vi "MC_8_10_12a_PD.vi"() -> ()   [LabVIEW 2011]
uses:
  <vilib>/Utility/file.llb/Read From Spreadsheet File (string).vi
  <vilib>/Utility/inputDevices.llb/keyboardAcquire.vi
  <vilib>/Utility/file.llb/Write To Spreadsheet File (DBL).vi
  <vilib>/Utility/file.llb/Write To Spreadsheet File (string).vi
  <vilib>/regexp/Match Regular Expression.xnode
panel:
  out "Opj X Axis":string
  in  "Room Temp":dbl=294.0
  out "No Image 2":path=path "\\\\acad1\\physics/Jurchescu-group/JW-PD/Image Not Found.png"
  out "Save1 Array":string[][](array[string])
  out "Lin Vd":dbl
  out "Lin-Vg Array-Used":dbl[](array[numeric])
  out "Lin Id-Used":dbl[](array[numeric])
  out "Comments":string
  out "Folder Index":dbl caption="Length"
  out "Current \nRecord":string[](array[string])
  out "Transformer \nHeaders":string[](array[string])
  out "Current Device ID":string
  out "Column":string
  out "Row":string
  out "Rec: Concentration":dbl
  out "Rec: Solvent":string
  out "Rec: Method":string
  in  "?":T1(tab)
  in  "Transport File":path
  out "Transport Folder":path
  out "Rec: Material":string
  in  "Treatment Concentration (mM):":dbl=nan
  in  "Surface Treatment:":string="NaN"
  in  "# Drops*:":dbl=inf
  in  "Solution Temp (C):":dbl=nan
  in  "Relative Humidity (%):":dbl=nan
  in  "Room Temp (F):":dbl=nan
  in  "Time (s):":dbl=nan
  out "Accel (RPM/s):":dbl
  in  "RPM:":dbl=nan
  in  "Wait Time (s):":dbl=nan
  in  "Sample #:":dbl=1.0
  in  "Fabricator:":string="NaN"
  in  "Transfer File":path
  out "Transfer Folder":path
  in  "Image Folder":path
  out "Image File":path=path "D:/UserData/Desktop/Jeremy/WFU/Research/Programs/VI mods/Image Not Found.png"
  in  "Ramp (s):":dbl=3.0
  out "Calc: On/Off":dbl caption="On/Off-Sat" format="%#.2e"
  out "Calc: Off I-Sat":dbl caption="Off I-Sat" format="%#.2e"
  in  "Manuel-Dielectric":bool
  in  "Manuel-Length":bool
  out "Calc: VT-Lin":dbl
  out "New: VT-Lin":dbl
  out "Rec: VT-Lin":dbl caption="VT-Lin" format="%#_3g"
  out "Calc: Trap Density-STS":dbl format="%#.2e"
  out "New: Trap Density-STS":dbl format="%#.2e"
  out "Rec: Trap Density-STS":dbl caption="N-Sat (STS)" format="%#.2e"
  out "Calc: Trap Density-VT":dbl format="%#.2e"
  out "New: Trap Density-VT":dbl format="%#.2e"
  out "Rec: Trap Density-VT":dbl caption="N-Sat (VT)" format="%#.2e"
  out "Calc: Mobility-Lin":dbl format="%#.2e"
  out "New: Mobility-Lin":dbl format="%#_4e"
  out "Rec: Mobility-Lin":dbl caption="Mobility-Lin" format="%#_3e"
  out "Calc: Mobility-Sat":dbl format="%#.2e"
  out "Rec: Length":dbl caption="Length" format="%#_3g"
  out "Rec: Width":dbl caption="Width" format="%#_4g"
  out "Rec: Dielectric (d)":dbl caption="Dielectric (d)" format="%#_3g"
  in  "Cancel Button":bool
  in  "Up Button":bool
  in  "Down Button":bool
  out "Data Name:":string
  in  "Save Changes?":bool
  in  "New: Dielectric":dbl
  in  "New: Length":dbl
  in  "New: Width":dbl
  out "New: Mobility-Sat":dbl format="%#.2e"
  in  "Blank Button":bool
  in  "Zoom":i16(slide)=-3 scale=-5.0..5.0
  out "Image Out 2":T2(plugin-control)
  out "Image Out":T2(plugin-control)
  in  "Magnification":u16(ring) items=["5x", "10x", "20x", "50x", "80x"]
  out "Total Width":dbl
  out "Distances":dbl[](array[numeric])
  in  "Undo Button":bool
  in  "Remove Button":bool
  out "Rec: Mobility-Sat":dbl caption="Mobility-Sat" format="%#.2e"
  out "Index":string
  out "Image Name":string
  in  "Export":bool
  out "Calc: VT-Sat":dbl format="%#.2g"
  out "New: VT-Sat":dbl format="%#.2g"
  in  "Manual-Width":bool caption="Manual"
  out "Calc: STS":dbl format="%#.2g"
  out "New: STS":dbl format="%#.2g"
  out "Rec: VT-Sat":dbl caption="VT-Sat" format="%#.2g"
  out "Rec: STS":dbl caption="STS-Sat" format="%#.2g"
  out "Rec: On/Off":dbl caption="On/Off-Sat" format="%#.2e"
  in  "Save Changes? 2":bool
  in  "Save Changes? 3":bool
  out "Date Recorded":string="Date Recorded" caption="Measured"
  out "Date Created":string caption="Fabricated"
  out "Rec: Temp":dbl caption="Sample Temp" format="%.1f"
  in  "New: Temp":dbl format="%.1f"
  out "Rec: Off I-Sat":dbl caption="Off I-Sat" format="%#.2e"
  in  "Independant Variable":string(combo)="Length (um):"
  in  "Transfer Plots":enum32{"Linear", "Saturation"}(tab)=enum."Saturation"
  out "XY Graph-Lin":cluster{dbl[], dbl[]}[](graph)
  in  "Slide":dbl(slide) step=1.0 scale=-22.0..89.0 scale format="%#_1p"
  out "XY Graph":cluster{dbl[], dbl[]}[](graph)
  in  "Previous Button":bool
  in  "Next Button":bool
  in  "NumPts":dbl=5.0
  in  "Log Plots":enum32{"Linear", "Saturation"}(tab)=enum."Saturation"
  in  "Slide 2":dbl(slide) step=1.0 scale=-1.0..82.0 scale format="%#_1p"
  out "XY Graph 2":cluster{dbl[], dbl[]}[](graph)
  in  "Previous Button 2":bool
  in  "Next Button 2":bool
  in  "NumPts 2":dbl=5.0 caption="NumPts"
  in  "Manual-Temp":bool caption="Manual"
  in  "Origin Project File":path=path "\\\\acad1\\physics/Jurchescu-group/JW-PD/Group Library/Origin Project Files/DeviceData_8_10_12a_JW.opj"
  in  "No Image File":path=path "\\\\acad1\\physics/Jurchescu-group/JW-PD/Mega Awesome/Image Not Found.png"
  out "String":string
  out "Index 2":dbl
  out "Sat Id-Log-Used":dbl[](array[numeric])
  out "Vg Array-Log-Used":dbl[](array[numeric])
  out "ROI Descriptor out":T3 {"Contours"."Type" items=["No Selection", "Point", "Line", "Rectangle", "Oval", "Polygon", "Freehand Region", "Annulus", "Unused2", "Unused3", "Broken Line", "Freehand Line", "Rotated Rectangle"]}
  out "ROI Descriptor":T3 {"Contours"."Type" items=["No Selection", "Point", "Line", "Rectangle", "Oval", "Polygon", "Freehand Region", "Annulus", "Unused2", "Unused3", "Broken Line", "Freehand Line", "Rotated Rectangle"]}
  out "Numeric 3":dbl
  out "Array 6":dbl[][](array[numeric])
  out "Cluster":T4
  out "Array 5":dbl[](array[numeric])
  out "Array 4":dbl[](array[numeric])
  out "Array 3":dbl[](array[numeric])
  out "Numeric 2":dbl
  out "Numeric":dbl
  out "Sat Id-Used":dbl[](array[numeric])
  out "Sat Vg Array-Used":dbl[](array[numeric])
  out "MobVi Index":dbl
  in  "Row Start":dbl=20.0
  # "Data Locations"
  # "Transport Location"
  # "Transfer Location"
  # "Image Location"
  # "Sample Properties"
  # "*     Inf = Full coverage\n   NaN = Unknown or Not Applicable"
  # "Recorded"
  # "Calculated"
  # "Re-Calculated"
  # "Manual"
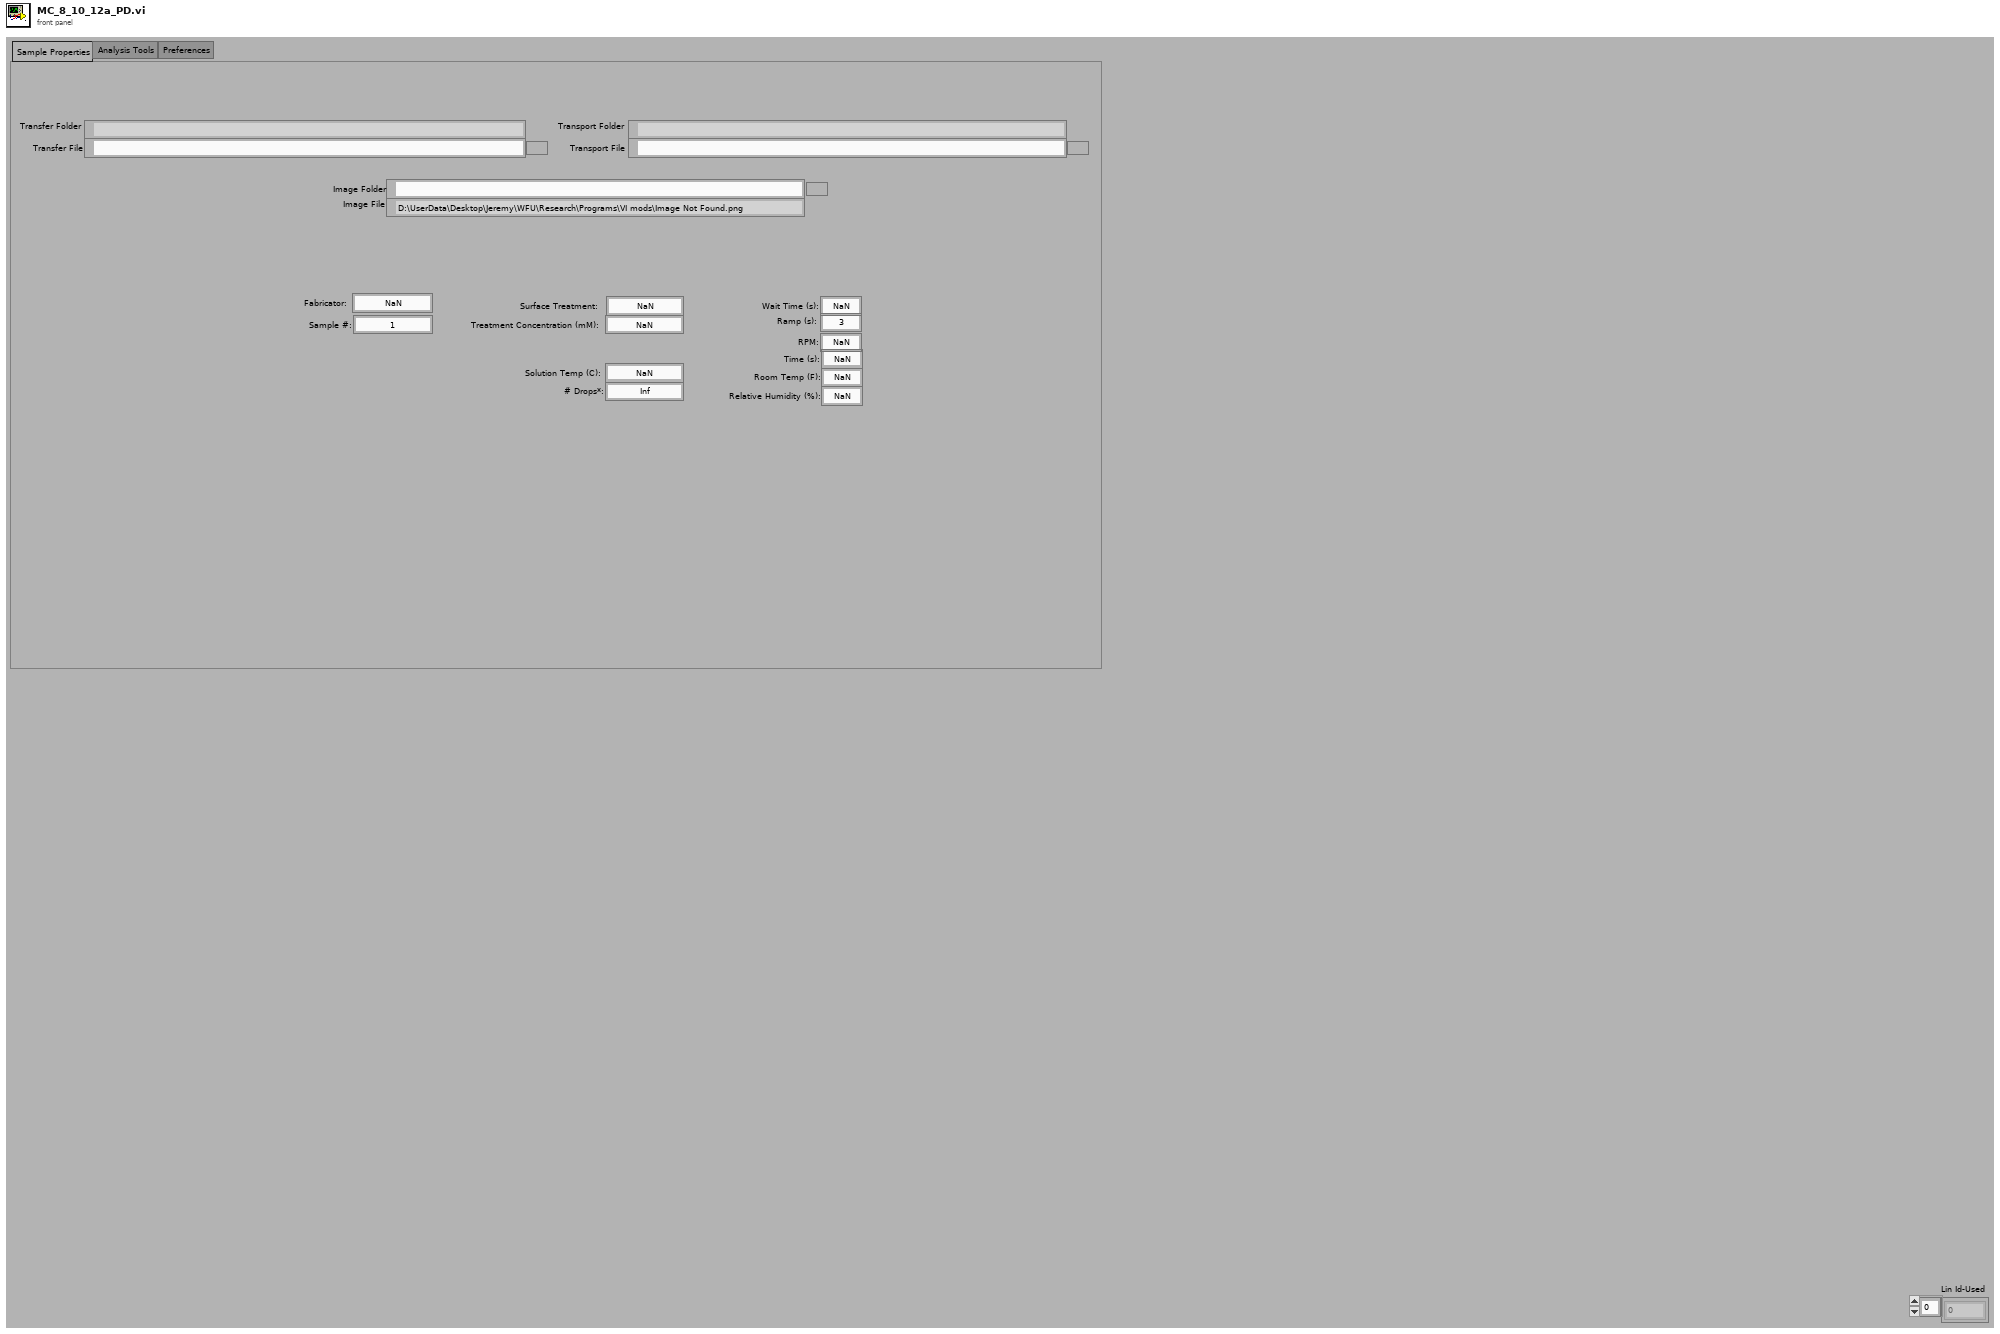
[diagram p1: front panel]
types:
  T1 = enum32{"Sample Properties", "Analysis Tools", "Preferences", "Current Database"}
  T2 = typedef "IMAQ Image.ctl" = refnum<image>
  T3 = typedef "ROI Descriptor" = cluster{"Global Rectangle":i32[], "Contours":cluster{"ID":enum32{"External", "Internal"}, "Type":u32, "Coordinates":i32[]}[]}
  T4 = cluster{"Numeric":dbl, "Numeric 2":dbl, "Numeric 3":dbl, "Numeric 4":dbl}
  T5 = cluster{"Mobility-Sat":dbl, "Moblitity-Lin":dbl, "On/Off":dbl, "Off Current":dbl, "Vt-Sat":dbl, "STS":dbl, "Trap Density-VT":dbl, "Trap Density-STS":dbl}
  T6 = cluster{"Date Recorded":string, "Index":string, "Length":dbl, "Width":dbl, "Sample Temp":dbl}
  T7 = cluster{"Date Created":string, "Material":string, "Solvent":string, "Concentration":dbl, "Method":string, "Dielectric (nm)":dbl, "Treatment":string, "Comments":string}
  T8 = cluster{"Mobility-Sat":dbl, "Vt-Sat":dbl, "Mobility-Lin":dbl, "Vt-Lin":dbl, "Off I-Sat":dbl, "On/Off I-Sat":dbl}
  T9 = cluster{"[0]":cluster{dbl[], dbl[]}, "[1]":cluster{dbl[], dbl[]}, "[2]":cluster{dbl[], dbl[]}, "[3]":cluster{dbl[], dbl[]}, "[4]":cluster{dbl[], dbl[]}, "[5]":cluster{dbl[], dbl[]}, "[6]":cluster{dbl[], dbl[]}, "[7]":cluster{dbl[], dbl[]}, "[8]":cluster{dbl[], dbl[]}}
  T10 = cluster{"Global Rectangle":i32[], "Contours":cluster{"Contour Type":u32, "ROI Type":u32, "Points":i32[]}[]}
  T11 = typedef "LVBoundsTypeDef.ctl" = cluster{"Width":u32, "Height":u32}
  T12 = enum16{"0", "1", "2", "3", "4", "5", "6", "7", "8", "9", "A", "B", "C", "D", "E", "F", "G", "H", "I", "J", "K", "L", "M", "N", "O", "P", "Q", "R", "S", "T", "U", "V", "W", "X", "Y", "Z", "F1", "F2", "F3", "F4", "F5", "F6", "F7", "F8", "F9", "F10", "F11", "F12", "F13", "F14", "F15", "ADD", "BACK", "BACKSLASH", "CAPITAL", "COMMA", "DECIMAL", "DELETE", "DIVIDE", "DOWN", "END", "EQUALS", "ESCAPE", "GRAVE (`)", "HOME", "INSERT", "LBRACKET", "LCONTROL", "LEFT", "L ALT", "LSHIFT", "LWIN", "MINUS", "MULTIPLY", "NEXT", "NUMLOCK", "NUMPAD_0", "NUMPAD_1", "NUMPAD_2", "NUMPAD_3", "NUMPAD_4", "NUMPAD_5", "NUMPAD_6", "NUMPAD_7", "NUMPAD_8", "NUMPAD_9", "PAUSE", "PERIOD", "PRIOR (PG UP)", "RBRACKET", "RCONTROL", "RETURN", "RIGHT", "R ALT", "RSHIFT", "RWIN", "SCROLL", "SEMICOLON", "SLASH", "SPACE", "SUBTRACT", "TAB", "UP", "ENTER (num pad)", "' (quote)"}[]
  T13 = enum16{"0", "1", "2", "3", "4", "5", "6", "7", "8", "9", "A", "B", "C", "D", "E", "F", "G", "H", "I", "J", "K", "L", "M", "N", "O", "P", "Q", "R", "S", "T", "U", "V", "W", "X", "Y", "Z", "F1", "F2", "F3", "F4", "F5", "F6", "F7", "F8", "F9", "F10", "F11", "F12", "F13", "F14", "F15", "ADD", "BACK", "BACKSLASH", "CAPITAL", "COMMA", "DECIMAL", "DELETE", "DIVIDE", "DOWN", "END", "EQUALS", "ESCAPE", "GRAVE (`)", "HOME", "INSERT", "LBRACKET", "LCONTROL", "LEFT", "L ALT", "LSHIFT", "LWIN", "MINUS", "MULTIPLY", "NEXT", "NUMLOCK", "NUMPAD_0", "NUMPAD_1", "NUMPAD_2", "NUMPAD_3", "NUMPAD_4", "NUMPAD_5", "NUMPAD_6", "NUMPAD_7", "NUMPAD_8", "NUMPAD_9", "PAUSE", "PERIOD", "PRIOR (PG UP)", "RBRACKET", "RCONTROL", "RETURN", "RIGHT", "R ALT", "RSHIFT", "RWIN", "SCROLL", "SEMICOLON", "SLASH", "SPACE", "SUBTRACT", "TAB", "UP", "ENTER (num pad)", "' (quote)"}
  T14 = cluster{"Contour Type":u32, "ROI Type":u32, "Points":i32[]}[]
  T15 = cluster{i32[], cluster{"Contour Type":u32, "ROI Type":u32, "Points":i32[]}[]}
  T16 = cluster{"Independant  Variable Indicator":string, "Parameter String Indicator":string}
  T17 = cluster{string, sgl, bool, bool, bool, bool, bool, bool, i32}
  T18 = cluster{i32, cluster{string, sgl, bool, bool, bool, bool, bool, bool, i32}, i32, i32}
  T19 = cluster{"Contour Type":u32, "ROI Type":u32, "Points":i32[]}
  T20 = cluster{"Points[0]":i32, "Points[1]":i32, "Points[2]":i32, "Points[3]":i32, "Points[4]":i32, "Points[5]":i32, "Points[6]":i32, "Points[7]":i32, "Points[8]":i32}
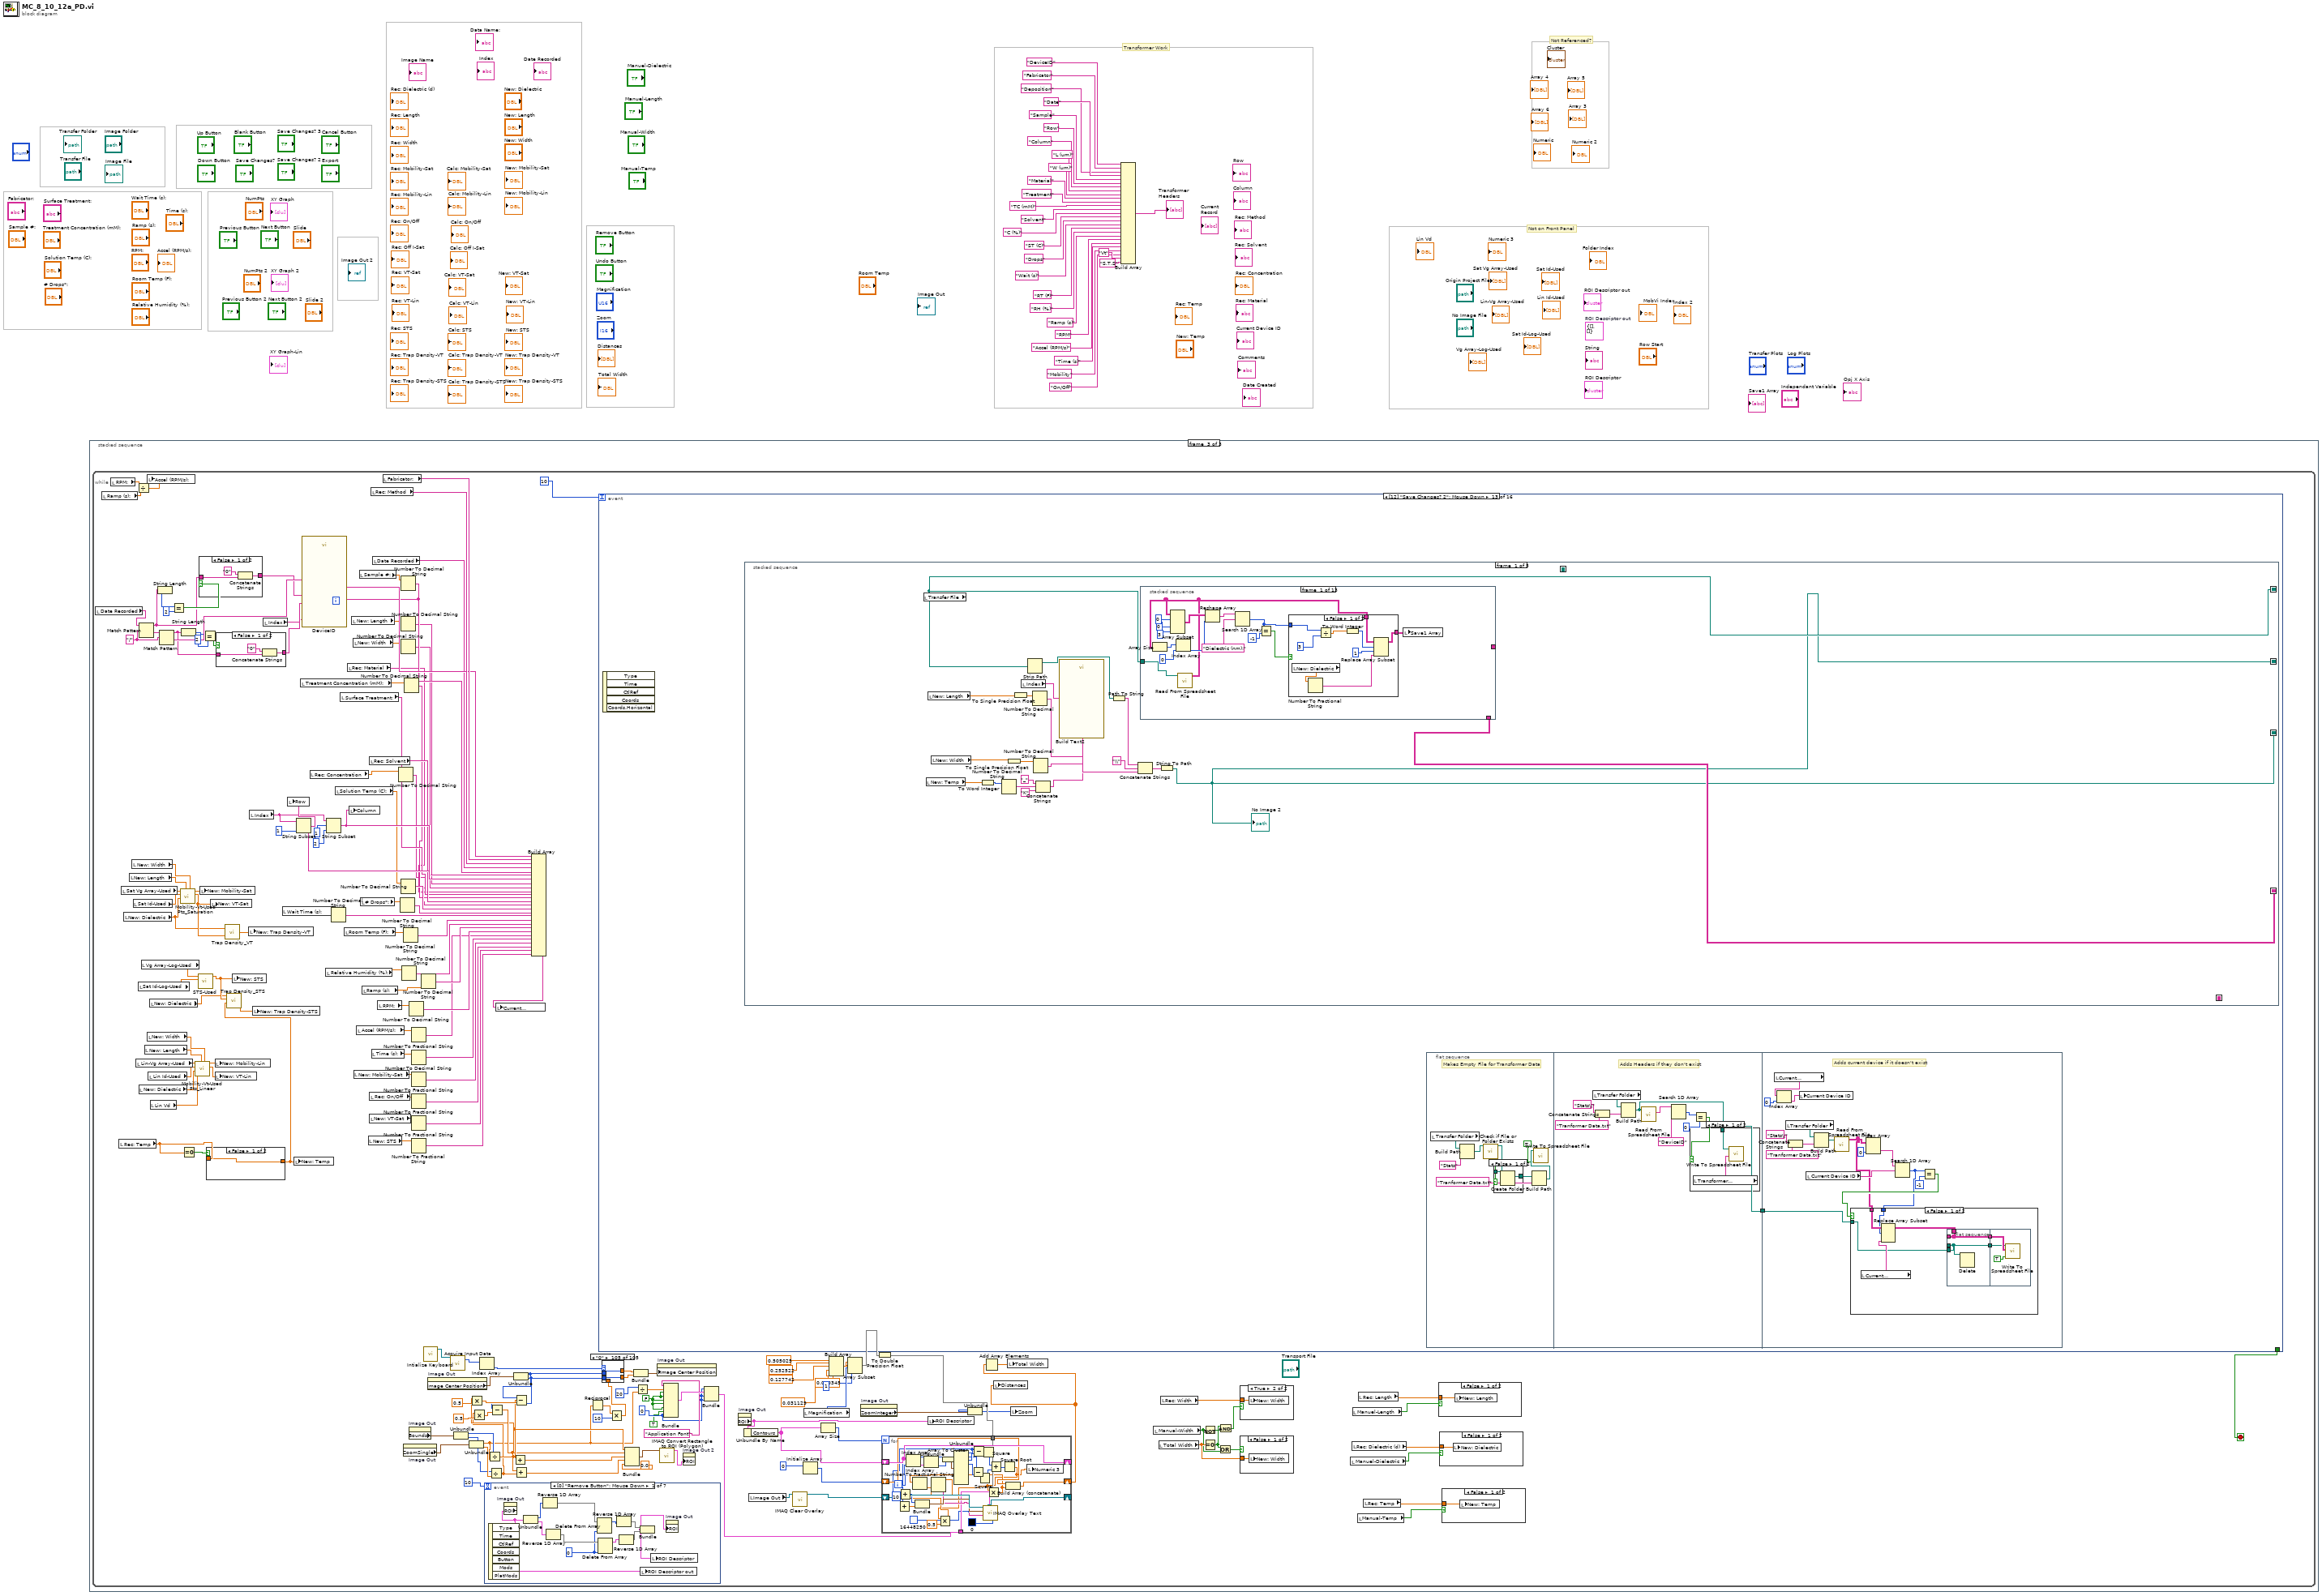
[diagram p0: block diagram]
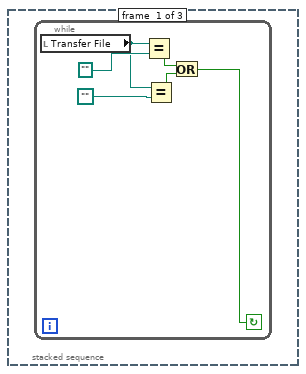
[diagram p2: hidden frame]
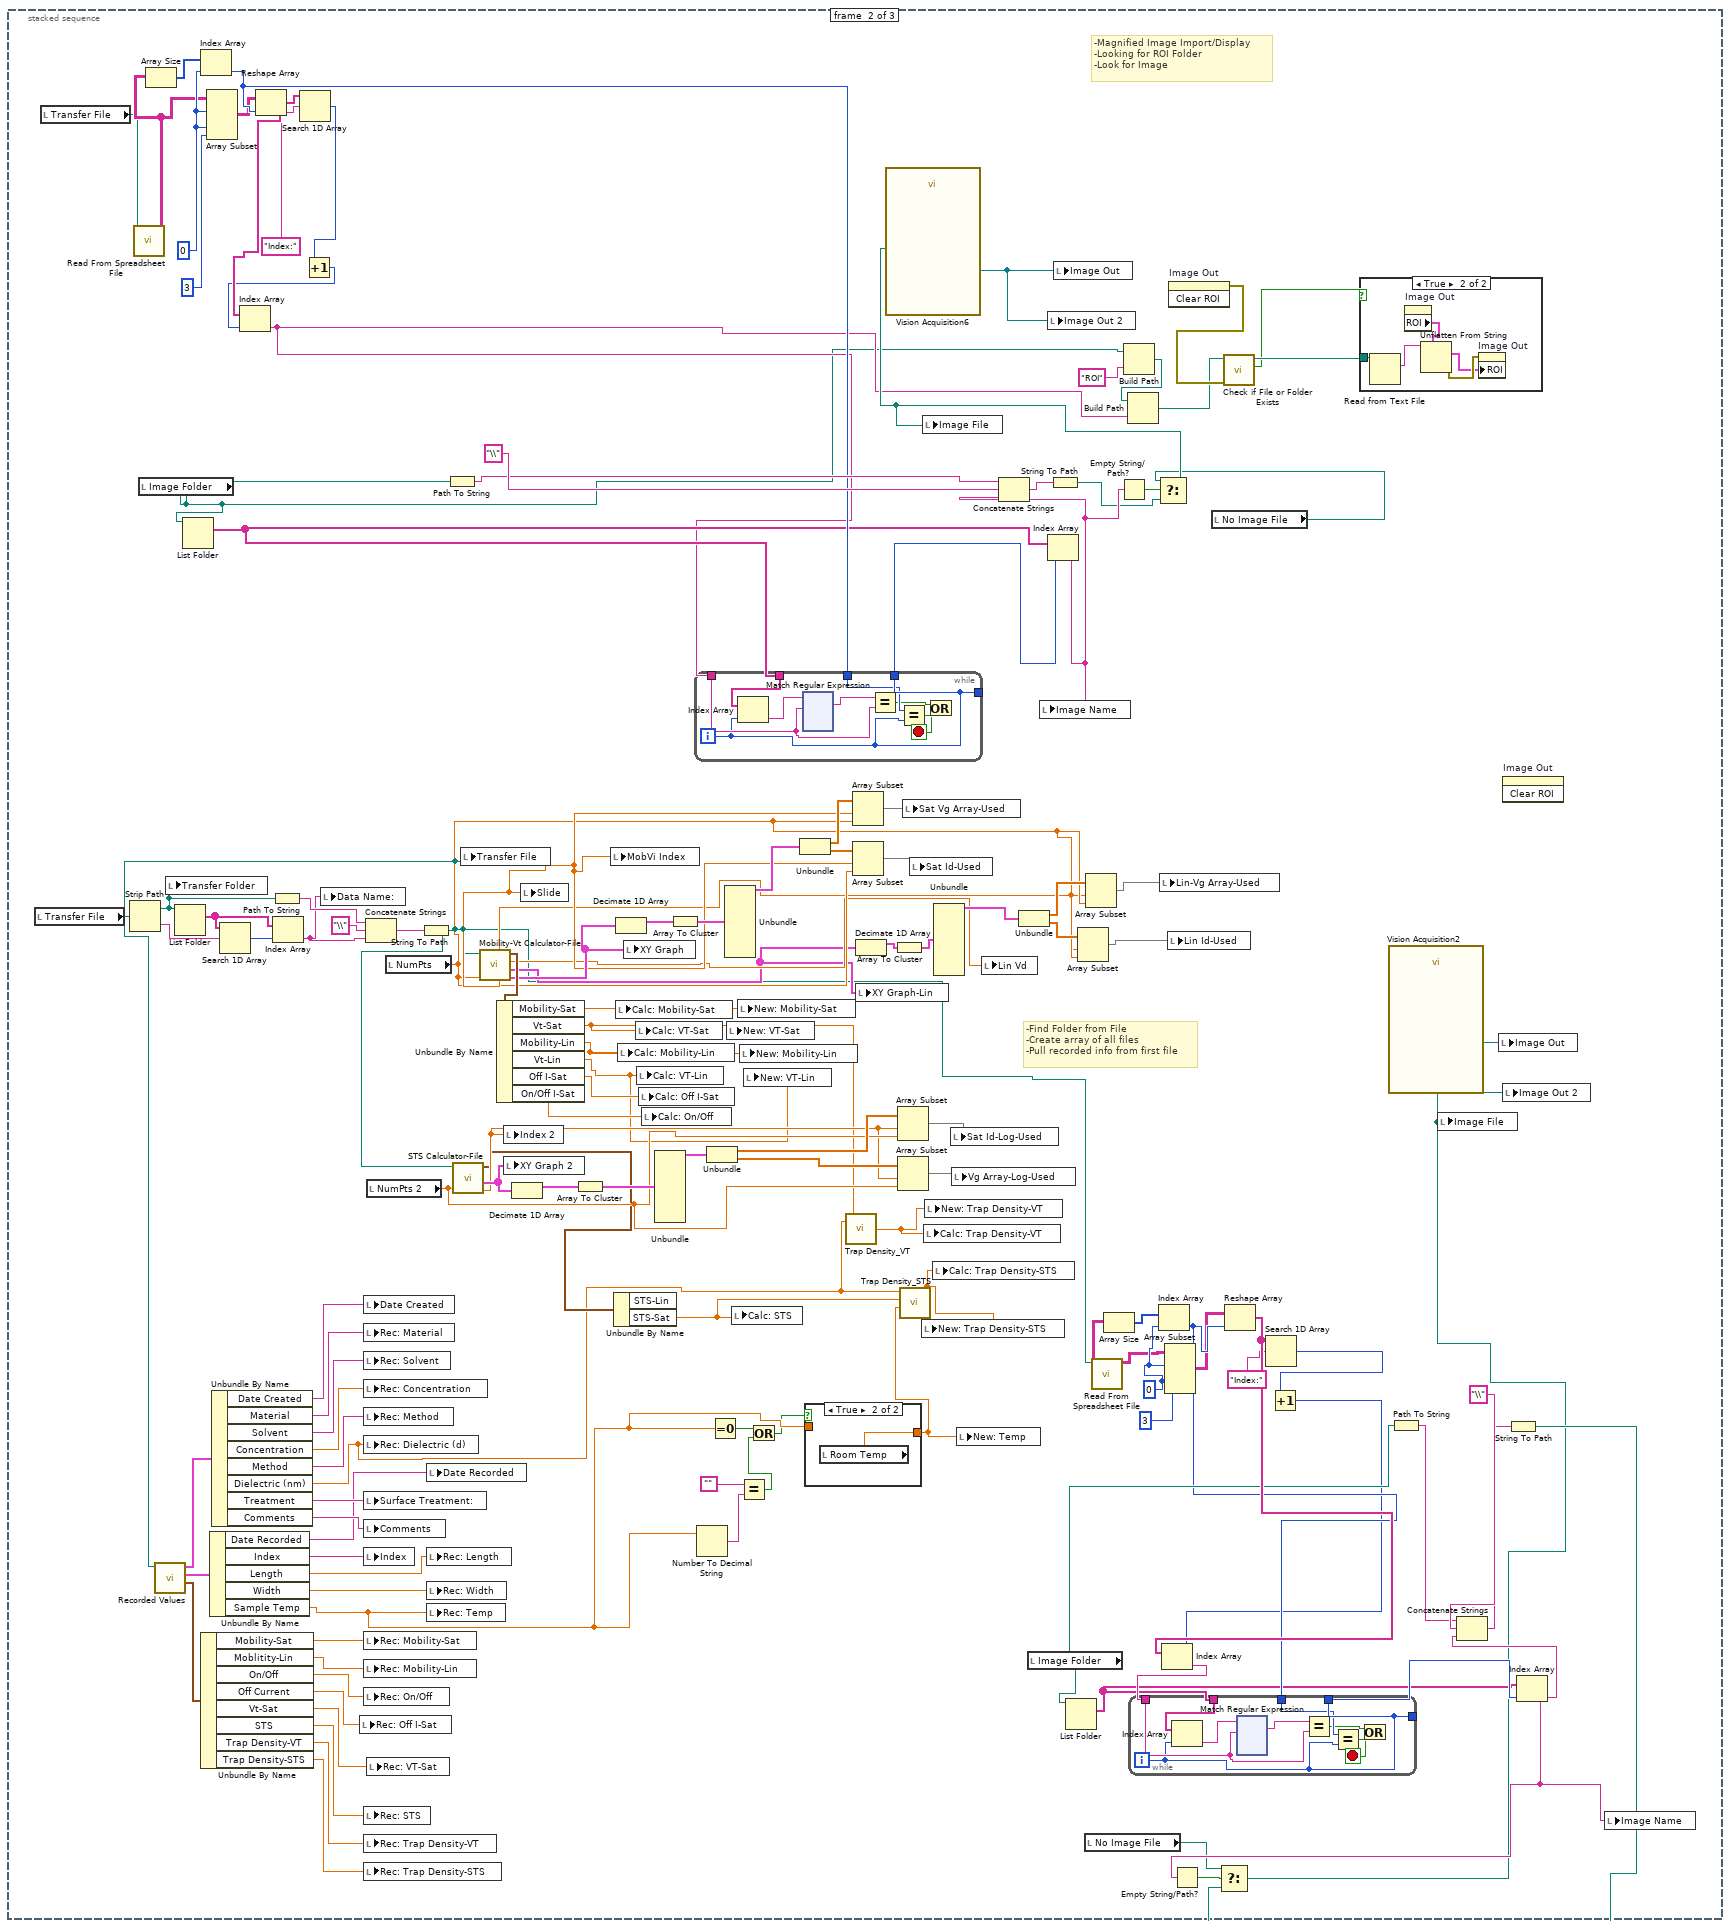
[diagram p3: hidden frame]
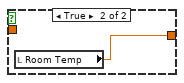
[diagram p7: hidden frame]
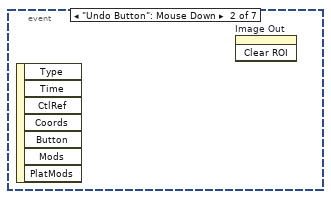
[diagram p14: hidden frame]
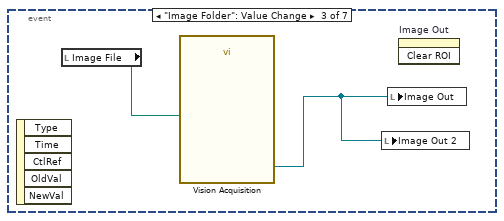
[diagram p15: hidden frame]
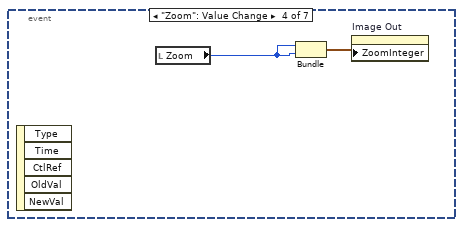
[diagram p16: hidden frame]
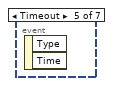
[diagram p17: hidden frame]
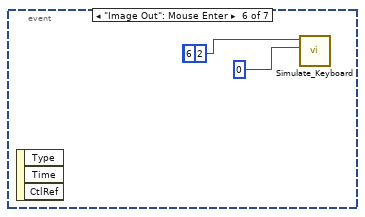
[diagram p18: hidden frame]
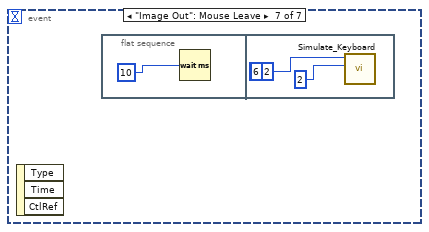
[diagram p19: hidden frame]
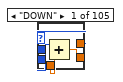
[diagram p20: hidden frame]
diagram:
  (unwired) T3 {"Global Rectangle"=[], "Contours"=[]}  # ROI Descriptor out
  # "Not Referenced?"
  # "Transformer Work"
  # "Not on Front Panel"
  n1 = stacked-sequence {
    frame #0 {
      n2 = while {
        stop <- w29 continue-if-true
        n3 = local read "Transfer File"() -> (w31:path)
        n4 = Equal?(x=w31, y=path "") -> (x = y?=w33:bool)
        n5 = Equal?(x=w31, y=path "") -> (x = y?=w32:bool)
        n6 = Or(x=w33, y=w32) -> (x .or. y?=w29:bool)
      }
    }
    frame #1 {
      w133 = 0
      w157 = 0
      # "-Find Folder from File\n-Create array of all files\n-Pull recorded info from first file"
      # "-Magnified Image Import/Display\n-Looking for ROI Folder\n-Look for Image"
      n7 = local read "Transfer File"() -> (w137:path)
      n8 = local read "Transfer File"() -> (w152:path)
      n9 = Strip Path(path=w137) -> (stripped path=w138:path, name=w124:string)
      n10 = call-poly <vilib>:"Read From Spreadsheet File.vi"("file path (dialog if empty)"=w152) -> ("all rows"=w155:string[][])  [unwired: 6 in, 4 out]
      n11 = local read "Image Folder"() -> (w94:path)
      n12 = Array Size(array=w155) -> (size(s)=w156:i32[])
      n13 = local write "Transfer Folder"(w138) -> ()
      n14 = List Folder(path=w138) -> (filenames=w128:string[])  [unwired: 3 in, 3 out]
      n15 = List Folder(path=w94) -> (filenames=w161:string[])  [unwired: 3 in, 3 out]
      n16 = Index Array(array=w156, index=w157) -> (element=w163:i32)
      n17 = Array Subset(array=w155, index (row)=w157, index (col)=w157, length (col)=3) -> (w154:string[][])  [unwired: 1 in]
      n18 = Search 1D Array(1D array=w128, element=w124) -> (index of element=w127:i32)  [unwired: 1 in]
      n19 = Reshape Array(w154, w163) -> (w168:string[])
      n20 = Path To String(path=w138) -> (string=w123:string)
      n21 = Index Array(array=w128, index=w127) -> (element=w93:string)
      n22 = Search 1D Array(1D array=w168, element="Index:") -> (index of element=w160:i32)  [unwired: 1 in]
      n23 = Increment(x=w160) -> (x+1=w159:i32)
      n24 = Index Array(array=w168, index=w159) -> (element=w95:string)
      n25 = local write "Data Name:"(w93) -> ()
      n26 = Concatenate Strings(w123, "\\", w93) -> (w125:string)
      n27 = local read "NumPts 2"() -> (w68:dbl)
      n28 = local read "NumPts"() -> (w59:dbl)
      n29 = String To Path(string=w125) -> (path=w52:path)
      n30 = call "Recorded Values.vi"("Path"=w52) -> ("Recorded Char"=w91:T5, "Recorded Prop"=w90:T6, "Fabrication Prop"=w92:T7)  [unwired: 8 in]
      n31 = Unbundle By Name(w91) -> ("Mobility-Sat"=w79:dbl, "Moblitity-Lin"=w78:dbl, "On/Off"=w77:dbl, "Off Current"=w76:dbl, "Vt-Sat"=w38:dbl, "STS"=w75:dbl, "Trap Density-VT"=w74:dbl, "Trap Density-STS"=w73:dbl)
      n32 = Unbundle By Name(w90) -> ("Date Recorded"=w83:string, "Index"=w82:string, "Length"=w81:dbl, "Width"=w80:dbl, "Sample Temp"=w44:dbl)
      n33 = Unbundle By Name(w92) -> ("Date Created"=w72:string, "Material"=w89:string, "Solvent"=w88:string, "Concentration"=w87:dbl, "Method"=w86:string, "Dielectric (nm)"=w48:dbl, "Treatment"=w85:string, "Comments"=w84:string)
      n34 = local write "Rec: Off I-Sat"(w76) -> ()
      n35 = local write "Date Created"(w72) -> ()
      n36 = local write "Rec: Material"(w89) -> ()
      n37 = local write "Rec: Solvent"(w88) -> ()
      n38 = local write "Rec: Concentration"(w87) -> ()
      n39 = local write "Rec: Method"(w86) -> ()
      n40 = local write "Rec: Dielectric (d)"(w48) -> ()
      n41 = local write "Surface Treatment:"(w85) -> ()
      n42 = local write "Comments"(w84) -> ()
      n43 = local write "Index"(w82) -> ()
      n44 = local write "Rec: Mobility-Sat"(w79) -> ()
      n45 = local write "Rec: Mobility-Lin"(w78) -> ()
      n46 = local write "Rec: On/Off"(w77) -> ()
      n47 = local write "Rec: STS"(w75) -> ()
      n48 = local write "Rec: Trap Density-VT"(w74) -> ()
      n49 = local write "Rec: Trap Density-STS"(w73) -> ()
      n50 = local write "Rec: VT-Sat"(w38) -> ()
      n51 = local write "Date Recorded"(w83) -> ()
      n52 = local write "Rec: Length"(w81) -> ()
      n53 = local write "Rec: Width"(w80) -> ()
      n54 = local write "Rec: Temp"(w44) -> ()
      n55 = Path To String(path=w94) -> (string=w165:string)
      n56 = call "STS Calculator-File.vi"("NumPts"=w68, "Path"=w52) -> ("STS Index-Sat"=w66:dbl, "XY Graph-Sat"=w67:cluster{dbl[], dbl[]}[], "Ouput"=w65:cluster{"STS-Sat":dbl, "STS-Lin":dbl})  [unwired: 5 in, 2 out]
      n57 = local write "Transfer File"(w52) -> ()
      n58 = call "Mobility-Vt Calculator-File.vi"("NumPts"=w59, "Path"=w52) -> ("XY Graph-Sat"=w70:cluster{dbl[], dbl[]}[], "XY Graph-Lin"=w54:cluster{dbl[], dbl[]}[], "Lin Vd"=w55:dbl, "Output"=w71:T8, "Index-Sat"=w69:dbl, "Index-Lin"=w58:dbl)  [unwired: 4 in]
      n59 = Unbundle By Name(w71) -> ("Mobility-Sat"=w47:dbl, "Vt-Sat"=w46:dbl, "Mobility-Lin"=w37:dbl, "Vt-Lin"=w35:dbl, "Off I-Sat"=w53:dbl, "On/Off I-Sat"=w36:dbl)
      n60 = local write "Index 2"(w66) -> ()
      n61 = local write "XY Graph 2"(w67) -> ()
      n62 = Decimate 1D Array(w67) -> (w115:cluster{dbl[], dbl[]}[])  [unwired: 1 out]
      n63 = local write "Slide"(w69) -> ()
      n64 = Array To Cluster(array=w115) -> (cluster=w117:T9)
      n65 = local write "MobVi Index"(w69) -> ()
      n66 = Unbundle By Name(w65) -> ("STS-Sat"=w51:dbl)  [unwired: 1 out]
      n67 = Decimate 1D Array(w70) -> (w151:cluster{dbl[], dbl[]}[])  [unwired: 1 out]
      n68 = local write "Calc: Mobility-Sat"(w47) -> ()
      n69 = local write "Calc: Mobility-Lin"(w37) -> ()
      n70 = local write "XY Graph"(w70) -> ()
      n71 = local write "Calc: VT-Sat"(w46) -> ()
      n72 = local write "Calc: VT-Lin"(w35) -> ()
      n73 = local write "Calc: Off I-Sat"(w53) -> ()
      n74 = local write "Calc: On/Off"(w36) -> ()
      n75 = Unbundle(w117) -> ("[0]"=w116:cluster{dbl[], dbl[]})  [unwired: 8 out]
      n76 = Array To Cluster(array=w151) -> (cluster=w149:T9)
      n77 = while {
        tunnel: w161 -> [w303]
        tunnel: w95 -> [w301]
        tunnel: [w300] -> _
        tunnel: [w300] -> w162
        tunnel: w163 -> [w299]
        i -> [w300]
        stop <- w296 stop-if-true
        n78 = Index Array(array=w303, index=w300) -> (element=w304:string)
        n79 = xnode "Match Regular Expression"("input string"=w304, "regular expression"=w301) -> ("whole match"=w302:string)  [unwired: 4 in, 4 out]
        n80 = Equal?(x=w302, y=w301) -> (x = y?=w298:bool)
        n81 = Equal?(x=w299, y=w300) -> (x = y?=w297:bool)
        n82 = Or(x=w298, y=w297) -> (x .or. y?=w296:bool)
      }
      n83 = Number To Decimal String(number=w44) -> (decimal integer string=w42:string)  [unwired: 1 in]
      n84 = Unbundle(w116) -> (w113:dbl[], w112:dbl[])
      n85 = Equal To 0?(x=w44) -> (x = 0?=w43:bool)
      n86 = Unbundle(w149) -> ("[0]"=w150:cluster{dbl[], dbl[]})  [unwired: 8 out]
      n87 = local write "New: VT-Sat"(w46) -> ()
      n88 = local write "Calc: STS"(w51) -> ()
      n89 = local write "New: Mobility-Sat"(w47) -> ()
      n90 = Equal?(x="", y=w42) -> (x = y?=w40:bool)
      n91 = local write "New: Mobility-Lin"(w37) -> ()
      n92 = local write "New: VT-Lin"(w35) -> ()
      n93 = Or(x=w43, y=w40) -> (x .or. y?=w39:bool)
      n94 = Unbundle(w150) -> (w114:dbl[], w118:dbl[])
      n95 = case shown="True" w39 {
        tunnel: [w169 w170] -> w50
        tunnel: w44 -> [w169 _]
        frame False {
        }
        frame True {
          n96 = local read "Room Temp"() -> (w170:dbl)
        }
      }
      n97 = call "Trap Density_VT.vi"("VT"=w46, "Dielectric"=w48) -> ("Trap Density-VT"=w45:dbl)
      n98 = Array Subset(array=w114, index=w69, length=w59) -> (w121:dbl[])
      n99 = Array Subset(array=w118, index=w69, length=w59) -> (w122:dbl[])
      n100 = Decimate 1D Array(w54) -> (w64:cluster{dbl[], dbl[]}[])  [unwired: 1 out]
      n101 = local write "XY Graph-Lin"(w54) -> ()
      n102 = Array To Cluster(array=w64) -> (cluster=w63:T9)
      n103 = Array Subset(array=w113, index=w66, length=w68) -> (w120:dbl[])
      n104 = Array Subset(array=w112, index=w66, length=w68) -> (w119:dbl[])
      n105 = call "Trap Density_STS.vi"("Temp (T) [K]"=w50, "S.T.S. (S)"=w51, "Dielectric"=w48) -> ("Trap Density (N)"=w49:dbl)  [unwired: 8 in]
      n106 = local write "Sat Vg Array-Used"(w121) -> ()
      n107 = local write "Sat Id-Used"(w122) -> ()
      n108 = local write "New: Trap Density-STS"(w49) -> ()
      n109 = local write "Calc: Trap Density-VT"(w45) -> ()
      n110 = local write "New: Trap Density-VT"(w45) -> ()
      n111 = local write "Calc: Trap Density-STS"(w49) -> ()
      n112 = Unbundle(w63) -> ("[0]"=w62:cluster{dbl[], dbl[]})  [unwired: 8 out]
      n113 = local write "Sat Id-Log-Used"(w120) -> ()
      n114 = local write "Vg Array-Log-Used"(w119) -> ()
      n115 = local write "New: Temp"(w50) -> ()
      n116 = local write "Lin Vd"(w55) -> ()
      n117 = Unbundle(w62) -> (w61:dbl[], w60:dbl[])
      n118 = local read "Image Folder"() -> (w144:path)
      n119 = Index Array(array=w161, index=w162) -> (element=w111:string)
      n120 = Concatenate Strings(w165, "\\", w111) -> (w166:string)
      n121 = local write "Image Name"(w111) -> ()
      n122 = String To Path(string=w166) -> (path=w109:path)
      n123 = List Folder(path=w144) -> (filenames=w140:string[])  [unwired: 3 in, 3 out]
      n124 = Array Subset(array=w60, index=w58, length=w59) -> (w56:dbl[])
      n125 = local read "No Image File"() -> (w103:path)
      n126 = Array Subset(array=w61, index=w58, length=w59) -> (w57:dbl[])
      n127 = call-poly <vilib>:"Read From Spreadsheet File.vi"("file path (dialog if empty)"=w52) -> ("all rows"=w131:string[][])  [unwired: 6 in, 4 out]
      n128 = Array Size(array=w131) -> (size(s)=w132:i32[])
      n129 = Empty String/Path?(string/path=w111) -> (empty?=w110:bool)
      n130 = Build Path(base path=w94, name or relative path="ROI") -> (appended path=w97:path)
      n131 = Build Path(base path=w97, name or relative path=w95) -> (appended path=w96:path)
      n132 = Index Array(array=w132, index=w133) -> (element=w143:i32)
      n133 = local write "Lin-Vg Array-Used"(w57) -> ()
      n134 = Array Subset(array=w131, index (row)=w133, index (col)=w133, length (col)=3) -> (w130:string[][])  [unwired: 1 in]
      n135 = local write "Lin Id-Used"(w56) -> ()
      n136 = invoke on="Image Out" class="ImageControl" method="Clear ROI"() -> (error out=w101:errorcluster)  [unwired: 3 in, 2 out]
      n137 = local read "No Image File"() -> (w102:path)
      n138 = Select(t=w102, s=w110, f=w109) -> (s? t:f=w108:path)
      n139 = call "Vision Acquisition6"("Image Path"=w108) -> ("Image Out"=w164:T2)  [unwired: 25 in, 1 out]
      n140 = local write "Image File"(w108) -> ()
      n141 = local write "Image Out 2"(w164) -> ()
      n142 = local write "Image Out"(w164) -> ()
      n143 = call <vilib>:"Check if File or Folder Exists.vi"("error in (no error)"=w101, "path"=w96) -> ("file or folder exists?"=w99:bool, "dup path"=w100:path)  [unwired: 7 in, 1 out]
      n144 = Reshape Array(w130, w143) -> (w148:string[])
      n145 = Search 1D Array(1D array=w148, element="Index:") -> (index of element=w136:i32)  [unwired: 1 in]
      n146 = Increment(x=w136) -> (x+1=w135:i32)
      n147 = Index Array(array=w148, index=w135) -> (element=w141:string)
      n148 = while {
        tunnel: w140 -> [w183]
        tunnel: w141 -> [w181]
        tunnel: [w180] -> _
        tunnel: [w180] -> w142
        tunnel: w143 -> [w179]
        i -> [w180]
        stop <- w176 stop-if-true
        n149 = Index Array(array=w183, index=w180) -> (element=w184:string)
        n150 = xnode "Match Regular Expression"("input string"=w184, "regular expression"=w181) -> ("whole match"=w182:string)  [unwired: 4 in, 4 out]
        n151 = Equal?(x=w182, y=w181) -> (x = y?=w178:bool)
        n152 = Equal?(x=w179, y=w180) -> (x = y?=w177:bool)
        n153 = Or(x=w178, y=w177) -> (x .or. y?=w176:bool)
      }
      n154 = case shown="True" w99 {
        tunnel: w100 -> [_ w171]
        frame False {
        }
        frame True {
          n155 = Read from Text File(file (use dialog)=w171) -> (text=w175:string)  [unwired: 3 in, 3 out]
          n156 = property on="Image Out" class="ImageControl"() -> ("ROI"=w172:T10)  [unwired: 2 in, 2 out]
          n157 = Unflatten From String(type=w172, binary string=w175) -> (value=w173:T10, error out=w174:errorcluster)  [unwired: 3 in, 1 out]
          n158 = property on="Image Out" class="ImageControl"(error in=w174, "ROI"=w173) -> ()  [unwired: 1 in, 2 out]
        }
      }
      n159 = Path To String(path=w144) -> (string=w145:string)
      n160 = invoke on="Image Out" class="ImageControl" method="Clear ROI"() -> ()  [unwired: 3 in, 3 out]
      n161 = Index Array(array=w140, index=w142) -> (element=w106:string)
      n162 = Empty String/Path?(string/path=w106) -> (empty?=w107:bool)
      n163 = Concatenate Strings(w145, "\\", w106) -> (w146:string)
      n164 = String To Path(string=w146) -> (path=w105:path)
      n165 = Select(t=w103, s=w107, f=w105) -> (s? t:f=w104:path)
      n166 = call "Vision Acquisition2"("Image Path"=w104) -> ("Image Out"=w139:T2)  [unwired: 25 in, 1 out]
      n167 = local write "Image File"(w104) -> ()
      n168 = local write "Image Out"(w139) -> ()
      n169 = local write "Image Out 2"(w139) -> ()
      n170 = local write "Image Name"(w106) -> ()
    }
    frame #2 {
      n171 = while {
        stop <- w583 stop-if-true
        w479 = "/"
        w533 = FALSE
        w531 = 0
        n172 = local read "Date Recorded"() -> (w482:string)
        n173 = local read "Ramp (s):"() -> (w449:dbl)
        n174 = local read "RPM:"() -> (w450:dbl)
        n175 = local read "Rec: Temp"() -> (w421:dbl)
        n176 = local read "Sat Vg Array-Used"() -> (w438:dbl[])
        n177 = local read "New: Dielectric"() -> (w423:dbl)
        n178 = local read "New: Length"() -> (w439:dbl)
        n179 = local read "New: Width"() -> (w441:dbl)
        n180 = local read "Sat Id-Used"() -> (w437:dbl[])
        n181 = local read "Lin-Vg Array-Used"() -> (w432:dbl[])
        n182 = Divide(x=w450, y=w449) -> (x/y=w448:dbl)
        n183 = local read "Sat Id-Log-Used"() -> (w436:dbl[])
        n184 = local read "New: Dielectric"() -> (w429:dbl)
        n185 = Match Pattern(string=w482, regular expression=w479) -> (before substring=w473:string, after substring=w480:string)  [unwired: 1 in, 2 out]
        n186 = local read "Vg Array-Log-Used"() -> (w435:dbl[])
        n187 = local read "New: Length"() -> (w431:dbl)
        n188 = local write "Accel (RPM/s):"(w448) -> ()
        n189 = local read "New: Width"() -> (w428:dbl)
        n190 = local read "Lin Id-Used"() -> (w433:dbl[])
        n191 = local read "New: Dielectric"() -> (w425:dbl)
        n192 = local read "Lin Vd"() -> (w427:dbl)
        n193 = String Length(string=w473) -> (length=w476:i32)
        n194 = Match Pattern(string=w480, regular expression=w479) -> (before substring=w467:string, after substring=w478:string)  [unwired: 1 in, 2 out]
        n195 = Equal?(x=w476, y=2) -> (x = y?=w474:bool)
        n196 = call "Mobility-Vt-Used Pts_Saturation.vi"("Width"=w441, "Length"=w439, "Dielectric (d)"=w423, "Sat Id Used"=w437, "Vg Used"=w438) -> ("Vt"=w424:dbl, "Mobility"=w440:dbl)  [unwired: 4 in, 1 out]
        n197 = String Length(string=w467) -> (length=w469:i32)
        n198 = Equal To 0?(x=w421) -> (x = 0?=w420:bool)
        n199 = call "Mobility-Vt-Used Pts_Linear.vi"("Width"=w428, "Length"=w431, "Vd"=w427, "Dielectric (d)"=w429, "Sat Id Used"=w433, "Vg Used"=w432) -> ("Vt"=w434:dbl, "Mobility"=w430:dbl)  [unwired: 3 in, 1 out]
        n200 = call "STS-Used.vi"("Id Used"=w436, "Vg-Used"=w435) -> ("STS"=w426:dbl)  [unwired: 9 in]
        n201 = case shown="False" w474 {
          tunnel: w473 -> [w594 w596]
          tunnel: [w593 w596] -> w472
          frame False {
            n202 = Concatenate Strings("0", w594) -> (w593:string)
          }
          frame True {
          }
        }
        n203 = local write "New: Mobility-Sat"(w440) -> ()
        n204 = Equal?(x=w469, y=2) -> (x = y?=w471:bool)
        n205 = case shown="False" w420 {
          tunnel: [w585 w586] -> w418
          tunnel: w421 -> [w585 _]
          frame False {
          }
          frame True {
            n206 = local read "Room Temp"() -> (w586:dbl)
          }
        }
        n207 = local write "New: VT-Sat"(w424) -> ()
        n208 = local write "New: Mobility-Lin"(w430) -> ()
        n209 = local write "New: VT-Lin"(w434) -> ()
        n210 = case shown="False" w471 {
          tunnel: w467 -> [w590 w592]
          tunnel: [w589 w592] -> w468
          frame False {
            n211 = Concatenate Strings("0", w590) -> (w589:string)
          }
          frame True {
          }
        }
        n212 = call "Trap Density_VT.vi"("VT"=w424, "Dielectric"=w423) -> ("Trap Density-VT"=w422:dbl)
        n213 = call "Trap Density_STS.vi"("Temp (T) [K]"=w418, "S.T.S. (S)"=w426, "Dielectric"=w425) -> ("Trap Density (N)"=w419:dbl)  [unwired: 8 in]
        n214 = local write "New: STS"(w426) -> ()
        n215 = local write "New: Trap Density-VT"(w422) -> ()
        n216 = local read "Index"() -> (w452:string)
        n217 = local write "New: Trap Density-STS"(w419) -> ()
        n218 = local read "Index"() -> (w466:string)
        n219 = local read "Wait Time (s):"() -> (w512:dbl)
        n220 = local write "New: Temp"(w418) -> ()
        n221 = String Subset(string=w452, length (rest)=1) -> (substring=w507:string)  [unwired: 1 in]
        n222 = local write "Row"(w507) -> ()
        n223 = local read "Treatment Concentration (mM):"() -> (w460:dbl)
        n224 = local read "Rec: Concentration"() -> (w447:dbl)
        n225 = local read "Relative Humidity (%):"() -> (w457:dbl)
        n226 = String Subset(string=w452, offset (0)=1, length (rest)=2) -> (substring=w508:string)
        n227 = Number To Decimal String(number=w512) -> (decimal integer string=w513:string)  [unwired: 1 in]
        n228 = local read "Solution Temp (C):"() -> (w501:dbl)
        n229 = local read "Surface Treatment:"() -> (w459:string)
        n230 = local read "Room Temp (F):"() -> (w505:dbl)
        n231 = local read "Rec: Material"() -> (w455:string)
        n232 = local write "Column"(w508) -> ()
        n233 = local read "New: Length"() -> (w465:dbl)
        n234 = local read "New: Width"() -> (w464:dbl)
        n235 = local read "New: Mobility-Sat"() -> (w494:dbl)
        n236 = local read "Accel (RPM/s):"() -> (w492:dbl)
        n237 = local read "Sample #:"() -> (w484:dbl)
        n238 = local read "# Drops*:"() -> (w502:dbl)
        n239 = local read "Ramp (s):"() -> (w510:dbl)
        n240 = local read "New: STS"() -> (w486:dbl)
        n241 = local read "Rec: Solvent"() -> (w461:string)
        n242 = local read "New: VT-Sat"() -> (w488:dbl)
        n243 = local read "Rec: On/Off"() -> (w490:dbl)
        n244 = local read "Rec: Method"() -> (w485:string)
        n245 = local read "Time (s):"() -> (w497:dbl)
        n246 = local read "Date Recorded"() -> (w481:string)
        n247 = local read "RPM:"() -> (w498:dbl)
        n248 = local read "Fabricator:"() -> (w506:string)
        n249 = Number To Decimal String(number=w447) -> (decimal integer string=w446:string)  [unwired: 1 in]
        n250 = Number To Decimal String(number=w502) -> (decimal integer string=w503:string)  [unwired: 1 in]
        n251 = Number To Decimal String(number=w484) -> (decimal integer string=w477:string)  [unwired: 1 in]
        n252 = call "DeviceID"("Sample"=w477, "Year"=w478, "Month"=w472, "Day"=w468, "Index"=w466) -> ("Result"=w483:string)  [unwired: 9 in, 1 out]
        n253 = Number To Decimal String(number=w465) -> (decimal integer string=w463:string)  [unwired: 1 in]
        n254 = Number To Decimal String(number=w464) -> (decimal integer string=w462:string)  [unwired: 1 in]
        n255 = Number To Decimal String(number=w501) -> (decimal integer string=w500:string)  [unwired: 1 in]
        n256 = Number To Decimal String(number=w457) -> (decimal integer string=w456:string)  [unwired: 1 in]
        n257 = Number To Decimal String(number=w505) -> (decimal integer string=w504:string)  [unwired: 1 in]
        n258 = property on="Image Out" class="ImageControl"() -> ("ZoomSingle"=w551:cluster{"X":sgl, "Y":sgl})  [unwired: 2 in, 2 out]
        n259 = Number To Decimal String(number=w460) -> (decimal integer string=w458:string)  [unwired: 1 in]
        n260 = property on="Image Out" class="ImageControl"() -> ("Bounds"=w552:T11)  [unwired: 2 in, 2 out]
        n261 = Number To Decimal String(number=w498) -> (decimal integer string=w499:string)  [unwired: 1 in]
        n262 = Number To Fractional String(number=w492) -> (F-format string=w493:string)  [unwired: 3 in]
        n263 = Number To Decimal String(number=w497) -> (decimal integer string=w496:string)  [unwired: 1 in]
        n264 = Number To Fractional String(number=w494) -> (F-format string=w495:string)  [unwired: 3 in]
        n265 = Number To Fractional String(number=w490) -> (F-format string=w491:string)  [unwired: 3 in]
        n266 = Number To Fractional String(number=w488) -> (F-format string=w489:string)  [unwired: 3 in]
        n267 = Number To Fractional String(number=w486) -> (F-format string=w487:string)  [unwired: 3 in]
        n268 = Number To Decimal String(number=w510) -> (decimal integer string=w511:string)  [unwired: 1 in]
        n269 = call <vilib>:"Intialize Keyboard.vi"() -> ("device ID"=w563:refnum<k1>)  [unwired: 10 in, 1 out]
        n270 = property on="Image Out" class="ImageControl"() -> ("Image Center Position"=w558:cluster{"X":u32, "Y":u32})  [unwired: 2 in, 2 out]
        n271 = call-poly <vilib>:"Acquire Input Data.vi"("device ID"=w563) -> ("keys pressed"=w562:T12)  [unwired: 16 in, 2 out]
        n272 = Unbundle(w552) -> ("Width"=w549:u32, "Height"=w548:u32)
        n273 = Unbundle(w551) -> ("X"=w526:sgl, "Y"=w550:sgl)
        n274 = Index Array(array=w562) -> (element=w566:T13)  [unwired: 1 in]
        n275 = event shown="[0] \"Remove Button\": Mouse Down" {
          selector: _ -> [_ _ _ _ _ _ _]
          dyn-events: _ -> [_ _ _ _ _ _ _]
          timeout: 10 -> [_ _ _ _ _ _ _]
          event "Remove Button": Mouse Down {
            w601 = 0
            n276 = event-data() -> ()  [unwired: 1 in, 7 out]
            n277 = property on="Image Out" class="ImageControl"() -> ("ROI"=w599:T10)  [unwired: 2 in, 2 out]
            n278 = Unbundle(w599) -> ("Global Rectangle"=w602:i32[], "Contours"=w604:T14)
            n279 = Reverse 1D Array(array=w602) -> (reversed array=w603:i32[])
            n280 = Reverse 1D Array(array=w604) -> (reversed array=w605:T14)
            n281 = Delete From Array(array=w603, index=w601) -> (array with subset deleted=w606:i32[])  [unwired: 1 in, 1 out]
            n282 = Delete From Array(array=w605, index=w601) -> (array with subset deleted=w607:T14)  [unwired: 1 in, 1 out]
            n283 = Reverse 1D Array(array=w606) -> (reversed array=w608:i32[])
            n284 = Reverse 1D Array(array=w607) -> (reversed array=w609:T14)
            n285 = Bundle(w608, w609) -> (w600:T15)  [unwired: 1 in]
            n286 = local write "ROI Descriptor out"(w599) -> ()
            n287 = local write "ROI Descriptor"(w600) -> ()
            n288 = property on="Image Out" class="ImageControl"("ROI"=w600) -> ()  [unwired: 2 in, 2 out]
          }
          event "Undo Button": Mouse Down {
            n289 = event-data() -> ()  [unwired: 1 in, 7 out]
            n290 = invoke on="Image Out" class="ImageControl" method="Clear ROI"() -> ()  [unwired: 3 in, 3 out]
          }
          event "Image Folder": Value Change {
            n291 = event-data() -> ()  [unwired: 1 in, 5 out]
            n292 = local read "Image File"() -> (w611:path)
            n293 = call "Vision Acquisition"("Image Path"=w611) -> ("Image Out"=w610:T2)  [unwired: 25 in, 1 out]
            n294 = local write "Image Out 2"(w610) -> ()
            n295 = local write "Image Out"(w610) -> ()
            n296 = invoke on="Image Out" class="ImageControl" method="Clear ROI"() -> ()  [unwired: 3 in, 3 out]
          }
          event "Zoom": Value Change {
            n297 = event-data() -> ()  [unwired: 1 in, 5 out]
            n298 = local read "Zoom"() -> (w612:i16)
            n299 = Bundle("Zoom"=w612, "Zoom"=w612) -> (w613:cluster{"Zoom":i16, "Zoom":i16})  [unwired: 1 in]
            n300 = property on="Image Out" class="ImageControl"("ZoomInteger"=w613) -> ()  [unwired: 2 in, 2 out]
          }
          event Timeout {
            n301 = event-data() -> ()  [unwired: 1 in, 2 out]
          }
          event "Image Out": Mouse Enter {
            (unwired) 6
            n302 = event-data() -> ()  [unwired: 1 in, 3 out]
            n303 = call "Simulate_Keyboard.vi"("Action"=0, "Virtual Key"=162) -> ()  [unwired: 7 in, 1 out]
          }
          event "Image Out": Mouse Leave {
            n304 = event-data() -> ()  [unwired: 1 in, 3 out]
            n305 = flat-sequence {
              frame #0 {
                n306 = Wait (ms)(milliseconds to wait=10) -> ()  [unwired: 1 out]
              }
              frame #1 {
                (unwired) 6
                n307 = call "Simulate_Keyboard.vi"("Action"=2, "Virtual Key"=162) -> ()  [unwired: 7 in, 1 out]
              }
            }
          }
        }
        n308 = Divide(x=w549, y=w526) -> (x/y=w539:sgl)
        n309 = Multiply(x=w539, y=0.5) -> (x*y=w545:dbl)
        n310 = Divide(x=w548, y=w550) -> (x/y=w538:sgl)
        n311 = Multiply(x=w538, y=0.5) -> (x*y=w544:dbl)
        n312 = Unbundle(w558) -> ("X"=w540:u32, "Y"=w541:u32)
        n313 = Subtract(x=w541, y=w544) -> (x-y=w542:dbl)
        n314 = Subtract(x=w540, y=w545) -> (x-y=w543:dbl)
        n315 = Add(x=w543, y=w539) -> (x+y=w557:dbl)
        n316 = Add(x=w542, y=w538) -> (x+y=w556:dbl)
        n317 = Build Array(w483, w506, w485, w481, w477, w507, w508, w463, w462, w455, w459, w458, w461, w446, w500, w503, w513, w504, w456, w511, w499, w493, w496, w495, w491, w489, w487) -> (w509:string[])
        n318 = local write "Current \nRecord"(w509) -> ()
        n319 = Reciprocal(x=w526) -> (1/x=w525:sgl)
        n320 = event shown="[12] \"Save Changes? 2\": Mouse Down" {
          selector: _ -> [_ _ _ _ _ _ _ _ _ _ _ _ _ _ _ _]
          dyn-events: _ -> [_ _ _ _ _ _ _ _ _ _ _ _ _ _ _ _]
          timeout: 10 -> [_ _ _ _ _ _ _ _ _ _ _ _ _ _ _ _]
          tunnel: [_ _ _ _ _ _ _ _ _ _ _ _ _ TRUE _ TRUE] -> w583
          event Timeout {
            n321 = event-data() -> ()  [unwired: 1 in, 2 out]
          }
          event "Down Button": Mouse Down {
            w953 = 0
            n322 = event-data() -> ()  [unwired: 1 in, 7 out]
            n323 = local read "Transfer File"() -> (w958:path)
            n324 = Strip Path(path=w958) -> (stripped path=w949:path, name=w967:string)
            n325 = local write "Transfer Folder"(w949) -> ()
            n326 = List Folder(path=w949) -> (filenames=w963:string[], error out=w903:errorcluster)  [unwired: 3 in, 2 out]
            n327 = local read "Folder Index"() -> (w905:dbl)
            n328 = Array Size(array=w963) -> (size(s)=w959:i32)
            n329 = Search 1D Array(1D array=w963, element=w967) -> (index of element=w960:i32)  [unwired: 1 in]
            n330 = property on="Image Out" class="ImageControl"() -> (error out=w906:errorcluster, "Image Center Position"=w910:cluster{"X":u32, "Y":u32})  [unwired: 2 in, 1 out]
            n331 = Decrement(x=w959) -> (x-1=w961:i32)
            n332 = Equal?(x=w960, y=w961) -> (x = y?=w962:bool)
            n333 = invoke on="Image Out" class="ImageControl" method="Clear ROI"() -> ()  [unwired: 3 in, 3 out]
            n334 = case shown="False" w962 {
              tunnel: w905 -> [w1120 _]
              tunnel: [w1119 0] -> w904
              tunnel: w903 -> [w1118 w1121]
              tunnel: [w1118 w1121] -> w902
              frame False {
                n335 = Increment(x=w1120) -> (x+1=w1119:dbl)
              }
              frame True {
              }
            }
            n336 = Unbundle(w910) -> ("X"=w908:u32)  [unwired: 1 out]
            n337 = local write "Folder Index"(w904) -> ()
            n338 = Bundle("X"=w908, 0) -> (w909:cluster{"X":u32, i32})  [unwired: 1 in]
            n339 = property on="Image Out" class="ImageControl"(error in=w906, "Image Center Position"=w909) -> ()  [unwired: 1 in, 2 out]
            n340 = Path To String(path=w949) -> (string=w968:string)
            n341 = Index Array(array=w963, index=w904) -> (element=w964:string)
            n342 = local write "Data Name:"(w964) -> ()
            n343 = Concatenate Strings(w968, "\\", w964) -> (w966:string)
            n344 = String To Path(string=w966) -> (path=w876:path)
            n345 = call "Recorded Values.vi"("Path"=w876) -> ("Recorded Char"=w970:T5, "Recorded Prop"=w971:T6, "Fabrication Prop"=w969:T7)  [unwired: 8 in]
            n346 = Unbundle By Name(w970) -> ("Mobility-Sat"=w983:dbl, "Moblitity-Lin"=w984:dbl, "On/Off"=w985:dbl, "Off Current"=w986:dbl, "Vt-Sat"=w871:dbl, "STS"=w987:dbl, "Trap Density-VT"=w988:dbl, "Trap Density-STS"=w989:dbl)
            n347 = Unbundle By Name(w969) -> ("Date Created"=w990:string, "Material"=w972:string, "Solvent"=w973:string, "Concentration"=w974:dbl, "Method"=w975:string, "Dielectric (nm)"=w976:dbl, "Treatment"=w977:string, "Comments"=w978:string)
            n348 = Unbundle By Name(w971) -> ("Date Recorded"=w979:string, "Index"=w980:string, "Length"=w981:dbl, "Width"=w982:dbl, "Sample Temp"=w873:dbl)
            n349 = local write "Date Created"(w990) -> ()
            n350 = local write "Rec: Off I-Sat"(w986) -> ()
            n351 = local write "Rec: Material"(w972) -> ()
            n352 = local write "Rec: VT-Sat"(w871) -> ()
            n353 = local write "Rec: Concentration"(w974) -> ()
            n354 = local write "Rec: Method"(w975) -> ()
            n355 = local write "Rec: Dielectric (d)"(w976) -> ()
            n356 = local write "Surface Treatment:"(w977) -> ()
            n357 = local write "Comments"(w978) -> ()
            n358 = local write "Index"(w980) -> ()
            n359 = local write "Rec: Mobility-Sat"(w983) -> ()
            n360 = local write "Rec: Mobility-Lin"(w984) -> ()
            n361 = local write "Rec: On/Off"(w985) -> ()
            n362 = local write "Rec: STS"(w987) -> ()
            n363 = local write "Rec: Trap Density-VT"(w988) -> ()
            n364 = local write "Rec: Trap Density-STS"(w989) -> ()
            n365 = local write "Rec: Solvent"(w973) -> ()
            n366 = local write "Date Recorded"(w979) -> ()
            n367 = local write "Rec: Length"(w981) -> ()
            n368 = local write "Rec: Width"(w982) -> ()
            n369 = local write "Rec: Temp"(w873) -> ()
            n370 = Equal To 0?(x=w873) -> (x = 0?=w874:bool)
            n371 = case shown="True" w874 {
              tunnel: [w991 w992] -> w872
              tunnel: w873 -> [w991 _]
              frame False {
              }
              frame True {
                n372 = local read "Room Temp"() -> (w992:dbl)
              }
            }
            n373 = local read "NumPts 2"() -> (w897:dbl)
            n374 = local write "Transfer File"(w876) -> ()
            n375 = local read "NumPts"() -> (w901:dbl)
            n376 = call-poly <vilib>:"Read From Spreadsheet File.vi"("file path (dialog if empty)"=w876) -> ("all rows"=w955:string[][])  [unwired: 6 in, 4 out]
            n377 = call "Mobility-Vt Calculator-File.vi"("NumPts"=w901, "Path"=w876) -> ("XY Graph-Sat"=w899:cluster{dbl[], dbl[]}[], "XY Graph-Lin"=w870:cluster{dbl[], dbl[]}[], "Output"=w900:T8, "Index-Sat"=w898:dbl, "Index-Lin"=w884:dbl)  [unwired: 4 in, 1 out]
            n378 = local read "New: Dielectric"() -> (w881:dbl)
            n379 = call "STS Calculator-File.vi"("NumPts"=w897, "Path"=w876) -> ("STS Index-Sat"=w896:dbl, "XY Graph-Sat"=w895:cluster{dbl[], dbl[]}[], "Ouput"=w894:cluster{"STS-Sat":dbl, "STS-Lin":dbl})  [unwired: 5 in, 2 out]
            n380 = Unbundle By Name(w900) -> ("Mobility-Sat"=w893:dbl, "Vt-Sat"=w880:dbl, "Mobility-Lin"=w892:dbl, "Vt-Lin"=w891:dbl, "Off I-Sat"=w877:dbl, "On/Off I-Sat"=w869:dbl)
            n381 = Unbundle By Name(w894) -> ("STS-Sat"=w875:dbl)  [unwired: 1 out]
            n382 = local write "Index 2"(w896) -> ()
            n383 = local write "XY Graph 2"(w895) -> ()
            n384 = local write "MobVi Index"(w898) -> ()
            n385 = local write "Slide"(w898) -> ()
            n386 = local write "XY Graph"(w899) -> ()
            n387 = Array Size(array=w955) -> (size(s)=w954:i32[])
            n388 = call "Trap Density_VT.vi"("VT"=w880, "Dielectric"=w881) -> ("Trap Density-VT"=w879:dbl)
            n389 = call "Trap Density_STS.vi"("Temp (T) [K]"=w872, "S.T.S. (S)"=w875, "Dielectric"=w881) -> ("Trap Density (N)"=w878:dbl)  [unwired: 8 in]
            n390 = local write "New: STS"(w875) -> ()
            n391 = local write "Calc: STS"(w875) -> ()
            n392 = local write "Calc: Mobility-Sat"(w893) -> ()
            n393 = local write "Calc: Off I-Sat"(w891) -> ()
            n394 = local write "Calc: Mobility-Lin"(w892) -> ()
            n395 = Index Array(array=w954, index=w953) -> (element=w935:i32)
            n396 = Decimate 1D Array(w895) -> (w929:cluster{dbl[], dbl[]}[])  [unwired: 1 out]
            n397 = Decimate 1D Array(w899) -> (w939:cluster{dbl[], dbl[]}[])  [unwired: 1 out]
            n398 = local write "Calc: Off I-Sat"(w877) -> ()
            n399 = local write "Calc: On/Off"(w869) -> ()
            n400 = Decimate 1D Array(w870) -> (w890:cluster{dbl[], dbl[]}[])  [unwired: 1 out]
            n401 = local write "Calc: VT-Sat"(w880) -> ()
            n402 = Array Subset(array=w955, index (row)=w953, index (col)=w953, length (col)=3) -> (w956:string[][])  [unwired: 1 in]
            n403 = local write "Calc: Trap Density-VT"(w879) -> ()
            n404 = local write "Calc: Trap Density-STS"(w878) -> ()
            n405 = local write "New: Trap Density-STS"(w878) -> ()
            n406 = local write "New: Trap Density-VT"(w879) -> ()
            n407 = local write "XY Graph-Lin"(w870) -> ()
            n408 = Array To Cluster(array=w929) -> (cluster=w927:T9)
            n409 = Array To Cluster(array=w939) -> (cluster=w941:T9)
            n410 = local write "New: VT-Lin"(w891) -> ()
            n411 = local write "New: VT-Sat"(w880) -> ()
            n412 = local write "New: Mobility-Sat"(w893) -> ()
            n413 = local write "New: Mobility-Lin"(w892) -> ()
            n414 = Reshape Array(w956, w935) -> (w942:string[])
            n415 = Array To Cluster(array=w890) -> (cluster=w889:T9)
            n416 = Subtract(x=w935, y=20) -> (x-y=w934:i32)
            n417 = property on="Slide" class="Slide (strict)"("Scale.Maximum"=w934) -> ()  [unwired: 2 in, 2 out]
            n418 = Unbundle(w927) -> ("[0]"=w928:cluster{dbl[], dbl[]})  [unwired: 8 out]
            n419 = Unbundle(w941) -> ("[0]"=w940:cluster{dbl[], dbl[]})  [unwired: 8 out]
            n420 = Unbundle(w889) -> ("[0]"=w886:cluster{dbl[], dbl[]})  [unwired: 8 out]
            n421 = Search 1D Array(1D array=w942, element="Index:") -> (index of element=w950:i32)  [unwired: 1 in]
            n422 = local read "NumPts"() -> (w885:dbl)
            n423 = Unbundle(w886) -> (w888:dbl[], w887:dbl[])
            n424 = Increment(x=w950) -> (x+1=w951:i32)
            n425 = Unbundle(w928) -> (w926:dbl[], w925:dbl[])
            n426 = Unbundle(w940) -> (w931:dbl[], w930:dbl[])
            n427 = Array Subset(array=w888, index=w884, length=w885) -> (w883:dbl[])
            n428 = Array Subset(array=w887, index=w884, length=w885) -> (w882:dbl[])
            n429 = Array Subset(array=w926, index=w896, length=w897) -> (w933:dbl[])
            n430 = Array Subset(array=w925, index=w896, length=w897) -> (w932:dbl[])
            n431 = Array Subset(array=w931, index=w898, length=w901) -> (w938:dbl[])
            n432 = Array Subset(array=w930, index=w898, length=w901) -> (w937:dbl[])
            n433 = Index Array(array=w942, index=w951) -> (element=w914:string)
            n434 = local write "Lin-Vg Array-Used"(w883) -> ()
            n435 = local write "Sat Vg Array-Used"(w938) -> ()
            n436 = local write "Vg Array-Log-Used"(w932) -> ()
            n437 = local write "Lin Id-Used"(w882) -> ()
            n438 = local read "Image Folder"() -> (w912:path)
            n439 = local write "Sat Id-Used"(w937) -> ()
            n440 = local write "Sat Id-Log-Used"(w933) -> ()
            n441 = List Folder(path=w912, error in=w902) -> (filenames=w948:string[], error out=w915:errorcluster)  [unwired: 2 in, 2 out]
            n442 = while {
              tunnel: w948 -> [w1005]
              tunnel: w914 -> [w1003]
              tunnel: [w1002] -> _
              tunnel: [w1002] -> w947
              tunnel: w935 -> [w1001]
              i -> [w1002]
              stop <- w998 stop-if-true
              n443 = Index Array(array=w1005, index=w1002) -> (element=w1006:string)
              n444 = xnode "Match Regular Expression"("input string"=w1006, "regular expression"=w1003) -> ("whole match"=w1004:string)  [unwired: 4 in, 4 out]
              n445 = Equal?(x=w1004, y=w1003) -> (x = y?=w1000:bool)
              n446 = Equal?(x=w1001, y=w1002) -> (x = y?=w999:bool)
              n447 = Or(x=w1000, y=w999) -> (x .or. y?=w998:bool)
            }
            n448 = Build Path(base path=w912, name or relative path="ROI") -> (appended path=w911:path)
            n449 = Path To String(path=w912) -> (string=w945:string)
            n450 = Index Array(array=w948, index=w947) -> (element=w923:string)
            n451 = invoke on="Image Out" class="ImageControl" method="Clear ROI"(error in=w915) -> (error out=w918:errorcluster)  [unwired: 2 in, 2 out]
            n452 = local write "Image Name"(w923) -> ()
            n453 = Build Path(base path=w911, name or relative path=w914) -> (appended path=w919:path)
            n454 = call <vilib>:"Check if File or Folder Exists.vi"("error in (no error)"=w918, "path"=w919) -> ("file or folder exists?"=w916:bool, "dup path"=w917:path)  [unwired: 7 in, 1 out]
            n455 = Concatenate Strings(w945, "\\", w923) -> (w944:string)
            n456 = case shown="False" w916 {
              tunnel: w917 -> [_ w993]
              frame False {
              }
              frame True {
                n457 = Read from Text File(file (use dialog)=w993) -> (text=w997:string)  [unwired: 3 in, 3 out]
                n458 = property on="Image Out" class="ImageControl"() -> ("ROI"=w994:T10)  [unwired: 2 in, 2 out]
                n459 = Unflatten From String(type=w994, binary string=w997) -> (value=w995:T10, error out=w996:errorcluster)  [unwired: 3 in, 1 out]
                n460 = property on="Image Out" class="ImageControl"(error in=w996, "ROI"=w995) -> ()  [unwired: 1 in, 2 out]
              }
            }
            n461 = String To Path(string=w944) -> (path=w922:path)
            n462 = Empty String/Path?(string/path=w923) -> (empty?=w924:bool)
            n463 = local read "No Image File"() -> (w920:path)
            n464 = Select(t=w920, s=w924, f=w922) -> (s? t:f=w921:path)
            n465 = local write "Image File"(w921) -> ()
            n466 = call "Vision Acquisition4"("Image Path"=w921) -> ("Image Out"=w946:T2)  [unwired: 25 in, 1 out]
            n467 = local write "Image Out"(w946) -> ()
            n468 = local write "Image Out 2"(w946) -> ()
          }
          event "Transfer File": Value Change {
            w1229 = 0
            n469 = event-data() -> ()  [unwired: 1 in, 5 out]
            n470 = local read "Transfer File"() -> (w1225:path)
            n471 = Strip Path(path=w1225) -> (stripped path=w1224:path, name=w1238:string)
            n472 = local write "Transfer Folder"(w1224) -> ()
            n473 = property on="Image Out" class="ImageControl"() -> (error out=w1180:errorcluster, "Image Center Position"=w1184:cluster{"X":u32, "Y":u32})  [unwired: 2 in, 1 out]
            n474 = List Folder(path=w1224) -> (filenames=w1234:string[], error out=w1190:errorcluster)  [unwired: 3 in, 2 out]
            n475 = Search 1D Array(1D array=w1234, element=w1238) -> (index of element=w1179:i32)  [unwired: 1 in]
            n476 = local write "Folder Index"(w1179) -> ()
            n477 = Unbundle(w1184) -> ("X"=w1182:u32)  [unwired: 1 out]
            n478 = Path To String(path=w1224) -> (string=w1239:string)
            n479 = Index Array(array=w1234, index=w1179) -> (element=w1235:string)
            n480 = Bundle("X"=w1182, 0) -> (w1183:cluster{"X":u32, i32})  [unwired: 1 in]
            n481 = local write "Data Name:"(w1235) -> ()
            n482 = property on="Image Out" class="ImageControl"(error in=w1180, "Image Center Position"=w1183) -> ()  [unwired: 1 in, 2 out]
            n483 = Concatenate Strings(w1239, "\\", w1235) -> (w1237:string)
            n484 = String To Path(string=w1237) -> (path=w1130:path)
            n485 = call "Recorded Values.vi"("Path"=w1130) -> ("Recorded Char"=w1177:T5, "Recorded Prop"=w1176:T6, "Fabrication Prop"=w1178:T7)  [unwired: 8 in]
            n486 = Unbundle By Name(w1177) -> ("Mobility-Sat"=w1164:dbl, "Moblitity-Lin"=w1163:dbl, "On/Off"=w1162:dbl, "Off Current"=w1161:dbl, "Vt-Sat"=w1126:dbl, "STS"=w1160:dbl, "Trap Density-VT"=w1159:dbl, "Trap Density-STS"=w1158:dbl)
            n487 = Unbundle By Name(w1178) -> ("Date Created"=w1157:string, "Material"=w1175:string, "Solvent"=w1174:string, "Concentration"=w1173:dbl, "Method"=w1172:string, "Dielectric (nm)"=w1171:dbl, "Treatment"=w1170:string, "Comments"=w1169:string)
            n488 = Unbundle By Name(w1176) -> ("Date Recorded"=w1168:string, "Index"=w1167:string, "Length"=w1166:dbl, "Width"=w1165:dbl, "Sample Temp"=w1128:dbl)
            n489 = local write "Date Created"(w1157) -> ()
            n490 = local write "Rec: Material"(w1175) -> ()
            n491 = local write "Rec: Off I-Sat"(w1161) -> ()
            n492 = local write "Rec: VT-Sat"(w1126) -> ()
            n493 = local write "Rec: Concentration"(w1173) -> ()
            n494 = local write "Rec: Method"(w1172) -> ()
            n495 = local write "Rec: Dielectric (d)"(w1171) -> ()
            n496 = local write "Surface Treatment:"(w1170) -> ()
            n497 = local write "Comments"(w1169) -> ()
            n498 = local write "Index"(w1167) -> ()
            n499 = local write "Rec: Mobility-Sat"(w1164) -> ()
            n500 = local write "Rec: Mobility-Lin"(w1163) -> ()
            n501 = local write "Rec: On/Off"(w1162) -> ()
            n502 = local write "Rec: STS"(w1160) -> ()
            n503 = local write "Rec: Trap Density-VT"(w1159) -> ()
            n504 = local write "Rec: Trap Density-STS"(w1158) -> ()
            n505 = local write "Rec: Solvent"(w1174) -> ()
            n506 = local write "Date Recorded"(w1168) -> ()
            n507 = local write "Rec: Length"(w1166) -> ()
            n508 = local write "Rec: Width"(w1165) -> ()
            n509 = local write "Rec: Temp"(w1128) -> ()
            n510 = Equal To 0?(x=w1128) -> (x = 0?=w1129:bool)
            n511 = case shown="False" w1129 {
              tunnel: [w1240 w1241] -> w1127
              tunnel: w1128 -> [w1240 _]
              frame False {
              }
              frame True {
                n512 = local read "Room Temp"() -> (w1241:dbl)
              }
            }
            n513 = local write "Transfer File"(w1130) -> ()
            n514 = local read "NumPts 2"() -> (w1152:dbl)
            n515 = local read "NumPts"() -> (w1153:dbl)
            n516 = call-poly <vilib>:"Read From Spreadsheet File.vi"("file path (dialog if empty)"=w1130) -> ("all rows"=w1231:string[][])  [unwired: 6 in, 4 out]
            n517 = local read "New: Dielectric"() -> (w1136:dbl)
            n518 = call "STS Calculator-File.vi"("NumPts"=w1152, "Path"=w1130) -> ("STS Index-Sat"=w1150:dbl, "XY Graph-Sat"=w1151:cluster{dbl[], dbl[]}[], "Ouput"=w1149:cluster{"STS-Sat":dbl, "STS-Lin":dbl})  [unwired: 5 in, 2 out]
            n519 = call "Mobility-Vt Calculator-File.vi"("NumPts"=w1153, "Path"=w1130) -> ("XY Graph-Sat"=w1156:cluster{dbl[], dbl[]}[], "XY Graph-Lin"=w1125:cluster{dbl[], dbl[]}[], "Output"=w1154:T8, "Index-Sat"=w1155:dbl, "Index-Lin"=w1142:dbl)  [unwired: 4 in, 1 out]
            n520 = Unbundle By Name(w1154) -> ("Mobility-Sat"=w1138:dbl, "Vt-Sat"=w1132:dbl, "Mobility-Lin"=w1137:dbl, "Vt-Lin"=w1123:dbl, "Off I-Sat"=w1131:dbl, "On/Off I-Sat"=w1124:dbl)
            n521 = local write "Index 2"(w1150) -> ()
            n522 = local write "XY Graph 2"(w1151) -> ()
            n523 = Unbundle By Name(w1149) -> ("STS-Sat"=w1133:dbl)  [unwired: 1 out]
            n524 = local write "MobVi Index"(w1155) -> ()
            n525 = Array Size(array=w1231) -> (size(s)=w1230:i32[])
            n526 = call "Trap Density_VT.vi"("VT"=w1132, "Dielectric"=w1136) -> ("Trap Density-VT"=w1135:dbl)
            n527 = call "Trap Density_STS.vi"("Temp (T) [K]"=w1127, "S.T.S. (S)"=w1133, "Dielectric"=w1136) -> ("Trap Density (N)"=w1134:dbl)  [unwired: 8 in]
            n528 = local write "Slide"(w1155) -> ()
            n529 = local write "Calc: Mobility-Lin"(w1137) -> ()
            n530 = local write "Calc: Mobility-Sat"(w1138) -> ()
            n531 = local write "Calc: VT-Sat"(w1132) -> ()
            n532 = local write "Calc: Off I-Sat"(w1131) -> ()
            n533 = local write "Calc: VT-Lin"(w1123) -> ()
            n534 = local write "Calc: On/Off"(w1124) -> ()
            n535 = local write "Calc: STS"(w1133) -> ()
            n536 = Decimate 1D Array(w1125) -> (w1148:cluster{dbl[], dbl[]}[])  [unwired: 1 out]
            n537 = local write "Calc: Trap Density-VT"(w1135) -> ()
            n538 = local write "Calc: Trap Density-STS"(w1134) -> ()
            n539 = local write "New: Trap Density-STS"(w1134) -> ()
            n540 = local write "New: Trap Density-VT"(w1135) -> ()
            n541 = local write "XY Graph-Lin"(w1125) -> ()
            n542 = local write "New: VT-Sat"(w1132) -> ()
            n543 = Decimate 1D Array(w1151) -> (w1205:cluster{dbl[], dbl[]}[])  [unwired: 1 out]
            n544 = Index Array(array=w1230, index=w1229) -> (element=w1211:i32)
            n545 = Decimate 1D Array(w1156) -> (w1214:cluster{dbl[], dbl[]}[])  [unwired: 1 out]
            n546 = local write "XY Graph"(w1156) -> ()
            n547 = local write "New: Mobility-Lin"(w1137) -> ()
            n548 = Array Subset(array=w1231, index (row)=w1229, index (col)=w1229, length (col)=3) -> (w1232:string[][])  [unwired: 1 in]
            n549 = local write "New: VT-Lin"(w1123) -> ()
            n550 = Array To Cluster(array=w1148) -> (cluster=w1147:T9)
            n551 = local write "New: STS"(w1133) -> ()
            n552 = local write "New: Mobility-Sat"(w1138) -> ()
            n553 = Array To Cluster(array=w1205) -> (cluster=w1203:T9)
            n554 = Array To Cluster(array=w1214) -> (cluster=w1216:T9)
            n555 = Reshape Array(w1232, w1211) -> (w1217:string[])
            n556 = Subtract(x=w1211, y=20) -> (x-y=w1209:i32)
            n557 = Unbundle(w1147) -> ("[0]"=w1146:cluster{dbl[], dbl[]})  [unwired: 8 out]
            n558 = property on="Slide" class="Slide (strict)"("Scale.Maximum"=w1209) -> ()  [unwired: 2 in, 2 out]
            n559 = local read "NumPts"() -> (w1143:dbl)
            n560 = Unbundle(w1146) -> (w1145:dbl[], w1144:dbl[])
            n561 = Unbundle(w1203) -> ("[0]"=w1204:cluster{dbl[], dbl[]})  [unwired: 8 out]
            n562 = Unbundle(w1216) -> ("[0]"=w1215:cluster{dbl[], dbl[]})  [unwired: 8 out]
            n563 = Search 1D Array(1D array=w1217, element="Index:") -> (index of element=w1226:i32)  [unwired: 1 in]
            n564 = local read "NumPts"() -> (w1139:dbl)
            n565 = Array Subset(array=w1145, index=w1142, length=w1143) -> (w1141:dbl[])
            n566 = Array Subset(array=w1144, index=w1142, length=w1143) -> (w1140:dbl[])
            n567 = Increment(x=w1226) -> (x+1=w1227:i32)
            n568 = Unbundle(w1204) -> (w1201:dbl[], w1200:dbl[])
            n569 = Unbundle(w1215) -> (w1202:dbl[], w1206:dbl[])
            n570 = local read "Image Folder"() -> (w1186:path)
            n571 = local write "Lin-Vg Array-Used"(w1141) -> ()
            n572 = Array Subset(array=w1201, index=w1150, length=w1152) -> (w1208:dbl[])
            n573 = Array Subset(array=w1200, index=w1150, length=w1152) -> (w1207:dbl[])
            n574 = Array Subset(array=w1202, index=w1155, length=w1139) -> (w1213:dbl[])
            n575 = Array Subset(array=w1206, index=w1155, length=w1139) -> (w1212:dbl[])
            n576 = Index Array(array=w1217, index=w1227) -> (element=w1188:string)
            n577 = local write "Lin Id-Used"(w1140) -> ()
            n578 = local write "Sat Vg Array-Used"(w1213) -> ()
            n579 = local write "Vg Array-Log-Used"(w1207) -> ()
            n580 = local write "Sat Id-Log-Used"(w1208) -> ()
            n581 = local write "Sat Id-Used"(w1212) -> ()
            n582 = local write "Index"(w1188) -> ()
            n583 = List Folder(path=w1186, error in=w1190) -> (filenames=w1222:string[], error out=w1189:errorcluster)  [unwired: 2 in, 2 out]
            n584 = Build Path(base path=w1186, name or relative path="ROI") -> (appended path=w1185:path)
            n585 = invoke on="Image Out" class="ImageControl" method="Clear ROI"(error in=w1189) -> (error out=w1193:errorcluster)  [unwired: 2 in, 2 out]
            n586 = Build Path(base path=w1185, name or relative path=w1188) -> (appended path=w1194:path)
            n587 = while {
              tunnel: w1222 -> [w1254]
              tunnel: w1188 -> [w1252]
              tunnel: [w1251] -> _
              tunnel: [w1251] -> w1221
              tunnel: w1211 -> [w1250]
              i -> [w1251]
              stop <- w1247 stop-if-true
              n588 = Index Array(array=w1254, index=w1251) -> (element=w1255:string)
              n589 = xnode "Match Regular Expression"("input string"=w1255, "regular expression"=w1252) -> ("whole match"=w1253:string)  [unwired: 4 in, 4 out]
              n590 = Equal?(x=w1253, y=w1252) -> (x = y?=w1249:bool)
              n591 = Equal?(x=w1250, y=w1251) -> (x = y?=w1248:bool)
              n592 = Or(x=w1249, y=w1248) -> (x .or. y?=w1247:bool)
            }
            n593 = call <vilib>:"Check if File or Folder Exists.vi"("error in (no error)"=w1193, "path"=w1194) -> ("file or folder exists?"=w1191:bool, "dup path"=w1192:path)  [unwired: 7 in, 1 out]
            n594 = case shown="True" w1191 {
              tunnel: w1192 -> [_ w1242]
              frame False {
              }
              frame True {
                n595 = Read from Text File(file (use dialog)=w1242) -> (text=w1246:string)  [unwired: 3 in, 3 out]
                n596 = property on="Image Out" class="ImageControl"() -> ("ROI"=w1243:T10)  [unwired: 2 in, 2 out]
                n597 = Unflatten From String(type=w1243, binary string=w1246) -> (value=w1244:T10, error out=w1245:errorcluster)  [unwired: 3 in, 1 out]
                n598 = property on="Image Out" class="ImageControl"(error in=w1245, "ROI"=w1244) -> ()  [unwired: 1 in, 2 out]
              }
            }
            n599 = invoke on="Image Out" class="ImageControl" method="Clear ROI"() -> ()  [unwired: 3 in, 3 out]
            n600 = Path To String(path=w1186) -> (string=w1220:string)
            n601 = Index Array(array=w1222, index=w1221) -> (element=w1198:string)
            n602 = Concatenate Strings(w1220, "\\", w1198) -> (w1219:string)
            n603 = local write "Image Name"(w1198) -> ()
            n604 = String To Path(string=w1219) -> (path=w1197:path)
            n605 = Empty String/Path?(string/path=w1198) -> (empty?=w1199:bool)
            n606 = local read "No Image File"() -> (w1195:path)
            n607 = Select(t=w1195, s=w1199, f=w1197) -> (s? t:f=w1196:path)
            n608 = local write "Image File"(w1196) -> ()
            n609 = call "Vision Acquisition3"("Image Path"=w1196) -> ("Image Out"=w1223:T2)  [unwired: 25 in, 1 out]
            n610 = local write "Image Out"(w1223) -> ()
            n611 = local write "Image Out 2"(w1223) -> ()
          }
          event "Up Button": Mouse Down {
            w1474 = 0
            n612 = event-data() -> ()  [unwired: 1 in, 5 out]
            n613 = local read "Transfer File"() -> (w1470:path)
            n614 = Strip Path(path=w1470) -> (stripped path=w1469:path, name=w1485:string)
            n615 = local write "Transfer Folder"(w1469) -> ()
            n616 = List Folder(path=w1469) -> (filenames=w1479:string[], error out=w1436:errorcluster)  [unwired: 3 in, 2 out]
            n617 = Array Size(array=w1479) -> (size(s)=w1424:i32)
            n618 = Search 1D Array(1D array=w1479, element=w1485) -> (index of element=w1480:i32)  [unwired: 1 in]
            n619 = Equal To 0?(x=w1480) -> (x = 0?=w1481:bool)
            n620 = local read "Folder Index"() -> (w1423:dbl)
            n621 = property on="Image Out" class="ImageControl"() -> (error out=w1426:errorcluster, "Image Center Position"=w1430:cluster{"X":u32, "Y":u32})  [unwired: 2 in, 1 out]
            n622 = case shown="True" w1481 {
              tunnel: w1423 -> [w1615 _]
              tunnel: [w1614 w1616] -> w1422
              tunnel: w1424 -> [_ w1617]
              frame False {
                n623 = Decrement(x=w1615) -> (x-1=w1614:dbl)
              }
              frame True {
                n624 = Decrement(x=w1617) -> (x-1=w1616:i32)
              }
            }
            n625 = Unbundle(w1430) -> ("X"=w1428:u32)  [unwired: 1 out]
            n626 = local write "Folder Index"(w1422) -> ()
            n627 = Bundle("X"=w1428, 0) -> (w1429:cluster{"X":u32, i32})  [unwired: 1 in]
            n628 = Path To String(path=w1469) -> (string=w1486:string)
            n629 = Index Array(array=w1479, index=w1422) -> (element=w1482:string)
            n630 = local write "Data Name:"(w1482) -> ()
            n631 = property on="Image Out" class="ImageControl"(error in=w1426, "Image Center Position"=w1429) -> ()  [unwired: 1 in, 2 out]
            n632 = Concatenate Strings(w1486, "\\", w1482) -> (w1484:string)
            n633 = String To Path(string=w1484) -> (path=w1373:path)
            n634 = call "Recorded Values.vi"("Path"=w1373) -> ("Recorded Char"=w1420:T5, "Recorded Prop"=w1419:T6, "Fabrication Prop"=w1421:T7)  [unwired: 8 in]
            n635 = Unbundle By Name(w1420) -> ("Mobility-Sat"=w1407:dbl, "Moblitity-Lin"=w1406:dbl, "On/Off"=w1405:dbl, "Off Current"=w1404:dbl, "Vt-Sat"=w1369:dbl, "STS"=w1403:dbl, "Trap Density-VT"=w1402:dbl, "Trap Density-STS"=w1401:dbl)
            n636 = Unbundle By Name(w1421) -> ("Date Created"=w1400:string, "Material"=w1418:string, "Solvent"=w1417:string, "Concentration"=w1416:dbl, "Method"=w1415:string, "Dielectric (nm)"=w1414:dbl, "Treatment"=w1413:string, "Comments"=w1412:string)
            n637 = Unbundle By Name(w1419) -> ("Date Recorded"=w1411:string, "Index"=w1410:string, "Length"=w1409:dbl, "Width"=w1408:dbl, "Sample Temp"=w1370:dbl)
            n638 = local write "Date Created"(w1400) -> ()
            n639 = local write "Rec: Material"(w1418) -> ()
            n640 = local write "Rec: Off I-Sat"(w1404) -> ()
            n641 = local write "Rec: VT-Sat"(w1369) -> ()
            n642 = local write "Rec: Solvent"(w1417) -> ()
            n643 = local write "Rec: Concentration"(w1416) -> ()
            n644 = local write "Rec: Method"(w1415) -> ()
            n645 = local write "Rec: Dielectric (d)"(w1414) -> ()
            n646 = local write "Surface Treatment:"(w1413) -> ()
            n647 = local write "Comments"(w1412) -> ()
            n648 = local write "Index"(w1410) -> ()
            n649 = local write "Rec: Mobility-Sat"(w1407) -> ()
            n650 = local write "Rec: Mobility-Lin"(w1406) -> ()
            n651 = local write "Rec: On/Off"(w1405) -> ()
            n652 = local write "Rec: STS"(w1403) -> ()
            n653 = local write "Rec: Trap Density-VT"(w1402) -> ()
            n654 = local write "Rec: Trap Density-STS"(w1401) -> ()
            n655 = local write "Date Recorded"(w1411) -> ()
            n656 = local write "Rec: Length"(w1409) -> ()
            n657 = local write "Rec: Width"(w1408) -> ()
            n658 = local write "Rec: Temp"(w1370) -> ()
            n659 = Equal To 0?(x=w1370) -> (x = 0?=w1372:bool)
            n660 = case shown="False" w1372 {
              tunnel: [w1487 w1488] -> w1371
              tunnel: w1370 -> [w1487 _]
              frame False {
              }
              frame True {
                n661 = local read "Room Temp"() -> (w1488:dbl)
              }
            }
            n662 = local write "Transfer File"(w1373) -> ()
            n663 = local read "NumPts 2"() -> (w1395:dbl)
            n664 = local read "NumPts"() -> (w1399:dbl)
            n665 = local read "New: Dielectric"() -> (w1379:dbl)
            n666 = call "Mobility-Vt Calculator-File.vi"("NumPts"=w1399, "Path"=w1373) -> ("XY Graph-Sat"=w1397:cluster{dbl[], dbl[]}[], "XY Graph-Lin"=w1368:cluster{dbl[], dbl[]}[], "Output"=w1398:T8, "Index-Sat"=w1396:dbl, "Index-Lin"=w1383:dbl)  [unwired: 4 in, 1 out]
            n667 = call "STS Calculator-File.vi"("NumPts"=w1395, "Path"=w1373) -> ("STS Index-Sat"=w1394:dbl, "XY Graph-Sat"=w1393:cluster{dbl[], dbl[]}[], "Ouput"=w1392:cluster{"STS-Sat":dbl, "STS-Lin":dbl})  [unwired: 5 in, 2 out]
            n668 = call-poly <vilib>:"Read From Spreadsheet File.vi"("file path (dialog if empty)"=w1373) -> ("all rows"=w1476:string[][])  [unwired: 6 in, 4 out]
            n669 = Unbundle By Name(w1398) -> ("Mobility-Sat"=w1382:dbl, "Vt-Sat"=w1375:dbl, "Mobility-Lin"=w1381:dbl, "Vt-Lin"=w1380:dbl, "Off I-Sat"=w1374:dbl, "On/Off I-Sat"=w1367:dbl)
            n670 = Unbundle By Name(w1392) -> ("STS-Sat"=w1376:dbl)  [unwired: 1 out]
            n671 = local write "Index 2"(w1394) -> ()
            n672 = local write "XY Graph 2"(w1393) -> ()
            n673 = local write "MobVi Index"(w1396) -> ()
            n674 = local write "Slide"(w1396) -> ()
            n675 = local write "XY Graph"(w1397) -> ()
            n676 = local write "Calc: Mobility-Sat"(w1382) -> ()
            n677 = local write "Calc: VT-Sat"(w1375) -> ()
            n678 = local write "Calc: Mobility-Lin"(w1381) -> ()
            n679 = local write "Calc: Off I-Sat"(w1374) -> ()
            n680 = local write "Calc: On/Off"(w1367) -> ()
            n681 = Array Size(array=w1476) -> (size(s)=w1475:i32[])
            n682 = local write "Calc: VT-Lin"(w1380) -> ()
            n683 = call "Trap Density_VT.vi"("VT"=w1375, "Dielectric"=w1379) -> ("Trap Density-VT"=w1378:dbl)
            n684 = call "Trap Density_STS.vi"("Temp (T) [K]"=w1371, "S.T.S. (S)"=w1376, "Dielectric"=w1379) -> ("Trap Density (N)"=w1377:dbl)  [unwired: 8 in]
            n685 = local write "Calc: STS"(w1376) -> ()
            n686 = local write "New: STS"(w1376) -> ()
            n687 = Decimate 1D Array(w1368) -> (w1391:cluster{dbl[], dbl[]}[])  [unwired: 1 out]
            n688 = local write "Calc: Trap Density-VT"(w1378) -> ()
            n689 = local write "New: VT-Sat"(w1375) -> ()
            n690 = local write "Calc: Trap Density-STS"(w1377) -> ()
            n691 = local write "New: Trap Density-STS"(w1377) -> ()
            n692 = local write "New: Trap Density-VT"(w1378) -> ()
            n693 = local write "XY Graph-Lin"(w1368) -> ()
            n694 = local write "New: VT-Lin"(w1380) -> ()
            n695 = local write "New: Mobility-Sat"(w1382) -> ()
            n696 = local write "New: Mobility-Lin"(w1381) -> ()
            n697 = Decimate 1D Array(w1393) -> (w1453:cluster{dbl[], dbl[]}[])  [unwired: 1 out]
            n698 = Index Array(array=w1475, index=w1474) -> (element=w1459:i32)
            n699 = Decimate 1D Array(w1397) -> (w1463:cluster{dbl[], dbl[]}[])  [unwired: 1 out]
            n700 = Array To Cluster(array=w1391) -> (cluster=w1390:T9)
            n701 = Array Subset(array=w1476, index (row)=w1474, index (col)=w1474, length (col)=3) -> (w1477:string[][])  [unwired: 1 in]
            n702 = Array To Cluster(array=w1453) -> (cluster=w1451:T9)
            n703 = Array To Cluster(array=w1463) -> (cluster=w1465:T9)
            n704 = Reshape Array(w1477, w1459) -> (w1466:string[])
            n705 = Subtract(x=w1459, y=20) -> (x-y=w1458:i32)
            n706 = Unbundle(w1390) -> ("[0]"=w1387:cluster{dbl[], dbl[]})  [unwired: 8 out]
            n707 = property on="Slide" class="Slide (strict)"("Scale.Maximum"=w1458) -> ()  [unwired: 2 in, 2 out]
            n708 = Unbundle(w1451) -> ("[0]"=w1452:cluster{dbl[], dbl[]})  [unwired: 8 out]
            n709 = Unbundle(w1465) -> ("[0]"=w1464:cluster{dbl[], dbl[]})  [unwired: 8 out]
            n710 = local read "NumPts"() -> (w1384:dbl)
            n711 = Unbundle(w1387) -> (w1386:dbl[], w1385:dbl[])
            n712 = Search 1D Array(1D array=w1466, element="Index:") -> (index of element=w1471:i32)  [unwired: 1 in]
            n713 = Increment(x=w1471) -> (x+1=w1472:i32)
            n714 = Unbundle(w1452) -> (w1450:dbl[], w1449:dbl[])
            n715 = Unbundle(w1464) -> (w1457:dbl[], w1456:dbl[])
            n716 = Array Subset(array=w1386, index=w1383, length=w1384) -> (w1388:dbl[])
            n717 = Array Subset(array=w1385, index=w1383, length=w1384) -> (w1389:dbl[])
            n718 = local read "Image Folder"() -> (w1425:path)
            n719 = local write "Lin-Vg Array-Used"(w1388) -> ()
            n720 = Array Subset(array=w1450, index=w1394, length=w1395) -> (w1455:dbl[])
            n721 = Array Subset(array=w1449, index=w1394, length=w1395) -> (w1454:dbl[])
            n722 = Array Subset(array=w1457, index=w1396, length=w1399) -> (w1462:dbl[])
            n723 = Array Subset(array=w1456, index=w1396, length=w1399) -> (w1461:dbl[])
            n724 = local write "Lin Id-Used"(w1389) -> ()
            n725 = Index Array(array=w1466, index=w1472) -> (element=w1432:string)
            n726 = local write "Sat Vg Array-Used"(w1462) -> ()
            n727 = local write "Vg Array-Log-Used"(w1454) -> ()
            n728 = local write "Sat Id-Log-Used"(w1455) -> ()
            n729 = local write "Sat Id-Used"(w1461) -> ()
            n730 = local write "Index"(w1432) -> ()
            n731 = List Folder(path=w1425, error in=w1436) -> (filenames=w1468:string[], error out=w1435:errorcluster)  [unwired: 2 in, 2 out]
            n732 = Build Path(base path=w1425, name or relative path="ROI") -> (appended path=w1433:path)
            n733 = while {
              tunnel: w1468 -> [w1501]
              tunnel: w1432 -> [w1499]
              tunnel: [w1498] -> w1467
              tunnel: w1459 -> [w1497]
              i -> [w1498]
              stop <- w1494 stop-if-true
              n734 = Index Array(array=w1501, index=w1498) -> (element=w1502:string)
              n735 = xnode "Match Regular Expression"("input string"=w1502, "regular expression"=w1499) -> ("whole match"=w1500:string)  [unwired: 4 in, 4 out]
              n736 = Equal?(x=w1500, y=w1499) -> (x = y?=w1496:bool)
              n737 = Equal?(x=w1497, y=w1498) -> (x = y?=w1495:bool)
              n738 = Or(x=w1496, y=w1495) -> (x .or. y?=w1494:bool)
            }
            n739 = invoke on="Image Out" class="ImageControl" method="Clear ROI"(error in=w1435) -> (error out=w1439:errorcluster)  [unwired: 2 in, 2 out]
            n740 = Build Path(base path=w1433, name or relative path=w1432) -> (appended path=w1431:path)
            n741 = call <vilib>:"Check if File or Folder Exists.vi"("error in (no error)"=w1439, "path"=w1431) -> ("file or folder exists?"=w1437:bool, "dup path"=w1438:path)  [unwired: 7 in, 1 out]
            n742 = case shown="True" w1437 {
              tunnel: w1438 -> [_ w1489]
              frame False {
              }
              frame True {
                n743 = Read from Text File(file (use dialog)=w1489) -> (text=w1493:string)  [unwired: 3 in, 3 out]
                n744 = property on="Image Out" class="ImageControl"() -> ("ROI"=w1490:T10)  [unwired: 2 in, 2 out]
                n745 = Unflatten From String(type=w1490, binary string=w1493) -> (value=w1491:T10, error out=w1492:errorcluster)  [unwired: 3 in, 1 out]
                n746 = property on="Image Out" class="ImageControl"(error in=w1492, "ROI"=w1491) -> ()  [unwired: 1 in, 2 out]
              }
            }
            n747 = Index Array(array=w1468, index=w1467) -> (element=w1441:string)
            n748 = local write "Image Name"(w1441) -> ()
            n749 = Empty String/Path?(string/path=w1441) -> (empty?=w1448:bool)
            n750 = Build Path(base path=w1425, name or relative path=w1441) -> (appended path=w1440:path)
            n751 = local read "No Image File"() -> (w1447:path)
            n752 = Select(t=w1447, s=w1448, f=w1440) -> (s? t:f=w1442:path)
            n753 = call <vilib>:"Get File Extension.vi"("file"=w1442) -> ("lowercase file extension"=w1444:string)  [unwired: 7 in, 3 out]
            n754 = local write "Image File"(w1442) -> ()
            n755 = local write "String"(w1444) -> ()
            n756 = Search 1D Array(1D array=string[] ["bmp", "jpeg", "png", "jpg", "gif"], element=w1444) -> (index of element=w1443:i32)  [unwired: 1 in]
            n757 = call "Vision Acquisition5"("Image Path"=w1442) -> ("Image Out"=w1446:T2)  [unwired: 25 in, 1 out]
            n758 = Less Than 0?(x=w1443) -> ()  [unwired: 1 out]
            n759 = local write "Image Out"(w1446) -> ()
            n760 = local write "Image Out 2"(w1446) -> ()
          }
          event "Save Changes? 3": Mouse Down {
            n761 = event-data() -> ()  [unwired: 1 in, 7 out]
            n762 = local read "Image Folder"() -> (w1618:path)
            n763 = Build Path(base path=w1618, name or relative path="ROI") -> (appended path=w1625:path)
            n764 = call <vilib>:"Check if File or Folder Exists.vi"("path"=w1625) -> ("file or folder exists?"=w1627:bool, "dup path"=w1624:path)  [unwired: 8 in, 1 out]
            n765 = case shown="False" w1627 {
              tunnel: w1624 -> [w1629 w1630]
              tunnel: [w1628 w1630] -> w1619
              frame False {
                n766 = Create Folder(path (use dialog)=w1629) -> (created path=w1628:path)  [unwired: 2 in, 2 out]
              }
              frame True {
              }
            }
            n767 = local read "Index"() -> (w1621:string)
            n768 = property on="Image Out" class="ImageControl"() -> ("ROI"=w1623:T10)  [unwired: 2 in, 2 out]
            n769 = Build Path(base path=w1619, name or relative path=w1621) -> (appended path=w1620:path)
            n770 = Flatten To String(anything=w1623) -> (data string=w1622:string)  [unwired: 3 in, 2 out]
            n771 = Write to Text File(file (use dialog)=w1620, text=w1622) -> ()  [unwired: 2 in, 3 out]
          }
          event "Next Button": Mouse Down {
            n772 = event-data() -> ()  [unwired: 1 in, 5 out]
            n773 = local read "XY Graph"() -> (w1643:cluster{dbl[], dbl[]}[])
            n774 = Decimate 1D Array(w1643) -> (w1639:cluster{dbl[], dbl[]}[], w1638:cluster{dbl[], dbl[]}[])
            n775 = Array To Cluster(array=w1639) -> (cluster=w1649:T9)
            n776 = local read "MobVi Index"() -> (w1645:dbl)
            n777 = Unbundle(w1649) -> ("[0]"=w1648:cluster{dbl[], dbl[]})  [unwired: 8 out]
            n778 = local read "NumPts"() -> (w1644:dbl)
            n779 = Unbundle(w1648) -> (w1647:dbl[], w1646:dbl[])
            n780 = Increment(x=w1645) -> (x+1=w1640:dbl)
            n781 = local read "New: Dielectric"() -> (w1634:dbl)
            n782 = local read "New: Length"() -> (w1633:dbl)
            n783 = local read "New: Width"() -> (w1632:dbl)
            n784 = local write "MobVi Index"(w1640) -> ()
            n785 = Array Subset(array=w1647, index=w1640, length=w1644) -> (w1636:dbl[])
            n786 = Array Subset(array=w1646, index=w1640, length=w1644) -> (w1635:dbl[])
            n787 = local write "Sat Vg Array-Used"(w1636) -> ()
            n788 = local write "Sat Id-Used"(w1635) -> ()
            n789 = call "Mobility-Vt-Used Pts_Saturation.vi"("Width"=w1632, "Length"=w1633, "Dielectric (d)"=w1634, "Sat Id Used"=w1635, "Vg Used"=w1636) -> ("Vt"=w1631:dbl, "Mobility"=w1637:dbl)  [unwired: 4 in, 1 out]
            n790 = Bundle(w1636, w1635) -> (w1642:cluster{dbl[], dbl[]})  [unwired: 1 in]
            n791 = Build Array (concatenate)(w1639, w1638, w1642) -> (w1641:cluster{dbl[], dbl[]}[])
            n792 = local write "New: Mobility-Sat"(w1637) -> ()
            n793 = local write "New: VT-Sat"(w1631) -> ()
            n794 = local write "XY Graph"(w1641) -> ()
          }
          event "Next Button 2": Mouse Down {
            n795 = event-data() -> ()  [unwired: 1 in, 7 out]
            n796 = local read "XY Graph 2"() -> (w1658:cluster{dbl[], dbl[]}[])
            n797 = Decimate 1D Array(w1658) -> (w1654:cluster{dbl[], dbl[]}[], w1653:cluster{dbl[], dbl[]}[])
            n798 = Array To Cluster(array=w1654) -> (cluster=w1664:T9)
            n799 = local read "Index 2"() -> (w1660:dbl)
            n800 = Unbundle(w1664) -> ("[0]"=w1663:cluster{dbl[], dbl[]})  [unwired: 8 out]
            n801 = local read "NumPts 2"() -> (w1659:dbl)
            n802 = Unbundle(w1663) -> (w1662:dbl[], w1661:dbl[])
            n803 = Increment(x=w1660) -> (x+1=w1655:dbl)
            n804 = local write "Index 2"(w1655) -> ()
            n805 = Array Subset(array=w1661, index=w1655, length=w1659) -> (w1650:dbl[])
            n806 = Array Subset(array=w1662, index=w1655, length=w1659) -> (w1651:dbl[])
            n807 = call "STS-Used.vi"("Id Used"=w1651, "Vg-Used"=w1650) -> ("STS"=w1652:dbl)  [unwired: 9 in]
            n808 = Bundle(w1651, w1650) -> (w1657:cluster{dbl[], dbl[]})  [unwired: 1 in]
            n809 = local write "Vg Array-Log-Used"(w1650) -> ()
            n810 = local write "Sat Id-Log-Used"(w1651) -> ()
            n811 = local write "New: STS"(w1652) -> ()
            n812 = Build Array (concatenate)(w1654, w1653, w1657) -> (w1656:cluster{dbl[], dbl[]}[])
            n813 = local write "XY Graph 2"(w1656) -> ()
          }
          event "Previous Button 2": Mouse Down {
            n814 = event-data() -> ()  [unwired: 1 in, 7 out]
            n815 = local read "XY Graph 2"() -> (w1674:cluster{dbl[], dbl[]}[])
            n816 = Decimate 1D Array(w1674) -> (w1671:cluster{dbl[], dbl[]}[], w1670:cluster{dbl[], dbl[]}[])
            n817 = Array To Cluster(array=w1671) -> (cluster=w1679:T9)
            n818 = local read "Index 2"() -> (w1667:dbl)
            n819 = Unbundle(w1679) -> ("[0]"=w1678:cluster{dbl[], dbl[]})  [unwired: 8 out]
            n820 = local read "NumPts 2"() -> (w1675:dbl)
            n821 = Unbundle(w1678) -> (w1677:dbl[], w1676:dbl[])
            n822 = Decrement(x=w1667) -> (x-1=w1668:dbl)
            n823 = local write "Index 2"(w1668) -> ()
            n824 = Array Subset(array=w1677, index=w1668, length=w1675) -> (w1665:dbl[])
            n825 = Array Subset(array=w1676, index=w1668, length=w1675) -> (w1666:dbl[])
            n826 = local write "Vg Array-Log-Used"(w1666) -> ()
            n827 = local write "Sat Id-Log-Used"(w1665) -> ()
            n828 = Bundle(w1665, w1666) -> (w1673:cluster{dbl[], dbl[]})  [unwired: 1 in]
            n829 = call "STS-Used.vi"("Id Used"=w1665, "Vg-Used"=w1666) -> ("STS"=w1669:dbl)  [unwired: 9 in]
            n830 = Build Array (concatenate)(w1671, w1670, w1673) -> (w1672:cluster{dbl[], dbl[]}[])
            n831 = local write "New: STS"(w1669) -> ()
            n832 = local write "XY Graph 2"(w1672) -> ()
          }
          event "Previous Button": Mouse Down {
            n833 = event-data() -> ()  [unwired: 1 in, 5 out]
            n834 = local read "XY Graph"() -> (w1693:cluster{dbl[], dbl[]}[])
            n835 = Decimate 1D Array(w1693) -> (w1690:cluster{dbl[], dbl[]}[], w1689:cluster{dbl[], dbl[]}[])
            n836 = Array To Cluster(array=w1690) -> (cluster=w1698:T9)
            n837 = local read "MobVi Index"() -> (w1688:dbl)
            n838 = Unbundle(w1698) -> ("[0]"=w1697:cluster{dbl[], dbl[]})  [unwired: 8 out]
            n839 = local read "NumPts"() -> (w1694:dbl)
            n840 = Unbundle(w1697) -> (w1696:dbl[], w1695:dbl[])
            n841 = Decrement(x=w1688) -> (x-1=w1687:dbl)
            n842 = local read "New: Dielectric"() -> (w1681:dbl)
            n843 = local read "New: Length"() -> (w1682:dbl)
            n844 = local read "New: Width"() -> (w1683:dbl)
            n845 = local write "MobVi Index"(w1687) -> ()
            n846 = Array Subset(array=w1696, index=w1687, length=w1694) -> (w1686:dbl[])
            n847 = Array Subset(array=w1695, index=w1687, length=w1694) -> (w1685:dbl[])
            n848 = local write "Sat Vg Array-Used"(w1686) -> ()
            n849 = local write "Sat Id-Used"(w1685) -> ()
            n850 = call "Mobility-Vt-Used Pts_Linear.vi"("Width"=w1683, "Length"=w1682, "Dielectric (d)"=w1681, "Sat Id Used"=w1685, "Vg Used"=w1686) -> ("Vt"=w1680:dbl, "Mobility"=w1684:dbl)  [unwired: 4 in, 1 out]
            n851 = Bundle(w1686, w1685) -> (w1692:cluster{dbl[], dbl[]})  [unwired: 1 in]
            n852 = local write "New: VT-Sat"(w1680) -> ()
            n853 = Build Array (concatenate)(w1690, w1689, w1692) -> (w1691:cluster{dbl[], dbl[]}[])
            n854 = local write "New: Mobility-Sat"(w1684) -> ()
            n855 = local write "XY Graph"(w1691) -> ()
          }
          event "Slide": Value Change {
            n856 = event-data() -> ()  [unwired: 1 in, 5 out]
            n857 = local read "XY Graph"() -> (w1711:cluster{dbl[], dbl[]}[])
            n858 = Decimate 1D Array(w1711) -> (w1708:cluster{dbl[], dbl[]}[], w1707:cluster{dbl[], dbl[]}[])
            n859 = Array To Cluster(array=w1708) -> (cluster=w1716:T9)
            n860 = Unbundle(w1716) -> ("[0]"=w1715:cluster{dbl[], dbl[]})  [unwired: 8 out]
            n861 = local read "NumPts"() -> (w1712:dbl)
            n862 = local read "Slide"() -> (w1700:dbl)
            n863 = Unbundle(w1715) -> (w1714:dbl[], w1713:dbl[])
            n864 = local read "New: Dielectric"() -> (w1701:dbl)
            n865 = local read "New: Length"() -> (w1702:dbl)
            n866 = local read "New: Width"() -> (w1703:dbl)
            n867 = local write "MobVi Index"(w1700) -> ()
            n868 = Array Subset(array=w1714, index=w1700, length=w1712) -> (w1706:dbl[])
            n869 = Array Subset(array=w1713, index=w1700, length=w1712) -> (w1705:dbl[])
            n870 = local write "Sat Vg Array-Used"(w1706) -> ()
            n871 = local write "Sat Id-Used"(w1705) -> ()
            n872 = call "Mobility-Vt-Used Pts_Linear.vi"("Width"=w1703, "Length"=w1702, "Dielectric (d)"=w1701, "Sat Id Used"=w1705, "Vg Used"=w1706) -> ("Vt"=w1699:dbl, "Mobility"=w1704:dbl)  [unwired: 4 in, 1 out]
            n873 = Bundle(w1706, w1705) -> (w1710:cluster{dbl[], dbl[]})  [unwired: 1 in]
            n874 = local write "New: VT-Sat"(w1699) -> ()
            n875 = Build Array (concatenate)(w1708, w1707, w1710) -> (w1709:cluster{dbl[], dbl[]}[])
            n876 = local write "New: Mobility-Sat"(w1704) -> ()
            n877 = local write "XY Graph"(w1709) -> ()
          }
          event "Slide 2": Value Change {
            n878 = event-data() -> ()  [unwired: 1 in, 5 out]
            n879 = local read "XY Graph 2"() -> (w1725:cluster{dbl[], dbl[]}[])
            n880 = Decimate 1D Array(w1725) -> (w1722:cluster{dbl[], dbl[]}[], w1721:cluster{dbl[], dbl[]}[])
            n881 = Array To Cluster(array=w1722) -> (cluster=w1730:T9)
            n882 = Unbundle(w1730) -> ("[0]"=w1729:cluster{dbl[], dbl[]})  [unwired: 8 out]
            n883 = local read "NumPts 2"() -> (w1726:dbl)
            n884 = local read "Slide 2"() -> (w1720:dbl)
            n885 = Unbundle(w1729) -> (w1728:dbl[], w1727:dbl[])
            n886 = local write "Index 2"(w1720) -> ()
            n887 = Array Subset(array=w1728, index=w1720, length=w1726) -> (w1718:dbl[])
            n888 = Array Subset(array=w1727, index=w1720, length=w1726) -> (w1717:dbl[])
            n889 = local write "Vg Array-Log-Used"(w1717) -> ()
            n890 = local write "Sat Id-Log-Used"(w1718) -> ()
            n891 = call "STS-Used.vi"("Id Used"=w1718, "Vg-Used"=w1717) -> ("STS"=w1719:dbl)  [unwired: 9 in]
            n892 = Bundle(w1718, w1717) -> (w1724:cluster{dbl[], dbl[]})  [unwired: 1 in]
            n893 = local write "New: STS"(w1719) -> ()
            n894 = Build Array (concatenate)(w1722, w1721, w1724) -> (w1723:cluster{dbl[], dbl[]}[])
            n895 = local write "XY Graph 2"(w1723) -> ()
          }
          event "Save Changes?": Mouse Down {
            n896 = event-data() -> ()  [unwired: 1 in, 5 out]
            n897 = flat-sequence {
              tunnel: [w1736] -> w1735
              tunnel: [w1744] -> w1734
              tunnel: [w1737] -> w1733
              tunnel: w1735 -> [w2253]
              tunnel: w1734 -> [w2250]
              tunnel: [w2251] -> w1732
              tunnel: w1733 -> [w2251]
              tunnel: [w2250] -> w1731
              tunnel: w1732 -> [w2258]
              tunnel: w1731 -> [w2257]
              frame #0 {
                n898 = local read "Transfer File"() -> (w1736:path)
                n899 = local read "New: Temp"() -> (w1738:dbl)
                n900 = local read "New: Length"() -> (w1742:dbl)
                n901 = local read "New: Width"() -> (w1740:dbl)
                n902 = To Single Precision Float(number=w1738) -> (single precision float=w1739:sgl)
                n903 = Number To Decimal String(number=w1739) -> (decimal integer string=w1747:string)  [unwired: 1 in]
                n904 = To Single Precision Float(number=w1740) -> (single precision float=w1741:sgl)
                n905 = To Single Precision Float(number=w1742) -> (single precision float=w1743:sgl)
                n906 = local read "Index"() -> (w1752:string)
                n907 = Strip Path(path=w1736) -> (stripped path=w1757:path)  [unwired: 1 out]
                n908 = Number To Decimal String(number=w1743) -> (decimal integer string=w1750:string)  [unwired: 1 in]
                n909 = Number To Decimal String(number=w1741) -> (decimal integer string=w1751:string)  [unwired: 1 in]
                n910 = Concatenate Strings("_", w1747, "K") -> (w1745:string)
                n911 = call "Build Text"("Temp"=w1745, "Index"=w1752, "Length"=w1750, "Width"=w1751) -> ("Result"=w1753:string)  [unwired: 10 in, 1 out]
                n912 = flat-sequence {
                  tunnel: [w2207] -> w1749
                  tunnel: w1749 -> [w2224]
                  frame #0 {
                    # "Makes Empty File for Transformer Data"
                    n913 = local read "Transfer Folder"() -> (w2196:path)
                    n914 = Build Path(base path=w2196, name or relative path="Stats") -> (appended path=w2198:path)
                    n915 = call <vilib>:"Check if File or Folder Exists.vi"("path"=w2198) -> ("file or folder exists?"=w2199:bool, "dup path"=w2200:path)  [unwired: 8 in, 1 out]
                    n916 = case shown="False" w2199 {
                      tunnel: [w2204 w2206] -> w2201
                      tunnel: w2200 -> [w2205 w2206]
                      frame False {
                        n917 = Create Folder(path (use dialog)=w2205) -> (created path=w2204:path)  [unwired: 2 in, 2 out]
                      }
                      frame True {
                      }
                    }
                    n918 = Build Path(base path=w2201, name or relative path="Tranformer Data.txt") -> (appended path=w2203:path)
                    n919 = call-poly <vilib>:"Write To Spreadsheet File.vi"("append to file? (new file:F)"=TRUE, "file path (dialog if empty)"=w2203) -> ()  [unwired: 6 in, 1 out]
                  }
                  frame #1 {
                    # "Adds Headers if they don't exist"
                    n920 = local read "Transfer Folder"() -> (w2213:path)
                    n921 = Concatenate Strings("Stats\\", "Tranformer Data.txt") -> (w2214:string)
                    n922 = Build Path(base path=w2213, name or relative path=w2214) -> (appended path=w2207:path)
                    n923 = call-poly <vilib>:"Read From Spreadsheet File.vi"("file path (dialog if empty)"=w2207) -> ("first row"=w2212:string[])  [unwired: 6 in, 4 out]
                    n924 = Search 1D Array(1D array=w2212, element="DeviceID") -> (index of element=w2210:i32)  [unwired: 1 in]
                    n925 = Equal?(x=w2210, y=0) -> (x = y?=w2208:bool)
                    n926 = case shown="False" w2208 {
                      tunnel: w2207 -> [w2218 _]
                      frame False {
                        n927 = local read "Transformer \nHeaders"() -> (w2217:string[])
                        n928 = call-poly <vilib>:"Write To Spreadsheet File.vi"("1D data"=w2217, "file path (dialog if empty)"=w2218) -> ()  [unwired: 6 in, 1 out]
                      }
                      frame True {
                      }
                    }
                  }
                  frame #2 {
                    # "Adds current device if it doesn't exist"
                    n929 = local read "Current \nRecord"() -> (w2223:string[])
                    n930 = Index Array(array=w2223, index=0) -> (element=w2222:string)
                    n931 = local read "Transfer Folder"() -> (w2226:path)
                    n932 = Concatenate Strings("Stats\\", "Tranformer Data.txt") -> (w2227:string)
                    n933 = local write "Current Device ID"(w2222) -> ()
                    n934 = local read "Current Device ID"() -> (w2232:string)
                    n935 = Build Path(base path=w2226, name or relative path=w2227) -> (appended path=w2225:path)
                    n936 = call-poly <vilib>:"Read From Spreadsheet File.vi"("file path (dialog if empty)"=w2225) -> ("all rows"=w2219:string[][])  [unwired: 6 in, 4 out]
                    n937 = Index Array(array=w2219, index (col)=0) -> (element=w2220:string[])  [unwired: 1 in]
                    n938 = Search 1D Array(1D array=w2220, element=w2232) -> (index of element=w2221:i32)  [unwired: 1 in]
                    n939 = Equal?(x=w2221, y=-1) -> (x = y?=w2234:bool)
                    n940 = case shown="False" w2234 {
                      tunnel: w2224 -> [w2237 w2248]
                      tunnel: w2221 -> [w2240 _]
                      tunnel: w2219 -> [w2241 _]
                      frame False {
                        n941 = local read "Current \nRecord"() -> (w2239:string[])
                        n942 = Replace Array Subset(array=w2241, new element=w2239, index (row)=w2240) -> (w2238:string[][])  [unwired: 1 in]
                        n943 = flat-sequence {
                          tunnel: w2237 -> [w2242]
                          tunnel: w2238 -> [w2243]
                          tunnel: [w2243] -> w2236
                          tunnel: [w2242] -> w2235
                          tunnel: w2236 -> [w2245]
                          tunnel: w2235 -> [w2244]
                          frame #0 {
                            n944 = Delete(path (use dialog)=w2242) -> ()  [unwired: 4 in, 3 out]
                          }
                          frame #1 {
                            n945 = call-poly <vilib>:"Write To Spreadsheet File.vi"("append to file? (new file:F)"=TRUE, "2D data"=w2245, "file path (dialog if empty)"=w2244) -> ()  [unwired: 5 in, 1 out]
                          }
                        }
                      }
                      frame True {
                        n946 = local read "Current \nRecord"() -> (w2247:string[])
                        n947 = call-poly <vilib>:"Write To Spreadsheet File.vi"("append to file? (new file:F)"=TRUE, "1D data"=w2247, "file path (dialog if empty)"=w2248) -> ()  [unwired: 5 in, 1 out]
                      }
                    }
                  }
                }
                n948 = Path To String(path=w1757) -> (string=w1755:string)
                n949 = stacked-sequence {
                  tunnel: [_ _ _ _ _ _ _ _ _ _ _ _ w2167] -> w1737
                  tunnel: w1736 -> [w1759 _ _ _ _ _ _ _ _ _ _ _ _]
                  frame #0 {
                    n950 = call-poly <vilib>:"Read From Spreadsheet File.vi"("file path (dialog if empty)"=w1759) -> ("all rows"=w1758:string[][])  [unwired: 6 in, 4 out]
                    n951 = Array Size(array=w1758) -> (size(s)=w1763:i32[])
                    n952 = Array Subset(array=w1758, index (row)=0, index (col)=0, length (col)=3) -> (w1767:string[][])  [unwired: 1 in]
                    n953 = Index Array(array=w1763, index=0) -> (element=w1761:i32)
                    n954 = Reshape Array(w1767, w1761) -> (w1760:string[])
                    n955 = Search 1D Array(1D array=w1760, element="Dielectric (nm):") -> (index of element=w1770:i32)  [unwired: 1 in]
                    n956 = Equal?(x=w1770, y=-1) -> (x = y?=w1769:bool)
                    n957 = case shown="False" w1769 {
                      tunnel: w1758 -> [w1778 w1782]
                      tunnel: w1770 -> [w1774 _]
                      tunnel: [w1773 w1782] -> w1768
                      frame False {
                        n958 = local read "New: Dielectric"() -> (w1780:dbl)
                        n959 = Number To Fractional String(number=w1780) -> (F-format string=w1775:string)  [unwired: 3 in]
                        n960 = Divide(x=w1774, y=3) -> (x/y=w1777:dbl)
                        n961 = To Word Integer(number=w1777) -> (16bit integer=w1776:i16)
                        n962 = Replace Array Subset(array=w1778, new element=w1775, index (row)=w1776, index (col)=1) -> (w1773:string[][])
                      }
                      frame True {
                      }
                    }
                    n963 = local write "Save1 Array"(w1768) -> ()
                  }
                  frame #1 {
                    n964 = local read "Save1 Array"() -> (w1784:string[][])
                    n965 = Array Size(array=w1784) -> (size(s)=w1787:i32[])
                    n966 = Array Subset(array=w1784, index (row)=0, index (col)=0, length (col)=3) -> (w1791:string[][])  [unwired: 1 in]
                    n967 = Index Array(array=w1787, index=0) -> (element=w1785:i32)
                    n968 = Reshape Array(w1791, w1785) -> (w1783:string[])
                    n969 = Search 1D Array(1D array=w1783, element="Length (um):") -> (index of element=w1794:i32)  [unwired: 1 in]
                    n970 = Equal?(x=w1794, y=-1) -> (x = y?=w1793:bool)
                    n971 = case shown="False" w1793 {
                      tunnel: w1784 -> [w1804 w1807]
                      tunnel: w1794 -> [w1801 _]
                      tunnel: [w1800 w1807] -> w1792
                      frame False {
                        n972 = local read "New: Length"() -> (w1797:dbl)
                        n973 = Divide(x=w1801, y=3) -> (x/y=w1803:dbl)
                        n974 = Format Value(format string="%#g", value (0)=w1797) -> (output string=w1798:string)  [unwired: 1 in]
                        n975 = To Word Integer(number=w1803) -> (16bit integer=w1802:i16)
                        n976 = Replace Array Subset(array=w1804, new element=w1798, index (row)=w1802, index (col)=1) -> (w1800:string[][])
                      }
                      frame True {
                      }
                    }
                    n977 = local write "Save1 Array"(w1792) -> ()
                  }
                  frame #2 {
                    n978 = local read "Save1 Array"() -> (w1809:string[][])
                    n979 = Array Size(array=w1809) -> (size(s)=w1814:i32[])
                    n980 = Array Subset(array=w1809, index (row)=0, index (col)=0, length (col)=3) -> (w1810:string[][])  [unwired: 1 in]
                    n981 = Index Array(array=w1814, index=0) -> (element=w1816:i32)
                    n982 = Reshape Array(w1810, w1816) -> (w1808:string[])
                    n983 = Search 1D Array(1D array=w1808, element="Width (um):") -> (index of element=w1819:i32)  [unwired: 1 in]
                    n984 = Equal?(x=w1819, y=-1) -> (x = y?=w1818:bool)
                    n985 = case shown="False" w1818 {
                      tunnel: w1819 -> [w1827 _]
                      tunnel: w1809 -> [w1826 w1832]
                      tunnel: [w1825 w1832] -> w1817
                      frame False {
                        n986 = local read "New: Width"() -> (w1822:dbl)
                        n987 = Divide(x=w1827, y=3) -> (x/y=w1829:dbl)
                        n988 = To Word Integer(number=w1829) -> (16bit integer=w1828:i16)
                        n989 = Format Value(format string="%#g", value (0)=w1822) -> (output string=w1823:string)  [unwired: 1 in]
                        n990 = Replace Array Subset(array=w1826, new element=w1823, index (row)=w1828, index (col)=1) -> (w1825:string[][])
                      }
                      frame True {
                      }
                    }
                    n991 = local write "Save1 Array"(w1817) -> ()
                  }
                  frame #3 {
                    w1842 = "Sample Temp (K):"
                    n992 = local read "Save1 Array"() -> (w1834:string[][])
                    n993 = Array Size(array=w1834) -> (size(s)=w1839:i32[])
                    n994 = Array Subset(array=w1834, index (row)=0, index (col)=0, length (col)=3) -> (w1835:string[][])  [unwired: 1 in]
                    n995 = Index Array(array=w1839, index=0) -> (element=w1841:i32)
                    n996 = Reshape Array(w1835, w1841) -> (w1833:string[])
                    n997 = Search 1D Array(1D array=w1833, element=w1842) -> (index of element=w1845:i32)  [unwired: 1 in]
                    n998 = Equal?(x=w1845, y=-1) -> (x = y?=w1844:bool)
                    n999 = case shown="True" w1844 {
                      tunnel: w1834 -> [w1854 w1868]
                      tunnel: w1845 -> [w1851 _]
                      tunnel: [w1850 w1867] -> w1843
                      tunnel: w1833 -> [_ w1870]
                      tunnel: w1842 -> [_ w1857]
                      frame False {
                        n1000 = local read "New: Temp"() -> (w1848:dbl)
                        n1001 = Divide(x=w1851, y=3) -> (x/y=w1853:dbl)
                        n1002 = Format Value(format string="%#g", value (0)=w1848) -> (output string=w1847:string)  [unwired: 1 in]
                        n1003 = To Word Integer(number=w1853) -> (16bit integer=w1852:i16)
                        n1004 = Replace Array Subset(array=w1854, new element=w1847, index (row)=w1852, index (col)=1) -> (w1850:string[][])
                      }
                      frame True {
                        n1005 = local read "New: Temp"() -> (w1859:dbl)
                        n1006 = Search 1D Array(1D array=w1870, element="Width (um):") -> (index of element=w1864:i32)  [unwired: 1 in]
                        n1007 = Divide(x=w1864, y=3) -> (x/y=w1865:dbl)
                        n1008 = To Word Integer(number=w1865) -> (16bit integer=w1863:i16)
                        n1009 = Format Value(format string="%#g", value (0)=w1859) -> (output string=w1858:string)  [unwired: 1 in]
                        n1010 = Build Array(w1857, w1858) -> (w1861:string[])
                        n1011 = Increment(x=w1863) -> (x+1=w1862:i16)
                        n1012 = Insert Into Array(array=w1868, index (row)=w1862, new element=w1861) -> (w1867:string[][])  [unwired: 1 in]
                      }
                    }
                    n1013 = local write "Save1 Array"(w1843) -> ()
                  }
                  frame #4 {
                    w1880 = "Mobility-Sat (cm^2/Vs):"
                    n1014 = local read "Save1 Array"() -> (w1872:string[][])
                    n1015 = Array Size(array=w1872) -> (size(s)=w1877:i32[])
                    n1016 = Array Subset(array=w1872, index (row)=0, index (col)=0, length (col)=3) -> (w1873:string[][])  [unwired: 1 in]
                    n1017 = Index Array(array=w1877, index=0) -> (element=w1879:i32)
                    n1018 = Reshape Array(w1873, w1879) -> (w1871:string[])
                    n1019 = Search 1D Array(1D array=w1871, element=w1880) -> (index of element=w1883:i32)  [unwired: 1 in]
                    n1020 = Equal?(x=w1883, y=-1) -> (x = y?=w1882:bool)
                    n1021 = case shown="True" w1882 {
                      tunnel: w1872 -> [w1892 w1900]
                      tunnel: w1883 -> [w1889 _]
                      tunnel: [w1888 w1899] -> w1881
                      tunnel: w1871 -> [_ w1897]
                      tunnel: w1880 -> [_ w1895]
                      frame False {
                        n1022 = local read "New: Mobility-Sat"() -> (w1885:dbl)
                        n1023 = Divide(x=w1889, y=3) -> (x/y=w1891:dbl)
                        n1024 = To Word Integer(number=w1891) -> (16bit integer=w1890:i16)
                        n1025 = Format Value(format string="%#g", value (0)=w1885) -> (output string=w1886:string)  [unwired: 1 in]
                        n1026 = Replace Array Subset(array=w1892, new element=w1886, index (row)=w1890, index (col)=1) -> (w1888:string[][])
                      }
                      frame True {
                        n1027 = local read "New: Mobility-Sat"() -> (w1901:dbl)
                        n1028 = Search 1D Array(1D array=w1897, element="Mobility (cm^2/Vs):") -> (index of element=w1904:i32)  [unwired: 1 in]
                        n1029 = Divide(x=w1904, y=3) -> (x/y=w1905:dbl)
                        n1030 = To Word Integer(number=w1905) -> (16bit integer=w1896:i16)
                        n1031 = Format Value(format string="%#g", value (0)=w1901) -> (output string=w1898:string)  [unwired: 1 in]
                        n1032 = Build Array(w1895, w1898) -> (w1903:string[])
                        n1033 = Replace Array Subset(array=w1900, new element=w1903, index (row)=w1896) -> (w1899:string[][])  [unwired: 1 in]
                      }
                    }
                    n1034 = local write "Save1 Array"(w1881) -> ()
                  }
                  frame #5 {
                    w1917 = "Mobility-Lin (cm^2/Vs):"
                    n1035 = local read "Save1 Array"() -> (w1908:string[][])
                    n1036 = Array Size(array=w1908) -> (size(s)=w1914:i32[])
                    n1037 = Array Subset(array=w1908, index (row)=0, index (col)=0, length (col)=3) -> (w1910:string[][])  [unwired: 1 in]
                    n1038 = Index Array(array=w1914, index=0) -> (element=w1916:i32)
                    n1039 = Reshape Array(w1910, w1916) -> (w1909:string[])
                    n1040 = Search 1D Array(1D array=w1909, element=w1917) -> (index of element=w1920:i32)  [unwired: 1 in]
                    n1041 = Equal?(x=w1920, y=-1) -> (x = y?=w1919:bool)
                    n1042 = case shown="True" w1919 {
                      tunnel: w1908 -> [w1929 w1935]
                      tunnel: w1920 -> [w1926 _]
                      tunnel: [w1925 w1934] -> w1918
                      tunnel: w1909 -> [_ w1933]
                      tunnel: w1917 -> [_ w1932]
                      frame False {
                        n1043 = local read "Calc: Mobility-Lin"() -> (w1922:dbl)
                        n1044 = Divide(x=w1926, y=3) -> (x/y=w1928:dbl)
                        n1045 = To Word Integer(number=w1928) -> (16bit integer=w1927:i16)
                        n1046 = Format Value(format string="%#g", value (0)=w1922) -> (output string=w1923:string)  [unwired: 1 in]
                        n1047 = Replace Array Subset(array=w1929, new element=w1923, index (row)=w1927, index (col)=1) -> (w1925:string[][])
                      }
                      frame True {
                        n1048 = local read "Calc: Mobility-Lin"() -> (w1936:dbl)
                        n1049 = Search 1D Array(1D array=w1933, element="Mobility-Sat (cm^2/Vs):") -> (index of element=w1941:i32)  [unwired: 1 in]
                        n1050 = Divide(x=w1941, y=3) -> (x/y=w1942:dbl)
                        n1051 = To Word Integer(number=w1942) -> (16bit integer=w1940:i16)
                        n1052 = Format Value(format string="%#g", value (0)=w1936) -> (output string=w1945:string)  [unwired: 1 in]
                        n1053 = Build Array(w1932, w1945) -> (w1938:string[])
                        n1054 = Increment(x=w1940) -> (x+1=w1939:i16)
                        n1055 = Insert Into Array(array=w1935, index (row)=w1939, new element=w1938) -> (w1934:string[][])  [unwired: 1 in]
                      }
                    }
                    n1056 = local write "Save1 Array"(w1918) -> ()
                  }
                  frame #6 {
                    w1955 = "On/Off I-Sat:"
                    n1057 = local read "Save1 Array"() -> (w1946:string[][])
                    n1058 = Array Size(array=w1946) -> (size(s)=w1952:i32[])
                    n1059 = Array Subset(array=w1946, index (row)=0, index (col)=0, length (col)=3) -> (w1948:string[][])  [unwired: 1 in]
                    n1060 = Index Array(array=w1952, index=0) -> (element=w1954:i32)
                    n1061 = Reshape Array(w1948, w1954) -> (w1947:string[])
                    n1062 = Search 1D Array(1D array=w1947, element=w1955) -> (index of element=w1958:i32)  [unwired: 1 in]
                    n1063 = Equal?(x=w1958, y=-1) -> (x = y?=w1957:bool)
                    n1064 = case shown="True" w1957 {
                      tunnel: w1946 -> [w1967 w1974]
                      tunnel: w1958 -> [w1964 _]
                      tunnel: [w1963 w1975] -> w1956
                      tunnel: w1947 -> [_ w1972]
                      tunnel: w1955 -> [_ w1970]
                      frame False {
                        n1065 = local read "Calc: On/Off"() -> (w1960:dbl)
                        n1066 = Divide(x=w1964, y=3) -> (x/y=w1966:dbl)
                        n1067 = To Word Integer(number=w1966) -> (16bit integer=w1965:i16)
                        n1068 = Format Value(format string="%#g", value (0)=w1960) -> (output string=w1961:string)  [unwired: 1 in]
                        n1069 = Replace Array Subset(array=w1967, new element=w1961, index (row)=w1965, index (col)=1) -> (w1963:string[][])
                      }
                      frame True {
                        n1070 = local read "Calc: On/Off"() -> (w1976:dbl)
                        n1071 = Search 1D Array(1D array=w1972, element="On/Off Current:") -> (index of element=w1979:i32)  [unwired: 1 in]
                        n1072 = Divide(x=w1979, y=3) -> (x/y=w1980:dbl)
                        n1073 = To Word Integer(number=w1980) -> (16bit integer=w1971:i16)
                        n1074 = Format Value(format string="%#g", value (0)=w1976) -> (output string=w1973:string)  [unwired: 1 in]
                        n1075 = Build Array(w1970, w1973) -> (w1978:string[])
                        n1076 = Replace Array Subset(array=w1974, new element=w1978, index (row)=w1971) -> (w1975:string[][])  [unwired: 1 in]
                      }
                    }
                    n1077 = local write "Save1 Array"(w1956) -> ()
                  }
                  frame #7 {
                    w1992 = "Off I-Sat (A):"
                    n1078 = local read "Save1 Array"() -> (w1983:string[][])
                    n1079 = Array Size(array=w1983) -> (size(s)=w1989:i32[])
                    n1080 = Array Subset(array=w1983, index (row)=0, index (col)=0, length (col)=3) -> (w1985:string[][])  [unwired: 1 in]
                    n1081 = Index Array(array=w1989, index=0) -> (element=w1991:i32)
                    n1082 = Reshape Array(w1985, w1991) -> (w1984:string[])
                    n1083 = Search 1D Array(1D array=w1984, element=w1992) -> (index of element=w1995:i32)  [unwired: 1 in]
                    n1084 = Equal?(x=w1995, y=-1) -> (x = y?=w1994:bool)
                    n1085 = case shown="True" w1994 {
                      tunnel: w1983 -> [w2004 w2010]
                      tunnel: w1995 -> [w2001 _]
                      tunnel: [w2000 w2009] -> w1993
                      tunnel: w1984 -> [_ w2008]
                      tunnel: w1992 -> [_ w2007]
                      frame False {
                        n1086 = local read "Calc: Off I-Sat"() -> (w1999:dbl)
                        n1087 = Divide(x=w2001, y=3) -> (x/y=w2003:dbl)
                        n1088 = Format Value(format string="%#g", value (0)=w1999) -> (output string=w1997:string)  [unwired: 1 in]
                        n1089 = To Word Integer(number=w2003) -> (16bit integer=w2002:i16)
                        n1090 = Replace Array Subset(array=w2004, new element=w1997, index (row)=w2002, index (col)=1) -> (w2000:string[][])
                      }
                      frame True {
                        n1091 = local read "Calc: Off I-Sat"() -> (w2011:dbl)
                        n1092 = Search 1D Array(1D array=w2008, element="On/Off I-Sat:") -> (index of element=w2016:i32)  [unwired: 1 in]
                        n1093 = Divide(x=w2016, y=3) -> (x/y=w2017:dbl)
                        n1094 = To Word Integer(number=w2017) -> (16bit integer=w2015:i16)
                        n1095 = Format Value(format string="%#g", value (0)=w2011) -> (output string=w2020:string)  [unwired: 1 in]
                        n1096 = Build Array(w2007, w2020) -> (w2013:string[])
                        n1097 = Increment(x=w2015) -> (x+1=w2014:i16)
                        n1098 = Insert Into Array(array=w2010, index (row)=w2014, new element=w2013) -> (w2009:string[][])  [unwired: 1 in]
                      }
                    }
                    n1099 = local write "Save1 Array"(w1993) -> ()
                  }
                  frame #8 {
                    w2022 = "Vt-Sat (V):"
                    n1100 = local read "Save1 Array"() -> (w2023:string[][])
                    n1101 = Array Size(array=w2023) -> (size(s)=w2028:i32[])
                    n1102 = Array Subset(array=w2023, index (row)=0, index (col)=0, length (col)=3) -> (w2024:string[][])  [unwired: 1 in]
                    n1103 = Index Array(array=w2028, index=0) -> (element=w2030:i32)
                    n1104 = Reshape Array(w2024, w2030) -> (w2021:string[])
                    n1105 = Search 1D Array(1D array=w2021, element=w2022) -> (index of element=w2033:i32)  [unwired: 1 in]
                    n1106 = Equal?(x=w2033, y=-1) -> (x = y?=w2032:bool)
                    n1107 = case shown="True" w2032 {
                      tunnel: w2023 -> [w2040 w2049]
                      tunnel: w2033 -> [w2036 _]
                      tunnel: [w2035 w2048] -> w2031
                      tunnel: w2022 -> [_ w2047]
                      tunnel: w2021 -> [_ w2046]
                      frame False {
                        n1108 = local read "New: VT-Sat"() -> (w2042:dbl)
                        n1109 = Number To Fractional String(number=w2042) -> (F-format string=w2037:string)  [unwired: 3 in]
                        n1110 = Divide(x=w2036, y=3) -> (x/y=w2039:dbl)
                        n1111 = To Word Integer(number=w2039) -> (16bit integer=w2038:i16)
                        n1112 = Replace Array Subset(array=w2040, new element=w2037, index (row)=w2038, index (col)=1) -> (w2035:string[][])
                      }
                      frame True {
                        n1113 = local read "New: VT-Sat"() -> (w2050:dbl)
                        n1114 = Search 1D Array(1D array=w2046, element="Threshold V (V):") -> (index of element=w2045:i32)  [unwired: 1 in]
                        n1115 = Divide(x=w2045, y=3) -> (x/y=w2053:dbl)
                        n1116 = To Word Integer(number=w2053) -> (16bit integer=w2044:i16)
                        n1117 = Format Value(format string="%#g", value (0)=w2050) -> (output string=w2056:string)  [unwired: 1 in]
                        n1118 = Build Array(w2047, w2056) -> (w2052:string[])
                        n1119 = Replace Array Subset(array=w2049, new element=w2052, index (row)=w2044) -> (w2048:string[][])  [unwired: 1 in]
                      }
                    }
                    n1120 = local write "Save1 Array"(w2031) -> ()
                  }
                  frame #9 {
                    n1121 = local read "Save1 Array"() -> (w2057:string[][])
                    n1122 = Array Size(array=w2057) -> (size(s)=w2063:i32[])
                    n1123 = Array Subset(array=w2057, index (row)=0, index (col)=0, length (col)=3) -> (w2059:string[][])  [unwired: 1 in]
                    n1124 = Index Array(array=w2063, index=0) -> (element=w2065:i32)
                    n1125 = Reshape Array(w2059, w2065) -> (w2058:string[])
                    n1126 = Search 1D Array(1D array=w2058, element="VT-Lin (V):") -> (index of element=w2068:i32)  [unwired: 1 in]
                    n1127 = Equal?(x=w2068, y=-1) -> (x = y?=w2067:bool)
                    n1128 = case shown="False" w2067 {
                      tunnel: w2057 -> [w2078 w2081]
                      tunnel: w2068 -> [w2075 _]
                      tunnel: [w2074 w2081] -> w2066
                      frame False {
                        n1129 = local read "New: VT-Lin"() -> (w2072:dbl)
                        n1130 = Divide(x=w2075, y=3) -> (x/y=w2077:dbl)
                        n1131 = Format Value(format string="%#g", value (0)=w2072) -> (output string=w2071:string)  [unwired: 1 in]
                        n1132 = To Word Integer(number=w2077) -> (16bit integer=w2076:i16)
                        n1133 = Replace Array Subset(array=w2078, new element=w2071, index (row)=w2076, index (col)=1) -> (w2074:string[][])
                      }
                      frame True {
                      }
                    }
                    n1134 = local write "Save1 Array"(w2066) -> ()
                  }
                  frame #10 {
                    w2082 = "STS-Sat (V/decade):"
                    n1135 = local read "Save1 Array"() -> (w2084:string[][])
                    n1136 = Array Size(array=w2084) -> (size(s)=w2089:i32[])
                    n1137 = Array Subset(array=w2084, index (row)=0, index (col)=0, length (col)=3) -> (w2085:string[][])  [unwired: 1 in]
                    n1138 = Index Array(array=w2089, index=0) -> (element=w2091:i32)
                    n1139 = Reshape Array(w2085, w2091) -> (w2083:string[])
                    n1140 = Search 1D Array(1D array=w2083, element=w2082) -> (index of element=w2094:i32)  [unwired: 1 in]
                    n1141 = Equal?(x=w2094, y=-1) -> (x = y?=w2093:bool)
                    n1142 = case shown="True" w2093 {
                      tunnel: w2084 -> [w2103 w2109]
                      tunnel: w2094 -> [w2100 _]
                      tunnel: [w2099 w2110] -> w2092
                      tunnel: w2083 -> [_ w2108]
                      tunnel: w2082 -> [_ w2107]
                      frame False {
                        n1143 = local read "New: STS"() -> (w2097:dbl)
                        n1144 = Divide(x=w2100, y=3) -> (x/y=w2102:dbl)
                        n1145 = Format Value(format string="%#g", value (0)=w2097) -> (output string=w2096:string)  [unwired: 1 in]
                        n1146 = To Word Integer(number=w2102) -> (16bit integer=w2101:i16)
                        n1147 = Replace Array Subset(array=w2103, new element=w2096, index (row)=w2101, index (col)=1) -> (w2099:string[][])
                      }
                      frame True {
                        n1148 = local read "New: STS"() -> (w2111:dbl)
                        n1149 = Search 1D Array(1D array=w2108, element="S.T.S. (V/decade):") -> (index of element=w2114:i32)  [unwired: 1 in]
                        n1150 = Divide(x=w2114, y=3) -> (x/y=w2115:dbl)
                        n1151 = To Word Integer(number=w2115) -> (16bit integer=w2106:i16)
                        n1152 = Format Value(format string="%#g", value (0)=w2111) -> (output string=w2118:string)  [unwired: 1 in]
                        n1153 = Build Array(w2107, w2118) -> (w2113:string[])
                        n1154 = Replace Array Subset(array=w2109, new element=w2113, index (row)=w2106) -> (w2110:string[][])  [unwired: 1 in]
                      }
                    }
                    n1155 = local write "Save1 Array"(w2092) -> ()
                  }
                  frame #11 {
                    w2119 = "Trap Density-VT (Traps/Vcm^2):"
                    n1156 = local read "Save1 Array"() -> (w2121:string[][])
                    n1157 = Array Size(array=w2121) -> (size(s)=w2126:i32[])
                    n1158 = Array Subset(array=w2121, index (row)=0, index (col)=0, length (col)=3) -> (w2122:string[][])  [unwired: 1 in]
                    n1159 = Index Array(array=w2126, index=0) -> (element=w2128:i32)
                    n1160 = Reshape Array(w2122, w2128) -> (w2120:string[])
                    n1161 = Search 1D Array(1D array=w2120, element=w2119) -> (index of element=w2131:i32)  [unwired: 1 in]
                    n1162 = Equal?(x=w2131, y=-1) -> (x = y?=w2130:bool)
                    n1163 = case shown="True" w2130 {
                      tunnel: w2121 -> [w2140 w2145]
                      tunnel: w2131 -> [w2136 _]
                      tunnel: [w2135 w2146] -> w2129
                      tunnel: w2120 -> [_ w2144]
                      tunnel: w2119 -> [_ w2143]
                      frame False {
                        n1164 = local read "New: Trap Density-VT"() -> (w2134:dbl)
                        n1165 = Format Value(format string="%#g", value (0)=w2134) -> (output string=w2137:string)  [unwired: 1 in]
                        n1166 = Divide(x=w2136, y=3) -> (x/y=w2139:dbl)
                        n1167 = To Word Integer(number=w2139) -> (16bit integer=w2138:i16)
                        n1168 = Replace Array Subset(array=w2140, new element=w2137, index (row)=w2138, index (col)=1) -> (w2135:string[][])
                      }
                      frame True {
                        n1169 = local read "New: Trap Density-VT"() -> (w2156:dbl)
                        n1170 = Search 1D Array(1D array=w2144, element="STS-Sat (V/decade):") -> (index of element=w2151:i32)  [unwired: 1 in]
                        n1171 = Divide(x=w2151, y=3) -> (x/y=w2150:dbl)
                        n1172 = To Word Integer(number=w2150) -> (16bit integer=w2152:i16)
                        n1173 = Format Value(format string="%#g", value (0)=w2156) -> (output string=w2147:string)  [unwired: 1 in]
                        n1174 = Build Array(w2143, w2147) -> (w2154:string[])
                        n1175 = Increment(x=w2152) -> (x+1=w2153:i16)
                        n1176 = Insert Into Array(array=w2145, index (row)=w2153, new element=w2154) -> (w2146:string[][])  [unwired: 1 in]
                      }
                    }
                    n1177 = local write "Save1 Array"(w2129) -> ()
                  }
                  frame #12 {
                    w2157 = "Trap Density-STS (Traps/Vcm^2):"
                    n1178 = local read "Save1 Array"() -> (w2159:string[][])
                    n1179 = Array Size(array=w2159) -> (size(s)=w2164:i32[])
                    n1180 = Array Subset(array=w2159, index (row)=0, index (col)=0, length (col)=3) -> (w2160:string[][])  [unwired: 1 in]
                    n1181 = Index Array(array=w2164, index=0) -> (element=w2166:i32)
                    n1182 = Reshape Array(w2160, w2166) -> (w2158:string[])
                    n1183 = Search 1D Array(1D array=w2158, element=w2157) -> (index of element=w2169:i32)  [unwired: 1 in]
                    n1184 = Equal?(x=w2169, y=-1) -> (x = y?=w2168:bool)
                    n1185 = case shown="True" w2168 {
                      tunnel: w2159 -> [w2178 w2183]
                      tunnel: w2169 -> [w2175 _]
                      tunnel: [w2174 w2184] -> w2167
                      tunnel: w2158 -> [_ w2182]
                      tunnel: w2157 -> [_ w2181]
                      frame False {
                        n1186 = local read "New: Trap Density-STS"() -> (w2172:dbl)
                        n1187 = Divide(x=w2175, y=3) -> (x/y=w2177:dbl)
                        n1188 = To Word Integer(number=w2177) -> (16bit integer=w2176:i16)
                        n1189 = Format Value(format string="%#g", value (0)=w2172) -> (output string=w2171:string)  [unwired: 1 in]
                        n1190 = Replace Array Subset(array=w2178, new element=w2171, index (row)=w2176, index (col)=1) -> (w2174:string[][])
                      }
                      frame True {
                        n1191 = local read "New: Trap Density-STS"() -> (w2185:dbl)
                        n1192 = Search 1D Array(1D array=w2182, element="Trap Density-VT (Traps/Vcm^2):") -> (index of element=w2190:i32)  [unwired: 1 in]
                        n1193 = Divide(x=w2190, y=3) -> (x/y=w2191:dbl)
                        n1194 = To Word Integer(number=w2191) -> (16bit integer=w2189:i16)
                        n1195 = Format Value(format string="%#g", value (0)=w2185) -> (output string=w2194:string)  [unwired: 1 in]
                        n1196 = Build Array(w2181, w2194) -> (w2187:string[])
                        n1197 = Increment(x=w2189) -> (x+1=w2188:i16)
                        n1198 = Insert Into Array(array=w2183, index (row)=w2188, new element=w2187) -> (w2184:string[][])  [unwired: 1 in]
                      }
                    }
                    n1199 = local write "Save1 Array"(w2167) -> ()
                  }
                }
                n1200 = Concatenate Strings(w1755, "\\", w1753) -> (w1754:string)
                n1201 = String To Path(string=w1754) -> (path=w1744:path)
                n1202 = disable-structure shown="Disabled" {
                  frame Disabled {
                  }
                  frame Enabled {
                  }
                }
              }
              frame #1 {
                n1203 = Equal?(x=w2253, y=w2250) -> (x = y?=w2252:bool)
                n1204 = case shown="False" w2252 {
                  tunnel: w2253 -> [w2256 _]
                  tunnel: w2250 -> [w2255 _]
                  frame False {
                    n1205 = Move(source path=w2256, 9:TRUE, 10:w2255) -> ()  [unwired: 2 in, 3 out]
                  }
                  frame True {
                  }
                }
              }
              frame #2 {
                n1206 = local write "Transfer File"(w2257) -> ()
                n1207 = call-poly <vilib>:"Write To Spreadsheet File.vi"("2D data"=w2258, "file path (dialog if empty)"=w2257) -> ()  [unwired: 6 in, 1 out]
              }
            }
          }
          event "Save Changes? 2": Mouse Down {
            n1208 = event-data() -> ()  [unwired: 1 in, 5 out]
            n1209 = stacked-sequence {
              seq-local: [w2316 _ _ _ _] -> [_ w2776 _ _ _]
              seq-local: [w2315 _ _ _ _] -> [_ w2777 _ _ _]
              seq-local: [w2315 _ _ _ _] -> [_ w2775 _ _ _]
              seq-local: [w2317 _ _ _ _] -> [_ w2773 _ _ _]
              seq-local: [_ w2777 _ _ _] -> [_ _ w2782 _ _]
              seq-local: [_ w2773 _ _ _] -> [_ _ w2781 _ _]
              frame #0 {
                n1210 = local read "Transfer File"() -> (w2316:path)
                n1211 = local read "New: Temp"() -> (w2319:dbl)
                n1212 = local read "New: Length"() -> (w2322:dbl)
                n1213 = local read "New: Width"() -> (w2320:dbl)
                n1214 = To Word Integer(number=w2319) -> (16bit integer=w2318:i16)
                n1215 = Number To Decimal String(number=w2318) -> (decimal integer string=w2326:string)  [unwired: 1 in]
                n1216 = To Single Precision Float(number=w2320) -> (single precision float=w2321:sgl)
                n1217 = To Single Precision Float(number=w2322) -> (single precision float=w2323:sgl)
                n1218 = local read "Index"() -> (w2330:string)
                n1219 = Strip Path(path=w2316) -> (stripped path=w2335:path)  [unwired: 1 out]
                n1220 = Number To Decimal String(number=w2323) -> (decimal integer string=w2328:string)  [unwired: 1 in]
                n1221 = Number To Decimal String(number=w2321) -> (decimal integer string=w2329:string)  [unwired: 1 in]
                n1222 = Concatenate Strings("_", w2326, "K") -> (w2324:string)
                n1223 = call "Build Text2"("Temp"=w2324, "Index"=w2330, "Length"=w2328, "Width"=w2329) -> ("Result"=w2331:string)  [unwired: 10 in, 1 out]
                n1224 = Path To String(path=w2335) -> (string=w2333:string)
                n1225 = Concatenate Strings(w2333, "\\", w2331) -> (w2332:string)
                n1226 = stacked-sequence {
                  tunnel: [_ _ _ _ _ _ _ _ _ _ _ _ w2735] -> _
                  tunnel: w2316 -> [w2337 _ _ _ _ _ _ _ _ _ _ _ _]
                  tunnel: [_ _ _ _ _ _ _ _ _ _ _ _ w2735] -> w2317
                  frame #0 {
                    n1227 = call-poly <vilib>:"Read From Spreadsheet File.vi"("file path (dialog if empty)"=w2337) -> ("all rows"=w2336:string[][])  [unwired: 6 in, 4 out]
                    n1228 = Array Size(array=w2336) -> (size(s)=w2341:i32[])
                    n1229 = Array Subset(array=w2336, index (row)=0, index (col)=0, length (col)=3) -> (w2345:string[][])  [unwired: 1 in]
                    n1230 = Index Array(array=w2341, index=0) -> (element=w2339:i32)
                    n1231 = Reshape Array(w2345, w2339) -> (w2338:string[])
                    n1232 = Search 1D Array(1D array=w2338, element="Dielectric (nm):") -> (index of element=w2348:i32)  [unwired: 1 in]
                    n1233 = Equal?(x=w2348, y=-1) -> (x = y?=w2347:bool)
                    n1234 = case shown="False" w2347 {
                      tunnel: w2336 -> [w2356 w2360]
                      tunnel: w2348 -> [w2352 _]
                      tunnel: [w2351 w2360] -> w2346
                      frame False {
                        n1235 = local read "New: Dielectric"() -> (w2358:dbl)
                        n1236 = Number To Fractional String(number=w2358) -> (F-format string=w2353:string)  [unwired: 3 in]
                        n1237 = Divide(x=w2352, y=3) -> (x/y=w2355:dbl)
                        n1238 = To Word Integer(number=w2355) -> (16bit integer=w2354:i16)
                        n1239 = Replace Array Subset(array=w2356, new element=w2353, index (row)=w2354, index (col)=1) -> (w2351:string[][])
                      }
                      frame True {
                      }
                    }
                    n1240 = local write "Save1 Array"(w2346) -> ()
                  }
                  frame #1 {
                    n1241 = local read "Save1 Array"() -> (w2362:string[][])
                    n1242 = Array Size(array=w2362) -> (size(s)=w2365:i32[])
                    n1243 = Array Subset(array=w2362, index (row)=0, index (col)=0, length (col)=3) -> (w2369:string[][])  [unwired: 1 in]
                    n1244 = Index Array(array=w2365, index=0) -> (element=w2363:i32)
                    n1245 = Reshape Array(w2369, w2363) -> (w2361:string[])
                    n1246 = Search 1D Array(1D array=w2361, element="Length (um):") -> (index of element=w2372:i32)  [unwired: 1 in]
                    n1247 = Equal?(x=w2372, y=-1) -> (x = y?=w2371:bool)
                    n1248 = case shown="False" w2371 {
                      tunnel: w2362 -> [w2382 w2385]
                      tunnel: w2372 -> [w2379 _]
                      tunnel: [w2378 w2385] -> w2370
                      frame False {
                        n1249 = local read "New: Length"() -> (w2375:dbl)
                        n1250 = Divide(x=w2379, y=3) -> (x/y=w2381:dbl)
                        n1251 = Format Value(format string="%#g", value (0)=w2375) -> (output string=w2376:string)  [unwired: 1 in]
                        n1252 = To Word Integer(number=w2381) -> (16bit integer=w2380:i16)
                        n1253 = Replace Array Subset(array=w2382, new element=w2376, index (row)=w2380, index (col)=1) -> (w2378:string[][])
                      }
                      frame True {
                      }
                    }
                    n1254 = local write "Save1 Array"(w2370) -> ()
                  }
                  frame #2 {
                    n1255 = local read "Save1 Array"() -> (w2387:string[][])
                    n1256 = Array Size(array=w2387) -> (size(s)=w2392:i32[])
                    n1257 = Array Subset(array=w2387, index (row)=0, index (col)=0, length (col)=3) -> (w2388:string[][])  [unwired: 1 in]
                    n1258 = Index Array(array=w2392, index=0) -> (element=w2394:i32)
                    n1259 = Reshape Array(w2388, w2394) -> (w2386:string[])
                    n1260 = Search 1D Array(1D array=w2386, element="Width (um):") -> (index of element=w2397:i32)  [unwired: 1 in]
                    n1261 = Equal?(x=w2397, y=-1) -> (x = y?=w2396:bool)
                    n1262 = case shown="False" w2396 {
                      tunnel: w2397 -> [w2405 _]
                      tunnel: w2387 -> [w2404 w2410]
                      tunnel: [w2403 w2410] -> w2395
                      frame False {
                        n1263 = local read "New: Width"() -> (w2400:dbl)
                        n1264 = Divide(x=w2405, y=3) -> (x/y=w2407:dbl)
                        n1265 = To Word Integer(number=w2407) -> (16bit integer=w2406:i16)
                        n1266 = Format Value(format string="%#g", value (0)=w2400) -> (output string=w2401:string)  [unwired: 1 in]
                        n1267 = Replace Array Subset(array=w2404, new element=w2401, index (row)=w2406, index (col)=1) -> (w2403:string[][])
                      }
                      frame True {
                      }
                    }
                    n1268 = local write "Save1 Array"(w2395) -> ()
                  }
                  frame #3 {
                    w2420 = "Sample Temp (K):"
                    n1269 = local read "Save1 Array"() -> (w2412:string[][])
                    n1270 = Array Size(array=w2412) -> (size(s)=w2417:i32[])
                    n1271 = Array Subset(array=w2412, index (row)=0, index (col)=0, length (col)=3) -> (w2413:string[][])  [unwired: 1 in]
                    n1272 = Index Array(array=w2417, index=0) -> (element=w2419:i32)
                    n1273 = Reshape Array(w2413, w2419) -> (w2411:string[])
                    n1274 = Search 1D Array(1D array=w2411, element=w2420) -> (index of element=w2423:i32)  [unwired: 1 in]
                    n1275 = Equal?(x=w2423, y=-1) -> (x = y?=w2422:bool)
                    n1276 = case shown="True" w2422 {
                      tunnel: w2412 -> [w2432 w2446]
                      tunnel: w2423 -> [w2429 _]
                      tunnel: [w2428 w2445] -> w2421
                      tunnel: w2411 -> [_ w2448]
                      tunnel: w2420 -> [_ w2435]
                      frame False {
                        n1277 = local read "New: Temp"() -> (w2426:dbl)
                        n1278 = Divide(x=w2429, y=3) -> (x/y=w2431:dbl)
                        n1279 = Format Value(format string="%#g", value (0)=w2426) -> (output string=w2425:string)  [unwired: 1 in]
                        n1280 = To Word Integer(number=w2431) -> (16bit integer=w2430:i16)
                        n1281 = Replace Array Subset(array=w2432, new element=w2425, index (row)=w2430, index (col)=1) -> (w2428:string[][])
                      }
                      frame True {
                        n1282 = local read "New: Temp"() -> (w2437:dbl)
                        n1283 = Search 1D Array(1D array=w2448, element="Width (um):") -> (index of element=w2442:i32)  [unwired: 1 in]
                        n1284 = Divide(x=w2442, y=3) -> (x/y=w2443:dbl)
                        n1285 = To Word Integer(number=w2443) -> (16bit integer=w2441:i16)
                        n1286 = Format Value(format string="%#g", value (0)=w2437) -> (output string=w2436:string)  [unwired: 1 in]
                        n1287 = Build Array(w2435, w2436) -> (w2439:string[])
                        n1288 = Increment(x=w2441) -> (x+1=w2440:i16)
                        n1289 = Insert Into Array(array=w2446, index (row)=w2440, new element=w2439) -> (w2445:string[][])  [unwired: 1 in]
                      }
                    }
                    n1290 = local write "Save1 Array"(w2421) -> ()
                  }
                  frame #4 {
                    w2458 = "Mobility-Sat (cm^2/Vs):"
                    n1291 = local read "Save1 Array"() -> (w2450:string[][])
                    n1292 = Array Size(array=w2450) -> (size(s)=w2455:i32[])
                    n1293 = Array Subset(array=w2450, index (row)=0, index (col)=0, length (col)=3) -> (w2451:string[][])  [unwired: 1 in]
                    n1294 = Index Array(array=w2455, index=0) -> (element=w2457:i32)
                    n1295 = Reshape Array(w2451, w2457) -> (w2449:string[])
                    n1296 = Search 1D Array(1D array=w2449, element=w2458) -> (index of element=w2461:i32)  [unwired: 1 in]
                    n1297 = Equal?(x=w2461, y=-1) -> (x = y?=w2460:bool)
                    n1298 = case shown="True" w2460 {
                      tunnel: w2450 -> [w2470 w2478]
                      tunnel: w2461 -> [w2467 _]
                      tunnel: [w2466 w2477] -> w2459
                      tunnel: w2449 -> [_ w2475]
                      tunnel: w2458 -> [_ w2473]
                      frame False {
                        n1299 = local read "New: Mobility-Sat"() -> (w2463:dbl)
                        n1300 = Divide(x=w2467, y=3) -> (x/y=w2469:dbl)
                        n1301 = To Word Integer(number=w2469) -> (16bit integer=w2468:i16)
                        n1302 = Format Value(format string="%#g", value (0)=w2463) -> (output string=w2464:string)  [unwired: 1 in]
                        n1303 = Replace Array Subset(array=w2470, new element=w2464, index (row)=w2468, index (col)=1) -> (w2466:string[][])
                      }
                      frame True {
                        n1304 = local read "New: Mobility-Sat"() -> (w2479:dbl)
                        n1305 = Search 1D Array(1D array=w2475, element="Mobility (cm^2/Vs):") -> (index of element=w2482:i32)  [unwired: 1 in]
                        n1306 = Divide(x=w2482, y=3) -> (x/y=w2483:dbl)
                        n1307 = To Word Integer(number=w2483) -> (16bit integer=w2474:i16)
                        n1308 = Format Value(format string="%#g", value (0)=w2479) -> (output string=w2476:string)  [unwired: 1 in]
                        n1309 = Build Array(w2473, w2476) -> (w2481:string[])
                        n1310 = Replace Array Subset(array=w2478, new element=w2481, index (row)=w2474) -> (w2477:string[][])  [unwired: 1 in]
                      }
                    }
                    n1311 = local write "Save1 Array"(w2459) -> ()
                  }
                  frame #5 {
                    w2495 = "Mobility-Lin (cm^2/Vs):"
                    n1312 = local read "Save1 Array"() -> (w2486:string[][])
                    n1313 = Array Size(array=w2486) -> (size(s)=w2492:i32[])
                    n1314 = Array Subset(array=w2486, index (row)=0, index (col)=0, length (col)=3) -> (w2488:string[][])  [unwired: 1 in]
                    n1315 = Index Array(array=w2492, index=0) -> (element=w2494:i32)
                    n1316 = Reshape Array(w2488, w2494) -> (w2487:string[])
                    n1317 = Search 1D Array(1D array=w2487, element=w2495) -> (index of element=w2498:i32)  [unwired: 1 in]
                    n1318 = Equal?(x=w2498, y=-1) -> (x = y?=w2497:bool)
                    n1319 = case shown="True" w2497 {
                      tunnel: w2486 -> [w2507 w2513]
                      tunnel: w2498 -> [w2504 _]
                      tunnel: [w2503 w2512] -> w2496
                      tunnel: w2487 -> [_ w2511]
                      tunnel: w2495 -> [_ w2510]
                      frame False {
                        n1320 = local read "Calc: Mobility-Lin"() -> (w2500:dbl)
                        n1321 = Divide(x=w2504, y=3) -> (x/y=w2506:dbl)
                        n1322 = To Word Integer(number=w2506) -> (16bit integer=w2505:i16)
                        n1323 = Format Value(format string="%#g", value (0)=w2500) -> (output string=w2501:string)  [unwired: 1 in]
                        n1324 = Replace Array Subset(array=w2507, new element=w2501, index (row)=w2505, index (col)=1) -> (w2503:string[][])
                      }
                      frame True {
                        n1325 = local read "Calc: Mobility-Lin"() -> (w2514:dbl)
                        n1326 = Search 1D Array(1D array=w2511, element="Mobility-Sat (cm^2/Vs):") -> (index of element=w2519:i32)  [unwired: 1 in]
                        n1327 = Divide(x=w2519, y=3) -> (x/y=w2520:dbl)
                        n1328 = To Word Integer(number=w2520) -> (16bit integer=w2518:i16)
                        n1329 = Format Value(format string="%#g", value (0)=w2514) -> (output string=w2523:string)  [unwired: 1 in]
                        n1330 = Build Array(w2510, w2523) -> (w2516:string[])
                        n1331 = Increment(x=w2518) -> (x+1=w2517:i16)
                        n1332 = Insert Into Array(array=w2513, index (row)=w2517, new element=w2516) -> (w2512:string[][])  [unwired: 1 in]
                      }
                    }
                    n1333 = local write "Save1 Array"(w2496) -> ()
                  }
                  frame #6 {
                    w2533 = "On/Off I-Sat:"
                    n1334 = local read "Save1 Array"() -> (w2524:string[][])
                    n1335 = Array Size(array=w2524) -> (size(s)=w2530:i32[])
                    n1336 = Array Subset(array=w2524, index (row)=0, index (col)=0, length (col)=3) -> (w2526:string[][])  [unwired: 1 in]
                    n1337 = Index Array(array=w2530, index=0) -> (element=w2532:i32)
                    n1338 = Reshape Array(w2526, w2532) -> (w2525:string[])
                    n1339 = Search 1D Array(1D array=w2525, element=w2533) -> (index of element=w2536:i32)  [unwired: 1 in]
                    n1340 = Equal?(x=w2536, y=-1) -> (x = y?=w2535:bool)
                    n1341 = case shown="True" w2535 {
                      tunnel: w2524 -> [w2545 w2552]
                      tunnel: w2536 -> [w2542 _]
                      tunnel: [w2541 w2553] -> w2534
                      tunnel: w2525 -> [_ w2550]
                      tunnel: w2533 -> [_ w2548]
                      frame False {
                        n1342 = local read "Calc: On/Off"() -> (w2538:dbl)
                        n1343 = Divide(x=w2542, y=3) -> (x/y=w2544:dbl)
                        n1344 = To Word Integer(number=w2544) -> (16bit integer=w2543:i16)
                        n1345 = Format Value(format string="%#g", value (0)=w2538) -> (output string=w2539:string)  [unwired: 1 in]
                        n1346 = Replace Array Subset(array=w2545, new element=w2539, index (row)=w2543, index (col)=1) -> (w2541:string[][])
                      }
                      frame True {
                        n1347 = local read "Calc: On/Off"() -> (w2554:dbl)
                        n1348 = Search 1D Array(1D array=w2550, element="On/Off Current:") -> (index of element=w2557:i32)  [unwired: 1 in]
                        n1349 = Divide(x=w2557, y=3) -> (x/y=w2558:dbl)
                        n1350 = To Word Integer(number=w2558) -> (16bit integer=w2549:i16)
                        n1351 = Format Value(format string="%#g", value (0)=w2554) -> (output string=w2551:string)  [unwired: 1 in]
                        n1352 = Build Array(w2548, w2551) -> (w2556:string[])
                        n1353 = Replace Array Subset(array=w2552, new element=w2556, index (row)=w2549) -> (w2553:string[][])  [unwired: 1 in]
                      }
                    }
                    n1354 = local write "Save1 Array"(w2534) -> ()
                  }
                  frame #7 {
                    w2570 = "Off I-Sat (A):"
                    n1355 = local read "Save1 Array"() -> (w2561:string[][])
                    n1356 = Array Size(array=w2561) -> (size(s)=w2567:i32[])
                    n1357 = Array Subset(array=w2561, index (row)=0, index (col)=0, length (col)=3) -> (w2563:string[][])  [unwired: 1 in]
                    n1358 = Index Array(array=w2567, index=0) -> (element=w2569:i32)
                    n1359 = Reshape Array(w2563, w2569) -> (w2562:string[])
                    n1360 = Search 1D Array(1D array=w2562, element=w2570) -> (index of element=w2573:i32)  [unwired: 1 in]
                    n1361 = Equal?(x=w2573, y=-1) -> (x = y?=w2572:bool)
                    n1362 = case shown="True" w2572 {
                      tunnel: w2561 -> [w2582 w2588]
                      tunnel: w2573 -> [w2579 _]
                      tunnel: [w2578 w2587] -> w2571
                      tunnel: w2562 -> [_ w2586]
                      tunnel: w2570 -> [_ w2585]
                      frame False {
                        n1363 = local read "Calc: Off I-Sat"() -> (w2577:dbl)
                        n1364 = Divide(x=w2579, y=3) -> (x/y=w2581:dbl)
                        n1365 = Format Value(format string="%#g", value (0)=w2577) -> (output string=w2575:string)  [unwired: 1 in]
                        n1366 = To Word Integer(number=w2581) -> (16bit integer=w2580:i16)
                        n1367 = Replace Array Subset(array=w2582, new element=w2575, index (row)=w2580, index (col)=1) -> (w2578:string[][])
                      }
                      frame True {
                        n1368 = local read "Calc: Off I-Sat"() -> (w2589:dbl)
                        n1369 = Search 1D Array(1D array=w2586, element="On/Off I-Sat:") -> (index of element=w2594:i32)  [unwired: 1 in]
                        n1370 = Divide(x=w2594, y=3) -> (x/y=w2595:dbl)
                        n1371 = To Word Integer(number=w2595) -> (16bit integer=w2593:i16)
                        n1372 = Format Value(format string="%#g", value (0)=w2589) -> (output string=w2598:string)  [unwired: 1 in]
                        n1373 = Build Array(w2585, w2598) -> (w2591:string[])
                        n1374 = Increment(x=w2593) -> (x+1=w2592:i16)
                        n1375 = Insert Into Array(array=w2588, index (row)=w2592, new element=w2591) -> (w2587:string[][])  [unwired: 1 in]
                      }
                    }
                    n1376 = local write "Save1 Array"(w2571) -> ()
                  }
                  frame #8 {
                    w2600 = "Vt-Sat (V):"
                    n1377 = local read "Save1 Array"() -> (w2601:string[][])
                    n1378 = Array Size(array=w2601) -> (size(s)=w2606:i32[])
                    n1379 = Array Subset(array=w2601, index (row)=0, index (col)=0, length (col)=3) -> (w2602:string[][])  [unwired: 1 in]
                    n1380 = Index Array(array=w2606, index=0) -> (element=w2608:i32)
                    n1381 = Reshape Array(w2602, w2608) -> (w2599:string[])
                    n1382 = Search 1D Array(1D array=w2599, element=w2600) -> (index of element=w2611:i32)  [unwired: 1 in]
                    n1383 = Equal?(x=w2611, y=-1) -> (x = y?=w2610:bool)
                    n1384 = case shown="True" w2610 {
                      tunnel: w2601 -> [w2618 w2627]
                      tunnel: w2611 -> [w2614 _]
                      tunnel: [w2613 w2626] -> w2609
                      tunnel: w2600 -> [_ w2625]
                      tunnel: w2599 -> [_ w2624]
                      frame False {
                        n1385 = local read "New: VT-Sat"() -> (w2620:dbl)
                        n1386 = Number To Fractional String(number=w2620) -> (F-format string=w2615:string)  [unwired: 3 in]
                        n1387 = Divide(x=w2614, y=3) -> (x/y=w2617:dbl)
                        n1388 = To Word Integer(number=w2617) -> (16bit integer=w2616:i16)
                        n1389 = Replace Array Subset(array=w2618, new element=w2615, index (row)=w2616, index (col)=1) -> (w2613:string[][])
                      }
                      frame True {
                        n1390 = local read "New: VT-Sat"() -> (w2628:dbl)
                        n1391 = Search 1D Array(1D array=w2624, element="Threshold V (V):") -> (index of element=w2623:i32)  [unwired: 1 in]
                        n1392 = Divide(x=w2623, y=3) -> (x/y=w2631:dbl)
                        n1393 = To Word Integer(number=w2631) -> (16bit integer=w2622:i16)
                        n1394 = Format Value(format string="%#g", value (0)=w2628) -> (output string=w2634:string)  [unwired: 1 in]
                        n1395 = Build Array(w2625, w2634) -> (w2630:string[])
                        n1396 = Replace Array Subset(array=w2627, new element=w2630, index (row)=w2622) -> (w2626:string[][])  [unwired: 1 in]
                      }
                    }
                    n1397 = local write "Save1 Array"(w2609) -> ()
                  }
                  frame #9 {
                    n1398 = local read "Save1 Array"() -> (w2635:string[][])
                    n1399 = Array Size(array=w2635) -> (size(s)=w2641:i32[])
                    n1400 = Array Subset(array=w2635, index (row)=0, index (col)=0, length (col)=3) -> (w2637:string[][])  [unwired: 1 in]
                    n1401 = Index Array(array=w2641, index=0) -> (element=w2643:i32)
                    n1402 = Reshape Array(w2637, w2643) -> (w2636:string[])
                    n1403 = Search 1D Array(1D array=w2636, element="VT-Lin (V):") -> (index of element=w2646:i32)  [unwired: 1 in]
                    n1404 = Equal?(x=w2646, y=-1) -> (x = y?=w2645:bool)
                    n1405 = case shown="False" w2645 {
                      tunnel: w2635 -> [w2656 w2659]
                      tunnel: w2646 -> [w2653 _]
                      tunnel: [w2652 w2659] -> w2644
                      frame False {
                        n1406 = local read "New: VT-Lin"() -> (w2650:dbl)
                        n1407 = Divide(x=w2653, y=3) -> (x/y=w2655:dbl)
                        n1408 = Format Value(format string="%#g", value (0)=w2650) -> (output string=w2649:string)  [unwired: 1 in]
                        n1409 = To Word Integer(number=w2655) -> (16bit integer=w2654:i16)
                        n1410 = Replace Array Subset(array=w2656, new element=w2649, index (row)=w2654, index (col)=1) -> (w2652:string[][])
                      }
                      frame True {
                      }
                    }
                    n1411 = local write "Save1 Array"(w2644) -> ()
                  }
                  frame #10 {
                    w2660 = "STS-Sat (V/decade):"
                    n1412 = local read "Save1 Array"() -> (w2662:string[][])
                    n1413 = Array Size(array=w2662) -> (size(s)=w2667:i32[])
                    n1414 = Array Subset(array=w2662, index (row)=0, index (col)=0, length (col)=3) -> (w2663:string[][])  [unwired: 1 in]
                    n1415 = Index Array(array=w2667, index=0) -> (element=w2669:i32)
                    n1416 = Reshape Array(w2663, w2669) -> (w2661:string[])
                    n1417 = Search 1D Array(1D array=w2661, element=w2660) -> (index of element=w2672:i32)  [unwired: 1 in]
                    n1418 = Equal?(x=w2672, y=-1) -> (x = y?=w2671:bool)
                    n1419 = case shown="True" w2671 {
                      tunnel: w2662 -> [w2681 w2687]
                      tunnel: w2672 -> [w2678 _]
                      tunnel: [w2677 w2688] -> w2670
                      tunnel: w2661 -> [_ w2686]
                      tunnel: w2660 -> [_ w2685]
                      frame False {
                        n1420 = local read "New: STS"() -> (w2675:dbl)
                        n1421 = Divide(x=w2678, y=3) -> (x/y=w2680:dbl)
                        n1422 = Format Value(format string="%#g", value (0)=w2675) -> (output string=w2674:string)  [unwired: 1 in]
                        n1423 = To Word Integer(number=w2680) -> (16bit integer=w2679:i16)
                        n1424 = Replace Array Subset(array=w2681, new element=w2674, index (row)=w2679, index (col)=1) -> (w2677:string[][])
                      }
                      frame True {
                        n1425 = local read "New: STS"() -> (w2689:dbl)
                        n1426 = Search 1D Array(1D array=w2686, element="S.T.S. (V/decade):") -> (index of element=w2692:i32)  [unwired: 1 in]
                        n1427 = Divide(x=w2692, y=3) -> (x/y=w2693:dbl)
                        n1428 = To Word Integer(number=w2693) -> (16bit integer=w2684:i16)
                        n1429 = Format Value(format string="%#g", value (0)=w2689) -> (output string=w2696:string)  [unwired: 1 in]
                        n1430 = Build Array(w2685, w2696) -> (w2691:string[])
                        n1431 = Replace Array Subset(array=w2687, new element=w2691, index (row)=w2684) -> (w2688:string[][])  [unwired: 1 in]
                      }
                    }
                    n1432 = local write "Save1 Array"(w2670) -> ()
                  }
                  frame #11 {
                    w2697 = "Trap Density-VT (Traps/Vcm^2):"
                    n1433 = local read "Save1 Array"() -> (w2699:string[][])
                    n1434 = Array Size(array=w2699) -> (size(s)=w2704:i32[])
                    n1435 = Array Subset(array=w2699, index (row)=0, index (col)=0, length (col)=3) -> (w2700:string[][])  [unwired: 1 in]
                    n1436 = Index Array(array=w2704, index=0) -> (element=w2706:i32)
                    n1437 = Reshape Array(w2700, w2706) -> (w2698:string[])
                    n1438 = Search 1D Array(1D array=w2698, element=w2697) -> (index of element=w2709:i32)  [unwired: 1 in]
                    n1439 = Equal?(x=w2709, y=-1) -> (x = y?=w2708:bool)
                    n1440 = case shown="True" w2708 {
                      tunnel: w2699 -> [w2718 w2723]
                      tunnel: w2709 -> [w2714 _]
                      tunnel: [w2713 w2724] -> w2707
                      tunnel: w2698 -> [_ w2722]
                      tunnel: w2697 -> [_ w2721]
                      frame False {
                        n1441 = local read "New: Trap Density-VT"() -> (w2712:dbl)
                        n1442 = Format Value(format string="%#g", value (0)=w2712) -> (output string=w2715:string)  [unwired: 1 in]
                        n1443 = Divide(x=w2714, y=3) -> (x/y=w2717:dbl)
                        n1444 = To Word Integer(number=w2717) -> (16bit integer=w2716:i16)
                        n1445 = Replace Array Subset(array=w2718, new element=w2715, index (row)=w2716, index (col)=1) -> (w2713:string[][])
                      }
                      frame True {
                        n1446 = local read "New: Trap Density-VT"() -> (w2734:dbl)
                        n1447 = Search 1D Array(1D array=w2722, element="STS-Sat (V/decade):") -> (index of element=w2729:i32)  [unwired: 1 in]
                        n1448 = Divide(x=w2729, y=3) -> (x/y=w2728:dbl)
                        n1449 = To Word Integer(number=w2728) -> (16bit integer=w2730:i16)
                        n1450 = Format Value(format string="%#g", value (0)=w2734) -> (output string=w2725:string)  [unwired: 1 in]
                        n1451 = Build Array(w2721, w2725) -> (w2732:string[])
                        n1452 = Increment(x=w2730) -> (x+1=w2731:i16)
                        n1453 = Insert Into Array(array=w2723, index (row)=w2731, new element=w2732) -> (w2724:string[][])  [unwired: 1 in]
                      }
                    }
                    n1454 = local write "Save1 Array"(w2707) -> ()
                  }
                  frame #12 {
                    w2736 = "Trap Density-STS (Traps/Vcm^2):"
                    n1455 = local read "Save1 Array"() -> (w2738:string[][])
                    n1456 = Array Size(array=w2738) -> (size(s)=w2743:i32[])
                    n1457 = Array Subset(array=w2738, index (row)=0, index (col)=0, length (col)=3) -> (w2739:string[][])  [unwired: 1 in]
                    n1458 = Index Array(array=w2743, index=0) -> (element=w2745:i32)
                    n1459 = Reshape Array(w2739, w2745) -> (w2737:string[])
                    n1460 = Search 1D Array(1D array=w2737, element=w2736) -> (index of element=w2747:i32)  [unwired: 1 in]
                    n1461 = Equal?(x=w2747, y=-1) -> (x = y?=w2746:bool)
                    n1462 = case shown="True" w2746 {
                      tunnel: w2738 -> [w2756 w2761]
                      tunnel: w2747 -> [w2753 _]
                      tunnel: [w2752 w2762] -> w2735
                      tunnel: w2737 -> [_ w2760]
                      tunnel: w2736 -> [_ w2759]
                      frame False {
                        n1463 = local read "New: Trap Density-STS"() -> (w2750:dbl)
                        n1464 = Divide(x=w2753, y=3) -> (x/y=w2755:dbl)
                        n1465 = To Word Integer(number=w2755) -> (16bit integer=w2754:i16)
                        n1466 = Format Value(format string="%#g", value (0)=w2750) -> (output string=w2749:string)  [unwired: 1 in]
                        n1467 = Replace Array Subset(array=w2756, new element=w2749, index (row)=w2754, index (col)=1) -> (w2752:string[][])
                      }
                      frame True {
                        n1468 = local read "New: Trap Density-STS"() -> (w2763:dbl)
                        n1469 = Search 1D Array(1D array=w2760, element="Trap Density-VT (Traps/Vcm^2):") -> (index of element=w2768:i32)  [unwired: 1 in]
                        n1470 = Divide(x=w2768, y=3) -> (x/y=w2769:dbl)
                        n1471 = To Word Integer(number=w2769) -> (16bit integer=w2767:i16)
                        n1472 = Format Value(format string="%#g", value (0)=w2763) -> (output string=w2772:string)  [unwired: 1 in]
                        n1473 = Build Array(w2759, w2772) -> (w2765:string[])
                        n1474 = Increment(x=w2767) -> (x+1=w2766:i16)
                        n1475 = Insert Into Array(array=w2761, index (row)=w2766, new element=w2765) -> (w2762:string[][])  [unwired: 1 in]
                      }
                    }
                    n1476 = local write "Save1 Array"(w2735) -> ()
                  }
                }
                n1477 = String To Path(string=w2332) -> (path=w2315:path)
                "No Image 2" <- w2315
              }
              frame #1 {
                n1478 = Equal?(x=w2776, y=w2775) -> (x = y?=w2774:bool)
                n1479 = case shown="False" w2774 {
                  tunnel: w2776 -> [w2780 _]
                  tunnel: w2775 -> [w2779 _]
                  frame False {
                    n1480 = Move(source path=w2780, 9:TRUE, 10:w2779) -> ()  [unwired: 2 in, 3 out]
                  }
                  frame True {
                  }
                }
              }
              frame #2 {
                n1481 = local write "Transfer File"(w2782) -> ()
                n1482 = call-poly <vilib>:"Write To Spreadsheet File.vi"("2D data"=w2781, "file path (dialog if empty)"=w2782) -> ()  [unwired: 6 in, 1 out]
              }
              frame #3 {
                w2882 = 0
                # "Moves to next file and displays new image/data"
                n1483 = property on="Image Out" class="ImageControl"() -> (error out=w2844:errorcluster, "Image Center Position"=w2848:cluster{"X":u32, "Y":u32})  [unwired: 2 in, 1 out]
                n1484 = local read "Transfer File"() -> (w2887:path)
                n1485 = Strip Path(path=w2887) -> (stripped path=w2878:path, name=w2896:string)
                n1486 = Unbundle(w2848) -> ("X"=w2846:u32)  [unwired: 1 out]
                n1487 = local write "Transfer Folder"(w2878) -> ()
                n1488 = Bundle("X"=w2846, 0) -> (w2847:cluster{"X":u32, i32})  [unwired: 1 in]
                n1489 = property on="Image Out" class="ImageControl"(error in=w2844, "Image Center Position"=w2847) -> ()  [unwired: 1 in, 2 out]
                n1490 = List Folder(path=w2878) -> (filenames=w2892:string[])  [unwired: 3 in, 3 out]
                n1491 = Search 1D Array(1D array=w2892, element=w2896) -> (index of element=w2889:i32)  [unwired: 1 in]
                n1492 = Array Size(array=w2892) -> (size(s)=w2888:i32)
                n1493 = Decrement(x=w2888) -> (x-1=w2890:i32)
                n1494 = Equal?(x=w2889, y=w2890) -> (x = y?=w2891:bool)
                n1495 = local read "Folder Index"() -> (w2840:dbl)
                n1496 = case shown="False" w2891 {
                  tunnel: w2840 -> [w3021 _]
                  tunnel: [w3020 0] -> w2839
                  frame False {
                    n1497 = Increment(x=w3021) -> (x+1=w3020:dbl)
                  }
                  frame True {
                  }
                }
                n1498 = invoke on="Image Out" class="ImageControl" method="Clear ROI"() -> ()  [unwired: 3 in, 3 out]
                n1499 = local write "Folder Index"(w2839) -> ()
                n1500 = Path To String(path=w2878) -> (string=w2897:string)
                n1501 = Index Array(array=w2892, index=w2839) -> (element=w2893:string)
                n1502 = local write "Data Name:"(w2893) -> ()
                n1503 = Concatenate Strings(w2897, "\\", w2893) -> (w2895:string)
                n1504 = String To Path(string=w2895) -> (path=w2791:path)
                n1505 = call "Recorded Values.vi"("Path"=w2791) -> ("Recorded Char"=w2793:T5, "Recorded Prop"=w2794:T6, "Fabrication Prop"=w2792:T7)  [unwired: 8 in]
                n1506 = Unbundle By Name(w2793) -> ("Mobility-Sat"=w2806:dbl, "Moblitity-Lin"=w2807:dbl, "On/Off"=w2808:dbl, "Off Current"=w2809:dbl, "Vt-Sat"=w2785:dbl, "STS"=w2810:dbl, "Trap Density-VT"=w2811:dbl, "Trap Density-STS"=w2812:dbl)
                n1507 = Unbundle By Name(w2794) -> ("Date Recorded"=w2802:string, "Index"=w2803:string, "Length"=w2804:dbl, "Width"=w2805:dbl, "Sample Temp"=w2788:dbl)
                n1508 = Unbundle By Name(w2792) -> ("Date Created"=w2813:string, "Material"=w2795:string, "Solvent"=w2796:string, "Concentration"=w2797:dbl, "Method"=w2798:string, "Dielectric (nm)"=w2799:dbl, "Treatment"=w2800:string, "Comments"=w2801:string)
                n1509 = local write "Rec: Off I-Sat"(w2809) -> ()
                n1510 = local write "Rec: VT-Sat"(w2785) -> ()
                n1511 = local write "Date Created"(w2813) -> ()
                n1512 = local write "Rec: Material"(w2795) -> ()
                n1513 = local write "Rec: Solvent"(w2796) -> ()
                n1514 = local write "Rec: Concentration"(w2797) -> ()
                n1515 = local write "Rec: Method"(w2798) -> ()
                n1516 = local write "Rec: Dielectric (d)"(w2799) -> ()
                n1517 = local write "Surface Treatment:"(w2800) -> ()
                n1518 = local write "Comments"(w2801) -> ()
                n1519 = local write "Index"(w2803) -> ()
                n1520 = local write "Rec: Mobility-Sat"(w2806) -> ()
                n1521 = local write "Rec: Mobility-Lin"(w2807) -> ()
                n1522 = local write "Rec: On/Off"(w2808) -> ()
                n1523 = local write "Rec: STS"(w2810) -> ()
                n1524 = local write "Rec: Trap Density-VT"(w2811) -> ()
                n1525 = local write "Rec: Trap Density-STS"(w2812) -> ()
                n1526 = local write "Date Recorded"(w2802) -> ()
                n1527 = local write "Rec: Length"(w2804) -> ()
                n1528 = local write "Rec: Width"(w2805) -> ()
                n1529 = local write "Rec: Temp"(w2788) -> ()
                n1530 = Equal To 0?(x=w2788) -> (x = 0?=w2789:bool)
                n1531 = case shown="False" w2789 {
                  tunnel: [w2898 w2899] -> w2786
                  tunnel: w2788 -> [w2898 _]
                  frame False {
                  }
                  frame True {
                    n1532 = local read "Room Temp"() -> (w2899:dbl)
                  }
                }
                n1533 = local write "Transfer File"(w2791) -> ()
                n1534 = local read "NumPts 2"() -> (w2835:dbl)
                n1535 = local read "NumPts"() -> (w2824:dbl)
                n1536 = local read "NumPts"() -> (w2836:dbl)
                n1537 = call-poly <vilib>:"Read From Spreadsheet File.vi"("file path (dialog if empty)"=w2791) -> ("all rows"=w2884:string[][])  [unwired: 6 in, 4 out]
                n1538 = call "Mobility-Vt Calculator-File.vi"("NumPts"=w2836, "Path"=w2791) -> ("XY Graph-Sat"=w2837:cluster{dbl[], dbl[]}[], "XY Graph-Lin"=w2819:cluster{dbl[], dbl[]}[], "Output"=w2838:T8, "Index-Sat"=w2816:dbl, "Index-Lin"=w2823:dbl)  [unwired: 4 in, 1 out]
                n1539 = Decimate 1D Array(w2819) -> (w2831:cluster{dbl[], dbl[]}[])  [unwired: 1 out]
                n1540 = Array To Cluster(array=w2831) -> (cluster=w2829:T9)
                n1541 = Unbundle(w2829) -> ("[0]"=w2830:cluster{dbl[], dbl[]})  [unwired: 8 out]
                n1542 = local write "XY Graph-Lin"(w2819) -> ()
                n1543 = Unbundle(w2830) -> (w2828:dbl[], w2827:dbl[])
                n1544 = Array Subset(array=w2827, index=w2823, length=w2824) -> (w2825:dbl[])
                n1545 = Array Subset(array=w2828, index=w2823, length=w2824) -> (w2826:dbl[])
                n1546 = call "STS Calculator-File.vi"("NumPts"=w2835, "Path"=w2791) -> ("STS Index-Sat"=w2834:dbl, "XY Graph-Sat"=w2833:cluster{dbl[], dbl[]}[], "Ouput"=w2832:cluster{"STS-Sat":dbl, "STS-Lin":dbl})  [unwired: 5 in, 2 out]
                n1547 = local read "New: Dielectric"() -> (w2818:dbl)
                n1548 = local write "Lin Id-Used"(w2825) -> ()
                n1549 = local write "Lin-Vg Array-Used"(w2826) -> ()
                n1550 = local write "MobVi Index"(w2816) -> ()
                n1551 = local write "Slide"(w2816) -> ()
                n1552 = local write "XY Graph"(w2837) -> ()
                n1553 = local write "Index 2"(w2834) -> ()
                n1554 = local write "XY Graph 2"(w2833) -> ()
                n1555 = Unbundle By Name(w2838) -> ("Mobility-Sat"=w2822:dbl, "Vt-Sat"=w2783:dbl, "Mobility-Lin"=w2821:dbl, "Mobility-Lin"=w2820:dbl, "Off I-Sat"=w2814:dbl, "On/Off I-Sat"=w2784:dbl)
                n1556 = Array Size(array=w2884) -> (size(s)=w2883:i32[])
                n1557 = local write "New: Temp"(w2786) -> ()
                n1558 = Unbundle By Name(w2832) -> ("STS-Sat"=w2817:dbl)
                n1559 = call "Trap Density_STS.vi"("Temp (T) [K]"=w2786, "S.T.S. (S)"=w2817, "Dielectric"=w2818) -> ("Trap Density (N)"=w2790:dbl)  [unwired: 8 in]
                n1560 = local write "Calc: Mobility-Lin"(w2821) -> ()
                n1561 = local write "Calc: Mobility-Sat"(w2822) -> ()
                n1562 = local write "Calc: Off I-Sat"(w2814) -> ()
                n1563 = local write "Calc: VT-Sat"(w2783) -> ()
                n1564 = local write "New: VT-Lin"(w2820) -> ()
                n1565 = local write "New: Trap Density-STS"(w2790) -> ()
                n1566 = local write "Calc: Trap Density-STS"(w2790) -> ()
                n1567 = local read "Image Folder"() -> (w2872:path)
                n1568 = local read "New: Dielectric"() -> (w2815:dbl)
                n1569 = Decimate 1D Array(w2837) -> (w2867:cluster{dbl[], dbl[]}[])  [unwired: 1 out]
                n1570 = Decimate 1D Array(w2833) -> (w2857:cluster{dbl[], dbl[]}[])  [unwired: 1 out]
                n1571 = Index Array(array=w2883, index=w2882) -> (element=w2863:i32)
                n1572 = Array Subset(array=w2884, index (row)=w2882, index (col)=w2882, length (col)=3) -> (w2885:string[][])  [unwired: 1 in]
                n1573 = local write "Calc: STS"(w2817) -> ()
                n1574 = local write "New: VT-Sat"(w2783) -> ()
                n1575 = local write "New: Mobility-Sat"(w2822) -> ()
                n1576 = local write "Calc: On/Off"(w2784) -> ()
                n1577 = local write "New: Mobility-Lin"(w2821) -> ()
                n1578 = List Folder(path=w2872) -> (filenames=w2877:string[])  [unwired: 3 in, 3 out]
                n1579 = local write "New: VT-Lin"(w2820) -> ()
                n1580 = Array To Cluster(array=w2867) -> (cluster=w2869:T9)
                n1581 = Array To Cluster(array=w2857) -> (cluster=w2855:T9)
                n1582 = Reshape Array(w2885, w2863) -> (w2870:string[])
                n1583 = Subtract(x=w2863, y=20) -> (x-y=w2862:i32)
                n1584 = local write "New: STS"(w2817) -> ()
                n1585 = property on="Slide" class="Slide (strict)"("Scale.Maximum"=w2862) -> ()  [unwired: 2 in, 2 out]
                n1586 = call "Trap Density_VT.vi"("VT"=w2783, "Dielectric"=w2815) -> ("Trap Density-VT"=w2787:dbl)
                n1587 = Unbundle(w2869) -> ("[0]"=w2868:cluster{dbl[], dbl[]})  [unwired: 8 out]
                n1588 = Unbundle(w2855) -> ("[0]"=w2856:cluster{dbl[], dbl[]})  [unwired: 8 out]
                n1589 = Search 1D Array(1D array=w2870, element="Index:") -> (index of element=w2879:i32)  [unwired: 1 in]
                n1590 = local write "New: Trap Density-VT"(w2787) -> ()
                n1591 = local write "Calc: Trap Density-VT"(w2787) -> ()
                n1592 = Unbundle(w2868) -> (w2859:dbl[], w2858:dbl[])
                n1593 = Unbundle(w2856) -> (w2854:dbl[], w2853:dbl[])
                n1594 = Increment(x=w2879) -> (x+1=w2880:i32)
                n1595 = Array Subset(array=w2859, index=w2816, length=w2836) -> (w2866:dbl[])
                n1596 = Array Subset(array=w2858, index=w2816, length=w2836) -> (w2865:dbl[])
                n1597 = Array Subset(array=w2854, index=w2834, length=w2835) -> (w2861:dbl[])
                n1598 = Array Subset(array=w2853, index=w2834, length=w2835) -> (w2860:dbl[])
                n1599 = Index Array(array=w2870, index=w2880) -> (element=w2875:string)
                n1600 = local write "Vg Array-Log-Used"(w2860) -> ()
                n1601 = local write "Sat Id-Log-Used"(w2861) -> ()
                n1602 = local write "Sat Id-Used"(w2865) -> ()
                n1603 = local write "Index"(w2875) -> ()
                n1604 = local write "Sat Vg Array-Used"(w2866) -> ()
                n1605 = while {
                  tunnel: w2877 -> [w2907]
                  tunnel: w2875 -> [w2905]
                  tunnel: [w2904] -> _
                  tunnel: [w2904] -> w2876
                  tunnel: w2863 -> [w2903]
                  i -> [w2904]
                  stop <- w2900 stop-if-true
                  n1606 = Index Array(array=w2907, index=w2904) -> (element=w2908:string)
                  n1607 = xnode "Match Regular Expression"("input string"=w2908, "regular expression"=w2905) -> ("whole match"=w2906:string)  [unwired: 4 in, 4 out]
                  n1608 = Equal?(x=w2906, y=w2905) -> (x = y?=w2902:bool)
                  n1609 = Equal?(x=w2903, y=w2904) -> (x = y?=w2901:bool)
                  n1610 = Or(x=w2902, y=w2901) -> (x .or. y?=w2900:bool)
                }
                n1611 = Path To String(path=w2872) -> (string=w2874:string)
                n1612 = Index Array(array=w2877, index=w2876) -> (element=w2851:string)
                n1613 = local write "Image Name"(w2851) -> ()
                n1614 = Empty String/Path?(string/path=w2851) -> (empty?=w2852:bool)
                n1615 = Concatenate Strings(w2874, "\\", w2851) -> (w2873:string)
                n1616 = String To Path(string=w2873) -> (path=w2850:path)
                n1617 = local read "No Image File"() -> (w2849:path)
                n1618 = Select(t=w2849, s=w2852, f=w2850) -> (s? t:f=w2843:path)
                n1619 = local write "Image File"(w2843) -> ()
                n1620 = local read "Image Out"() -> (w2841:T2)
                n1621 = call "IMAQ ReadFile"("File Path"=w2843, "Image"=w2841) -> ("Image Out"=w2842:T2)  [unwired: 5 in, 4 out]
                n1622 = local write "Image Out"(w2842) -> ()
                n1623 = local write "Image Out 2"(w2842) -> ()
              }
              frame #4 {
                # "Output ROI data"
                n1624 = local read "Image Folder"() -> (w3023:path)
                n1625 = Build Path(base path=w3023, name or relative path="ROI") -> (appended path=w3025:path)
                n1626 = local read "Index"() -> (w3024:string)
                n1627 = Build Path(base path=w3025, name or relative path=w3024) -> (appended path=w3030:path)
                n1628 = invoke on="Image Out" class="ImageControl" method="Clear ROI"() -> (error out=w3029:errorcluster)  [unwired: 3 in, 2 out]
                n1629 = call <vilib>:"Check if File or Folder Exists.vi"("error in (no error)"=w3029, "path"=w3030) -> ("file or folder exists?"=w3027:bool, "dup path"=w3028:path)  [unwired: 7 in, 1 out]
                n1630 = case shown="True" w3027 {
                  tunnel: w3028 -> [_ w3031]
                  frame False {
                  }
                  frame True {
                    n1631 = Read from Text File(file (use dialog)=w3031) -> (text=w3035:string)  [unwired: 3 in, 3 out]
                    n1632 = property on="Image Out" class="ImageControl"() -> ("ROI"=w3032:T10)  [unwired: 2 in, 2 out]
                    n1633 = Unflatten From String(type=w3032, binary string=w3035) -> (value=w3033:T10, error out=w3034:errorcluster)  [unwired: 3 in, 1 out]
                    n1634 = property on="Image Out" class="ImageControl"(error in=w3034, "ROI"=w3033) -> ()  [unwired: 1 in, 2 out]
                  }
                }
              }
            }
            n1635 = flat-sequence {
              tunnel: [w2272] -> w2259
              tunnel: w2259 -> [w2286]
              frame #0 {
                # "Makes Empty File for Transformer Data"
                n1636 = local read "Transfer Folder"() -> (w2261:path)
                n1637 = Build Path(base path=w2261, name or relative path="Stats") -> (appended path=w2263:path)
                n1638 = call <vilib>:"Check if File or Folder Exists.vi"("path"=w2263) -> ("file or folder exists?"=w2264:bool, "dup path"=w2265:path)  [unwired: 8 in, 1 out]
                n1639 = case shown="False" w2264 {
                  tunnel: [w2269 w2271] -> w2266
                  tunnel: w2265 -> [w2270 w2271]
                  frame False {
                    n1640 = Create Folder(path (use dialog)=w2270) -> (created path=w2269:path)  [unwired: 2 in, 2 out]
                  }
                  frame True {
                  }
                }
                n1641 = Build Path(base path=w2266, name or relative path="Tranformer Data.txt") -> (appended path=w2268:path)
                n1642 = call-poly <vilib>:"Write To Spreadsheet File.vi"("append to file? (new file:F)"=TRUE, "file path (dialog if empty)"=w2268) -> ()  [unwired: 6 in, 1 out]
              }
              frame #1 {
                # "Adds Headers if they don't exist"
                n1643 = local read "Transfer Folder"() -> (w2278:path)
                n1644 = Concatenate Strings("Stats\\", "Tranformer Data.txt") -> (w2279:string)
                n1645 = Build Path(base path=w2278, name or relative path=w2279) -> (appended path=w2272:path)
                n1646 = call-poly <vilib>:"Read From Spreadsheet File.vi"("file path (dialog if empty)"=w2272) -> ("first row"=w2277:string[])  [unwired: 6 in, 4 out]
                n1647 = Search 1D Array(1D array=w2277, element="DeviceID") -> (index of element=w2275:i32)  [unwired: 1 in]
                n1648 = Equal?(x=w2275, y=0) -> (x = y?=w2273:bool)
                n1649 = case shown="False" w2273 {
                  tunnel: w2272 -> [w2283 _]
                  frame False {
                    n1650 = local read "Transformer \nHeaders"() -> (w2282:string[])
                    n1651 = call-poly <vilib>:"Write To Spreadsheet File.vi"("1D data"=w2282, "file path (dialog if empty)"=w2283) -> ()  [unwired: 6 in, 1 out]
                  }
                  frame True {
                  }
                }
              }
              frame #2 {
                # "Adds current device if it doesn't exist"
                n1652 = local read "Current \nRecord"() -> (w2289:string[])
                n1653 = Index Array(array=w2289, index=0) -> (element=w2288:string)
                n1654 = local read "Transfer Folder"() -> (w2291:path)
                n1655 = Concatenate Strings("Stats\\", "Tranformer Data.txt") -> (w2292:string)
                n1656 = local write "Current Device ID"(w2288) -> ()
                n1657 = local read "Current Device ID"() -> (w2298:string)
                n1658 = Build Path(base path=w2291, name or relative path=w2292) -> (appended path=w2290:path)
                n1659 = call-poly <vilib>:"Read From Spreadsheet File.vi"("file path (dialog if empty)"=w2290) -> ("all rows"=w2285:string[][])  [unwired: 6 in, 4 out]
                n1660 = Index Array(array=w2285, index (col)=0) -> (element=w2296:string[])  [unwired: 1 in]
                n1661 = Search 1D Array(1D array=w2296, element=w2298) -> (index of element=w2284:i32)  [unwired: 1 in]
                n1662 = Equal?(x=w2284, y=-1) -> (x = y?=w2287:bool)
                n1663 = case shown="False" w2287 {
                  tunnel: w2286 -> [w2300 w2313]
                  tunnel: w2284 -> [w2305 _]
                  tunnel: w2285 -> [w2306 _]
                  frame False {
                    n1664 = local read "Current \nRecord"() -> (w2304:string[])
                    n1665 = Replace Array Subset(array=w2306, new element=w2304, index (row)=w2305) -> (w2301:string[][])  [unwired: 1 in]
                    n1666 = flat-sequence {
                      tunnel: [w2307] -> _
                      tunnel: [w2308] -> _
                      tunnel: [w2308] -> w2303
                      tunnel: [w2307] -> w2302
                      tunnel: w2301 -> [w2308]
                      tunnel: w2300 -> [w2307]
                      tunnel: w2303 -> [w2310]
                      tunnel: w2302 -> [w2309]
                      frame #0 {
                        n1667 = Delete(path (use dialog)=w2307) -> ()  [unwired: 4 in, 3 out]
                      }
                      frame #1 {
                        n1668 = call-poly <vilib>:"Write To Spreadsheet File.vi"("append to file? (new file:F)"=TRUE, "2D data"=w2310, "file path (dialog if empty)"=w2309) -> ()  [unwired: 5 in, 1 out]
                      }
                    }
                  }
                  frame True {
                    n1669 = local read "Current \nRecord"() -> (w2312:string[])
                    n1670 = call-poly <vilib>:"Write To Spreadsheet File.vi"("append to file? (new file:F)"=TRUE, "1D data"=w2312, "file path (dialog if empty)"=w2313) -> ()  [unwired: 5 in, 1 out]
                  }
                }
              }
            }
          }
          event "Export": Mouse Down {
            n1671 = event-data() -> ()  [unwired: 1 in, 7 out]
            n1672 = flat-sequence {
              frame #0 {
                n1673 = stacked-sequence {
                  frame #0 {
                    n1674 = local read "Independant Variable"() -> (w3037:string)
                    n1675 = Equal?(x=w3037, y="Length (um):") -> (x = y?=w3038:bool)
                    n1676 = case shown="True" w3038 {
                      frame False {
                      }
                      frame True {
                        n1677 = local write "Opj X Axis"("2") -> ()
                      }
                    }
                  }
                  frame #1 {
                    n1678 = local read "Independant Variable"() -> (w3041:string)
                    n1679 = Equal?(x=w3041, y="Sample Temp (K):") -> (x = y?=w3042:bool)
                    n1680 = case shown="True" w3042 {
                      frame False {
                      }
                      frame True {
                        n1681 = local write "Opj X Axis"("1") -> ()
                      }
                    }
                  }
                  frame #2 {
                    n1682 = local read "Independant Variable"() -> (w3045:string)
                    n1683 = Equal?(x=w3045, y="Mobility-Sat (cm^2/Vs):") -> (x = y?=w3046:bool)
                    n1684 = case shown="True" w3046 {
                      frame False {
                      }
                      frame True {
                        n1685 = local write "Opj X Axis"("2") -> ()
                      }
                    }
                  }
                  frame #3 {
                    n1686 = local read "Independant Variable"() -> (w3049:string)
                    n1687 = Equal?(x=w3049, y="Mobility-Lin (cm^2/Vs):") -> (x = y?=w3050:bool)
                    n1688 = case shown="True" w3050 {
                      frame False {
                      }
                      frame True {
                        n1689 = local write "Opj X Axis"("2") -> ()
                      }
                    }
                  }
                  frame #4 {
                    n1690 = local read "Independant Variable"() -> (w3053:string)
                    n1691 = Equal?(x=w3053, y="On/Off I-Sat:") -> (x = y?=w3054:bool)
                    n1692 = case shown="True" w3054 {
                      frame False {
                      }
                      frame True {
                        n1693 = local write "Opj X Axis"("2") -> ()
                      }
                    }
                  }
                  frame #5 {
                    n1694 = local read "Independant Variable"() -> (w3057:string)
                    n1695 = Equal?(x=w3057, y="Off I-Sat (A):") -> (x = y?=w3058:bool)
                    n1696 = case shown="True" w3058 {
                      frame False {
                      }
                      frame True {
                        n1697 = local write "Opj X Axis"("2") -> ()
                      }
                    }
                  }
                  frame #6 {
                    n1698 = local read "Independant Variable"() -> (w3061:string)
                    n1699 = Equal?(x=w3061, y="Vt-Sat (V):") -> (x = y?=w3062:bool)
                    n1700 = case shown="True" w3062 {
                      frame False {
                      }
                      frame True {
                        n1701 = local write "Opj X Axis"("1") -> ()
                      }
                    }
                  }
                  frame #7 {
                    n1702 = local read "Independant Variable"() -> (w3065:string)
                    n1703 = Equal?(x=w3065, y="STS-Sat (V/decade):") -> (x = y?=w3066:bool)
                    n1704 = case shown="True" w3066 {
                      frame False {
                      }
                      frame True {
                        n1705 = local write "Opj X Axis"("1") -> ()
                      }
                    }
                  }
                  frame #8 {
                    n1706 = local read "Independant Variable"() -> (w3069:string)
                    n1707 = Equal?(x=w3069, y="Trap Density-VT (Traps/Vcm^2):") -> (x = y?=w3070:bool)
                    n1708 = case shown="True" w3070 {
                      frame False {
                      }
                      frame True {
                        n1709 = local write "Opj X Axis"("2") -> ()
                      }
                    }
                  }
                  frame #9 {
                    n1710 = local read "Independant Variable"() -> (w3073:string)
                    n1711 = Equal?(x=w3073, y="Trap Density-STS (Traps/Vcm^2):") -> (x = y?=w3074:bool)
                    n1712 = case shown="True" w3074 {
                      frame False {
                      }
                      frame True {
                        n1713 = local write "Opj X Axis"("2") -> ()
                      }
                    }
                  }
                }
              }
              frame #1 {
                n1714 = local read "Transfer Folder"() -> (w3081:path)
                n1715 = Build Path(base path=w3081, name or relative path="Stats") -> (appended path=w3082:path)
                n1716 = local read "Origin Project File"() -> (w3093:path)
                n1717 = call <vilib>:"Check if File or Folder Exists.vi"("path"=w3082) -> ("file or folder exists?"=w3097:bool, "dup path"=w3096:path)  [unwired: 8 in, 1 out]
                n1718 = call <userlib>:"OA_ConnectToOrigin.vi"() -> ("error out"=w3094:errorcluster, "Origin.IOApplication"=w3095:refnum<k7>)  [unwired: 8 in]
                n1719 = case shown="False" w3097 {
                  tunnel: w3096 -> [w3254 w3255]
                  tunnel: [w3253 w3255] -> w3080
                  frame False {
                    n1720 = Create Folder(path (use dialog)=w3254) -> (created path=w3253:path)  [unwired: 2 in, 2 out]
                  }
                  frame True {
                  }
                }
                n1721 = call <userlib>:"OA_Load.vi"("error in (no error)"=w3094, "Path"=w3093, "Origin.IOApplication"=w3095) -> ("error out"=w3091:errorcluster, "Origin.IOApplication"=w3092:refnum<k7>)  [unwired: 1 out]
                n1722 = call <userlib>:"OAExecute.vi"("script"="document -m 3;", "Error IO"=w3091, "Origin.IOApplication"=w3092) -> ("Error IO Out"=w3089:errorcluster, "Origin.IOApplication"=w3090:refnum<k7>)  [unwired: 1 in, 1 out]
                n1723 = call "File Dialog"("start path"=w3082) -> ("selected path"=w3084:path)  [unwired: 11 in, 3 out]
                n1724 = local read "Independant Variable"() -> (w3077:string)
                n1725 = stacked-sequence {
                  tunnel: w3081 -> [w3106 w3134 w3144 w3164 w3182 w3201 w3220 w3241]
                  tunnel: w3080 -> [w3107 w3133 w3145 w3163 w3183 w3202 w3221 w3242]
                  tunnel: w3090 -> [w3109 w3131 w3147 w3166 w3185 w3204 w3223 w3244]
                  tunnel: w3089 -> [w3108 w3132 w3146 w3165 w3184 w3203 w3222 w3243]
                  tunnel: [_ _ _ _ _ _ _ w3239] -> w3079
                  tunnel: [_ _ _ _ _ _ _ w3240] -> w3078
                  tunnel: w3077 -> [w3105 w3124 w3143 w3162 w3181 w3200 w3219 w3238]
                  frame #0 {
                    n1726 = local read "Opj X Axis"() -> (w3101:string)
                    n1727 = Concatenate Strings("window -a MOBLGraph;\nlayer.x.type=", w3101, ";", "window -a MOBLTable;\nwindow -s TV;") -> (w3099:string)
                    n1728 = call "Param_Analysis_7_24b_JW.vi"("Independant Variable"=w3105, "error in (no error)"=w3108, "Data Folder"=w3106, "Parameter String"="Mobility-Lin (cm^2/Vs):", "Parameter Name"="Mobility-Lin", "Stats Folder"=w3107) -> ("error out"=w3111:errorcluster, "Output Array"=w3113:string[][], "Variables"=w3104:T16)  [unwired: 2 in, 1 out]
                    n1729 = call "Origin_Export_7_27a_JW.vi"("Input Conditions"=w3104, "Analysis Array"=w3113, "error in (no error)"=w3111, "Parameter Worksheet Name"="[MOBLTable]Mobilities", "Parameter Folder Script"="pe_cd \"Mobility-Lin\";", "Origin.IOApplication"=w3109) -> ("error out"=w3110:errorcluster, "reference out"=w3112:refnum<k7>)  [unwired: 3 in, 1 out]
                    n1730 = call <userlib>:"OAExecute.vi"("script"=w3099, "Error IO"=w3110, "Origin.IOApplication"=w3112) -> ()  [unwired: 1 in, 3 out]
                  }
                  frame #1 {
                    n1731 = local read "Opj X Axis"() -> (w3120:string)
                    n1732 = Concatenate Strings("window -a MOBSGraph;\nlayer.x.type=", w3120, ";", "window -a MOBSTable;\nwindow -s TV;") -> (w3118:string)
                    n1733 = call "Param_Analysis_7_24b_JW.vi"("Independant Variable"=w3124, "error in (no error)"=w3132, "Data Folder"=w3134, "Parameter String"="Mobility-Sat (cm^2/Vs):", "Parameter Name"="Mobility-Sat", "Stats Folder"=w3133) -> ("error out"=w3127:errorcluster, "Output Array"=w3125:string[][], "Variables"=w3123:T16)  [unwired: 2 in, 1 out]
                    n1734 = call "Origin_Export_7_27a_JW.vi"("Input Conditions"=w3123, "Analysis Array"=w3125, "error in (no error)"=w3127, "Parameter Worksheet Name"="[MOBSTable]Mobilities", "Parameter Folder Script"="pe_cd \"Mobility-Sat\";", "Origin.IOApplication"=w3131) -> ("error out"=w3126:errorcluster, "reference out"=w3128:refnum<k7>)  [unwired: 3 in, 1 out]
                    n1735 = call <userlib>:"OAExecute.vi"("script"=w3118, "Error IO"=w3126, "Origin.IOApplication"=w3128) -> ()  [unwired: 1 in, 3 out]
                  }
                  frame #2 {
                    n1736 = local read "Opj X Axis"() -> (w3139:string)
                    n1737 = Concatenate Strings("window -a NSTSGraph;\nlayer.x.type=", w3139, ";", "window -a NSTSTable;\nwindow -s TV;") -> (w3137:string)
                    n1738 = call "Param_Analysis_7_24b_JW.vi"("Independant Variable"=w3143, "error in (no error)"=w3146, "Data Folder"=w3144, "Parameter String"="Trap Density-STS (Traps/Vcm^2):", "Parameter Name"="Trap Density-STS", "Stats Folder"=w3145) -> ("error out"=w3150:errorcluster, "Output Array"=w3148:string[][], "Variables"=w3142:T16)  [unwired: 2 in, 1 out]
                    n1739 = call "Origin_Export_7_27a_JW.vi"("Input Conditions"=w3142, "Analysis Array"=w3148, "error in (no error)"=w3150, "Parameter Worksheet Name"="[NSTSTable]Trap Densities", "Parameter Folder Script"="pe_cd \"N-STS\";", "Origin.IOApplication"=w3147) -> ("error out"=w3149:errorcluster, "reference out"=w3151:refnum<k7>)  [unwired: 3 in, 1 out]
                    n1740 = call <userlib>:"OAExecute.vi"("script"=w3137, "Error IO"=w3149, "Origin.IOApplication"=w3151) -> ()  [unwired: 1 in, 3 out]
                  }
                  frame #3 {
                    n1741 = local read "Opj X Axis"() -> (w3158:string)
                    n1742 = call "Param_Analysis_7_24b_JW.vi"("Independant Variable"=w3162, "error in (no error)"=w3165, "Data Folder"=w3164, "Parameter String"="Trap Density-VT (Traps/Vcm^2):", "Parameter Name"="Trap Density-Vt", "Stats Folder"=w3163) -> ("error out"=w3169:errorcluster, "Output Array"=w3167:string[][], "Variables"=w3161:T16)  [unwired: 2 in, 1 out]
                    n1743 = Concatenate Strings("window -a NVtGraph;\nlayer.x.type=", w3158, ";", "window -a NVtTable;\nwindow -s TV;") -> (w3156:string)
                    n1744 = call "Origin_Export_7_27a_JW.vi"("Input Conditions"=w3161, "Analysis Array"=w3167, "error in (no error)"=w3169, "Parameter Worksheet Name"="[NVTTable]Trap Densities", "Parameter Folder Script"="pe_cd \"N-Vt\";", "Origin.IOApplication"=w3166) -> ("error out"=w3168:errorcluster, "reference out"=w3170:refnum<k7>)  [unwired: 3 in, 1 out]
                    n1745 = call <userlib>:"OAExecute.vi"("script"=w3156, "Error IO"=w3168, "Origin.IOApplication"=w3170) -> ()  [unwired: 1 in, 3 out]
                  }
                  frame #4 {
                    n1746 = local read "Opj X Axis"() -> (w3177:string)
                    n1747 = Concatenate Strings("window -a OffIGraph;\nlayer.x.type=", w3177, ";", "window -a OffITable;\nwindow -s TV;") -> (w3175:string)
                    n1748 = call "Param_Analysis_7_24b_JW.vi"("Independant Variable"=w3181, "error in (no error)"=w3184, "Data Folder"=w3182, "Parameter String"="Off I-Sat (A):", "Parameter Name"="Off I-Sat", "Stats Folder"=w3183) -> ("error out"=w3188:errorcluster, "Output Array"=w3186:string[][], "Variables"=w3180:T16)  [unwired: 2 in, 1 out]
                    n1749 = call "Origin_Export_7_27a_JW.vi"("Input Conditions"=w3180, "Analysis Array"=w3186, "error in (no error)"=w3188, "Parameter Worksheet Name"="[OffItable]OffCurrents", "Parameter Folder Script"="pe_cd \"OffI-Sat\";", "Origin.IOApplication"=w3185) -> ("error out"=w3187:errorcluster, "reference out"=w3189:refnum<k7>)  [unwired: 3 in, 1 out]
                    n1750 = call <userlib>:"OAExecute.vi"("script"=w3175, "Error IO"=w3187, "Origin.IOApplication"=w3189) -> ()  [unwired: 1 in, 3 out]
                  }
                  frame #5 {
                    n1751 = local read "Opj X Axis"() -> (w3196:string)
                    n1752 = Concatenate Strings("window -a OnOffGraph;\nlayer.x.type=", w3196, ";", "window -a OnOffTable;\nwindow -s TV;") -> (w3194:string)
                    n1753 = call "Param_Analysis_7_24b_JW.vi"("Independant Variable"=w3200, "error in (no error)"=w3203, "Data Folder"=w3201, "Parameter String"="On/Off I-Sat:", "Parameter Name"="OnOff Ratio", "Stats Folder"=w3202) -> ("error out"=w3207:errorcluster, "Output Array"=w3205:string[][], "Variables"=w3199:T16)  [unwired: 2 in, 1 out]
                    n1754 = call "Origin_Export_7_27a_JW.vi"("Input Conditions"=w3199, "Analysis Array"=w3205, "error in (no error)"=w3207, "Parameter Worksheet Name"="[OnOffTable]On/Off Ratios", "Parameter Folder Script"="pe_cd \"OnOff-Ratio\";", "Origin.IOApplication"=w3204) -> ("error out"=w3206:errorcluster, "reference out"=w3208:refnum<k7>)  [unwired: 3 in, 1 out]
                    n1755 = call <userlib>:"OAExecute.vi"("script"=w3194, "Error IO"=w3206, "Origin.IOApplication"=w3208) -> ()  [unwired: 1 in, 3 out]
                  }
                  frame #6 {
                    n1756 = local read "Opj X Axis"() -> (w3215:string)
                    n1757 = call "Param_Analysis_7_24b_JW.vi"("Independant Variable"=w3219, "error in (no error)"=w3222, "Data Folder"=w3220, "Parameter String"="STS-Sat (V/decade):", "Parameter Name"="STS-Sat", "Stats Folder"=w3221) -> ("error out"=w3226:errorcluster, "Output Array"=w3224:string[][], "Variables"=w3218:T16)  [unwired: 2 in, 1 out]
                    n1758 = Concatenate Strings("window -a SGraph;\nlayer.x.type=", w3215, ";", "window -a STable;\nwindow -s TV;") -> (w3213:string)
                    n1759 = call "Origin_Export_7_27a_JW.vi"("Input Conditions"=w3218, "Analysis Array"=w3224, "error in (no error)"=w3226, "Parameter Worksheet Name"="[STable]Threshold Swing", "Parameter Folder Script"="pe_cd \"STS-Sat\";", "Origin.IOApplication"=w3223) -> ("error out"=w3225:errorcluster, "reference out"=w3227:refnum<k7>)  [unwired: 3 in, 1 out]
                    n1760 = call <userlib>:"OAExecute.vi"("script"=w3213, "Error IO"=w3225, "Origin.IOApplication"=w3227) -> ()  [unwired: 1 in, 3 out]
                  }
                  frame #7 {
                    n1761 = local read "Opj X Axis"() -> (w3234:string)
                    n1762 = Concatenate Strings("window -a VtGraph;\nlayer.x.type=", w3234, ";", "window -a VtTable;\nwindow -s TV;") -> (w3232:string)
                    n1763 = call "Param_Analysis_7_24b_JW.vi"("Independant Variable"=w3238, "error in (no error)"=w3243, "Data Folder"=w3241, "Parameter String"="Vt-Sat (V):", "Parameter Name"="Vt-Sat", "Stats Folder"=w3242) -> ("error out"=w3247:errorcluster, "Output Array"=w3245:string[][], "Variables"=w3237:T16)  [unwired: 2 in, 1 out]
                    n1764 = call "Origin_Export_7_27a_JW.vi"("Input Conditions"=w3237, "Analysis Array"=w3245, "error in (no error)"=w3247, "Parameter Worksheet Name"="[VtTable]Threshold Voltages", "Parameter Folder Script"="pe_cd \"Vt-Sat\";", "Origin.IOApplication"=w3244) -> ("error out"=w3246:errorcluster, "reference out"=w3248:refnum<k7>)  [unwired: 3 in, 1 out]
                    n1765 = call <userlib>:"OAExecute.vi"("script"=w3232, "Error IO"=w3246, "Origin.IOApplication"=w3248) -> ("Error IO Out"=w3239:errorcluster, "Origin.IOApplication"=w3240:refnum<k7>)  [unwired: 1 in, 1 out]
                  }
                }
                n1766 = Path To String(path=w3084) -> (string=w3083:string)
                n1767 = call <userlib>:"OAExecute.vi"("script"="pe_cd /; ", "Error IO"=w3079, "Origin.IOApplication"=w3078) -> ("Error IO Out"=w3085:errorcluster, "Origin.IOApplication"=w3086:refnum<k7>)  [unwired: 1 in, 1 out]
                n1768 = call <userlib>:"OASaveProject.vi"("path"=w3083, "Error IO"=w3085, "Origin.IOApplication"=w3086) -> ()  [unwired: 3 out]
              }
            }
          }
          event "Blank Button": Mouse Down {
            n1769 = event-data() -> ()  [unwired: 1 in, 7 out]
            n1770 = local read "Transfer File"() -> (w3263:path)
            n1771 = disable-structure shown="Disabled" {
              frame Disabled {
                n1772 = local read "Folder Index"() -> (w3264:dbl)
                n1773 = Decrement(x=w3264) -> (x-1=w3265:dbl)
                n1774 = local write "Folder Index"(w3265) -> ()
              }
              frame Enabled {
              }
            }
            n1775 = Strip Path(path=w3263) -> (stripped path=w3259:path, name=w3261:string)
            n1776 = Path To String(path=w3259) -> (string=w3258:string)
            n1777 = Concatenate Strings(w3258, "\\", "X_", w3261) -> (w3257:string)
            n1778 = String To Path(string=w3257) -> (path=w3256:path)
            n1779 = Move(source path=w3263, 10:w3256) -> ()  [unwired: 3 in, 3 out]
            n1780 = local write "Transfer File"(w3256) -> ()
          }
          event "Cancel Button": Mouse Down {
            (unwired) 6
            n1781 = event-data() -> ()  [unwired: 1 in, 7 out]
            n1782 = call "Simulate_Keyboard.vi"("Action"=2, "Virtual Key"=162) -> ()  [unwired: 7 in, 1 out]
          }
        }
        n1783 = Multiply(x=w525, y=10) -> (x*y=w527:sgl)
        n1784 = case shown="\"0\"" w566 {
          tunnel: w540 -> [w620 w626 w630 w632 w636 w638 w640 w642 w644 w646 w648 w650 w652 w654 w656 w658 w660 w662 w664 w666 w668 w670 w672 w674 w676 w678 w680 w682 w684 w686 w688 w690 w692 w694 w696 w698 w700 w702 w704 w706 w708 w710 w712 w714 w716 w718 w720 w722 w724 w726 w728 w730 w732 w734 w736 w738 w740 w742 w744 w746 w748 w750 w752 w754 w756 w758 w760 w762 w764 w766 w768 w770 w772 w774 w776 w778 w780 w782 w784 w786 w788 w790 w792 w794 w796 w798 w800 w802 w804 w806 w808 w810 w812 w814 w816 w818 w820 w822 w824 w826 w828 w830 w832 w834 w836]
          tunnel: [w620 w625 w629 w632 w636 w638 w640 w642 w644 w646 w648 w650 w652 w654 w656 w658 w660 w662 w664 w666 w668 w670 w672 w674 w676 w678 w680 w682 w684 w686 w688 w690 w692 w694 w696 w698 w700 w702 w704 w706 w708 w710 w712 w714 w716 w718 w720 w722 w724 w726 w728 w730 w732 w734 w736 w738 w740 w742 w744 w746 w748 w750 w752 w754 w756 w758 w760 w762 w764 w766 w768 w770 w772 w774 w776 w778 w780 w782 w784 w786 w788 w790 w792 w794 w796 w798 w800 w802 w804 w806 w808 w810 w812 w814 w816 w818 w820 w822 w824 w826 w828 w830 w832 w834 w836] -> w565
          tunnel: w541 -> [w622 w624 w628 w634 w635 w637 w639 w641 w643 w645 w647 w649 w651 w653 w655 w657 w659 w661 w663 w665 w667 w669 w671 w673 w675 w677 w679 w681 w683 w685 w687 w689 w691 w693 w695 w697 w699 w701 w703 w705 w707 w709 w711 w713 w715 w717 w719 w721 w723 w725 w727 w729 w731 w733 w735 w737 w739 w741 w743 w745 w747 w749 w751 w753 w755 w757 w759 w761 w763 w765 w767 w769 w771 w773 w775 w777 w779 w781 w783 w785 w787 w789 w791 w793 w795 w797 w799 w801 w803 w805 w807 w809 w811 w813 w815 w817 w819 w821 w823 w825 w827 w829 w831 w833 w835]
          tunnel: [w621 w624 w628 w633 w635 w637 w639 w641 w643 w645 w647 w649 w651 w653 w655 w657 w659 w661 w663 w665 w667 w669 w671 w673 w675 w677 w679 w681 w683 w685 w687 w689 w691 w693 w695 w697 w699 w701 w703 w705 w707 w709 w711 w713 w715 w717 w719 w721 w723 w725 w727 w729 w731 w733 w735 w737 w739 w741 w743 w745 w747 w749 w751 w753 w755 w757 w759 w761 w763 w765 w767 w769 w771 w773 w775 w777 w779 w781 w783 w785 w787 w789 w791 w793 w795 w797 w799 w801 w803 w805 w807 w809 w811 w813 w815 w817 w819 w821 w823 w825 w827 w829 w831 w833 w835] -> w564
          tunnel: w527 -> [w619 w623 w627 w631 _ _ _ _ _ _ _ _ _ _ _ _ _ _ _ _ _ _ _ _ _ _ _ _ _ _ _ _ _ _ _ _ _ _ _ _ _ _ _ _ _ _ _ _ _ _ _ _ _ _ _ _ _ _ _ _ _ _ _ _ _ _ _ _ _ _ _ _ _ _ _ _ _ _ _ _ _ _ _ _ _ _ _ _ _ _ _ _ _ _ _ _ _ _ _ _ _ _ _ _ _]
          frame "DOWN" {
            n1785 = Add(x=w622, y=w619) -> (x+y=w621:sgl)
          }
          frame "LEFT" {
            n1786 = Subtract(x=w626, y=w623) -> (x-y=w625:sgl)
          }
          frame "RIGHT" {
            n1787 = Add(x=w630, y=w627) -> (x+y=w629:sgl)
          }
          frame "UP" {
            n1788 = Subtract(x=w634, y=w631) -> (x-y=w633:sgl)
          }
          frame "ENTER (num pad)" {
          }
          frame "' (quote)" {
          }
          frame "END" {
          }
          frame "EQUALS" {
          }
          frame "ESCAPE" {
          }
          frame "GRAVE (`)" {
          }
          frame "HOME" {
          }
          frame "INSERT" {
          }
          frame "LBRACKET" {
          }
          frame "LCONTROL" {
          }
          frame "L ALT" {
          }
          frame "LSHIFT" {
          }
          frame "LWIN" {
          }
          frame "MINUS" {
          }
          frame "MULTIPLY" {
          }
          frame "NEXT" {
          }
          frame "NUMLOCK" {
          }
          frame "NUMPAD_0" {
          }
          frame "NUMPAD_1" {
          }
          frame "NUMPAD_2" {
          }
          frame "NUMPAD_3" {
          }
          frame "NUMPAD_4" {
          }
          frame "NUMPAD_5" {
          }
          frame "NUMPAD_6" {
          }
          frame "NUMPAD_7" {
          }
          frame "NUMPAD_8" {
          }
          frame "NUMPAD_9" {
          }
          frame "PAUSE" {
          }
          frame "PERIOD" {
          }
          frame "PRIOR (PG UP)" {
          }
          frame "RBRACKET" {
          }
          frame "RCONTROL" {
          }
          frame "RETURN" {
          }
          frame "R ALT" {
          }
          frame "RSHIFT" {
          }
          frame "RWIN" {
          }
          frame "SCROLL" {
          }
          frame "SEMICOLON" {
          }
          frame "SLASH" {
          }
          frame "SPACE" {
          }
          frame "SUBTRACT" {
          }
          frame "TAB" {
          }
          frame "DIVIDE" {
          }
          frame "DELETE" {
          }
          frame "DECIMAL" {
          }
          frame "COMMA" {
          }
          frame "CAPITAL" {
          }
          frame "BACKSLASH" {
          }
          frame "BACK" {
          }
          frame "ADD" {
          }
          frame "F15" {
          }
          frame "F14" {
          }
          frame "F13" {
          }
          frame "F12" {
          }
          frame "F11" {
          }
          frame "F10" {
          }
          frame "F9" {
          }
          frame "F8" {
          }
          frame "F7" {
          }
          frame "F6" {
          }
          frame "F5" {
          }
          frame "F4" {
          }
          frame "F3" {
          }
          frame "F2" {
          }
          frame "F1" {
          }
          frame "Z" {
          }
          frame "Y" {
          }
          frame "X" {
          }
          frame "W" {
          }
          frame "V" {
          }
          frame "U" {
          }
          frame "T" {
          }
          frame "S" {
          }
          frame "R" {
          }
          frame "Q" {
          }
          frame "P" {
          }
          frame "O" {
          }
          frame "N" {
          }
          frame "M" {
          }
          frame "L" {
          }
          frame "K" {
          }
          frame "J" {
          }
          frame "I" {
          }
          frame "H" {
          }
          frame "G" {
          }
          frame "F" {
          }
          frame "E" {
          }
          frame "D" {
          }
          frame "C" {
          }
          frame "B" {
          }
          frame "A" {
          }
          frame "9" {
          }
          frame "8" {
          }
          frame "7" {
          }
          frame "6" {
          }
          frame "5" {
          }
          frame "4" {
          }
          frame "3" {
          }
          frame "2" {
          }
          frame "1" {
          }
          frame "0" {
          }
        }
        n1789 = Bundle(w543, w542, w557, w556, 0.0) -> (w555:cluster{dbl, dbl, dbl, dbl, dbl})  [unwired: 1 in]
        n1790 = Bundle("X"=w565, "Y"=w564) -> (w559:cluster{"X":sgl, "Y":sgl})  [unwired: 1 in]
        n1791 = Divide(x=20, y=w526) -> (x/y=w529:sgl)
        n1792 = property on="Image Out" class="ImageControl"("Image Center Position"=w559) -> ()  [unwired: 2 in, 2 out]
        n1793 = call "IMAQ Convert Rectangle to ROI (Polygon)"("Rectangle"=w555) -> ("ROI Descriptor"=w553:T3)  [unwired: 7 in, 2 out]
        n1794 = Bundle("Application Font", w529, w533, w533, w533, w533, w533, TRUE, w531) -> (w535:T17)  [unwired: 1 in]
        n1795 = property on="Image Out 2" class="ImageControl"("ROI"=w553) -> ()  [unwired: 2 in, 2 out]
        n1796 = Bundle(w531, w535, w531, w531) -> (w534:T18)  [unwired: 1 in]
        n1797 = property on="Image Out" class="ImageControl"() -> ("ROI"=w518:T10)  [unwired: 2 in, 2 out]
        n1798 = Unbundle By Name(w518) -> ("Contours"=w582:T14)
        n1799 = local read "Image Out"() -> (w537:T2)
        n1800 = call "IMAQ Clear Overlay"("Image"=w537) -> ("Image Out"=w536:T2)  [unwired: 9 in, 1 out]
        n1801 = Initialize Array(0) -> (w580:i32[])  [unwired: 1 in]
        n1802 = local read "Magnification"() -> (w571:u16)
        n1803 = Array Size(array=w582) -> (size(s)=w581:i32)
        n1804 = Build Array(0.505025, 0.252522, 0.127742, 0.050345, 0.031129) -> (w572:dbl[])
        n1805 = Array Subset(array=w572, index=w571, length=1) -> (w569:dbl[])
        n1806 = property on="Image Out" class="ImageControl"() -> ("ZoomInteger"=w561:cluster{"X":i32, "Y":i32})  [unwired: 2 in, 2 out]
        n1807 = To Double Precision Float(number=w569) -> (double precision float=w568:dbl[])
        n1808 = for {
          N: w581 -> [_]
          shift-right: [w859] -> _
          shift-left: w582 -> [w859]
          shift-right: [w857] -> w567
          shift-left: w580 -> [w856]
          tunnel: w568 -> [w855]
          shift-right: [w852] -> _
          shift-left: w536 -> [w854]
          tunnel: w534 -> [w847]
          i -> [w851]
          n1809 = Index Array(array=w859, index=w851) -> (element=w868:T19)
          n1810 = Unbundle(w868) -> ("Points"=w867:i32[])  [unwired: 2 out]
          n1811 = Array To Cluster(array=w867) -> (cluster=w866:T20)
          n1812 = Unbundle(w866) -> ("Points[0]"=w846:i32, "Points[1]"=w843:i32, "Points[2]"=w858:i32, "Points[3]"=w864:i32)  [unwired: 5 out]
          n1813 = Add(x=w846, y=10) -> (x+y=w844:i32)
          n1814 = Subtract(x=w843, y=w864) -> (x-y=w863:i32)
          n1815 = Subtract(x=w846, y=w858) -> (x-y=w865:i32)
          n1816 = Square(x=w863) -> (x^2=w861:i32)
          n1817 = Square(x=w865) -> (x^2=w862:i32)
          n1818 = Add(x=w862, y=w861) -> (x+y=w860:i32)
          n1819 = Square Root(x=w860) -> (sqrt(x)=w837:dbl)
          n1820 = Multiply(x=w837, y=0.5) -> (x*y=w840:dbl)
          n1821 = Add(x=w840, y=w843) -> (x+y=w842:dbl)
          n1822 = Bundle(w844, w842) -> (w853:cluster{i32, dbl})  [unwired: 1 in]
          n1823 = Multiply(x=w837, y=w855) -> (x*y=w850:dbl[])
          n1824 = Index Array(array=w850) -> (element=w849:dbl)  [unwired: 1 in]
          n1825 = Number To Fractional String(number=w849) -> (F-format string=w848:string)  [unwired: 3 in]
          n1826 = call "IMAQ Overlay Text"("BG Color (Transparent)"=u32 0, "Text Color (black)"=u32 16448250, "Font, Size & Style"=w847, "String"=w848, "Origin"=w853, "Image"=w854) -> ("Image Out"=w852:T2)  [unwired: 4 in, 1 out]
          n1827 = Build Array (concatenate)(w856, w850) -> (w857:dbl[])
          n1828 = local write "Numeric 3"(w837) -> ()
        }
        n1829 = local write "ROI Descriptor"(w518) -> ()
        n1830 = Unbundle(w561) -> ("X"=w560:i32)  [unwired: 1 out]
        n1831 = Add Array Elements(numeric array=w567) -> (sum=w578:dbl)
        n1832 = local write "Distances"(w567) -> ()
        n1833 = local write "Total Width"(w578) -> ()
        n1834 = local write "Zoom"(w560) -> ()
        n1835 = local read "Manual-Width"() -> (w517:bool)
        n1836 = local read "Total Width"() -> (w521:dbl)
        n1837 = local read "Rec: Width"() -> (w519:dbl)
        n1838 = Not(x=w517) -> (.not. x?=w515:bool)
        n1839 = Equal To 0?(x=w521) -> (x = 0?=w516:bool)
        n1840 = Or(x=w516, y=w517) -> (x .or. y?=w520:bool)
        n1841 = And(x=w516, y=w515) -> (x .and. y?=w514:bool)
        n1842 = case shown="True" w514 {
          tunnel: w519 -> [_ w597]
          frame False {
          }
          frame True {
            n1843 = local write "New: Width"(w597) -> ()
          }
        }
        n1844 = case shown="False" w520 {
          tunnel: w521 -> [w598 _]
          frame False {
            n1845 = local write "New: Width"(w598) -> ()
          }
          frame True {
          }
        }
        n1846 = local read "Manuel-Dielectric"() -> (w443:bool)
        n1847 = local read "Rec: Dielectric (d)"() -> (w442:dbl)
        n1848 = local read "Manuel-Length"() -> (w444:bool)
        n1849 = local read "Manual-Temp"() -> (w416:bool)
        n1850 = local read "Rec: Length"() -> (w445:dbl)
        n1851 = local read "Rec: Temp"() -> (w417:dbl)
        n1852 = case shown="False" w444 {
          tunnel: w445 -> [w588 _]
          frame False {
            n1853 = local write "New: Length"(w588) -> ()
          }
          frame True {
          }
        }
        n1854 = case shown="False" w443 {
          tunnel: w442 -> [w587 _]
          frame False {
            n1855 = local write "New: Dielectric"(w587) -> ()
          }
          frame True {
          }
        }
        n1856 = case shown="False" w416 {
          tunnel: w417 -> [w584 _]
          frame False {
            n1857 = local write "New: Temp"(w584) -> ()
          }
          frame True {
          }
        }
      }
    }
  }
  n1858 = Build Array("DeviceID", "Fabricator", "Deposition", "Date", "Sample", "Row", "Column", "L (um)", "W (um)", "Material", "Treatment", "TC (mM)", "Solvent", "C (%)", "ST (C)", "Drops", "Wait (s)", "RT (F)", "RH (%)", "Ramp (s)", "RPM", "Accel (RPM/s)", "Time (s)", "Mobility", "On/Off", "Vt", "S.T.S") -> (→"Transformer \nHeaders":string[])
